vi "SentinelController v36.vi"() -> ()   [LabVIEW 2011]
uses:
  SC MT99XX tester states.ctl
  SC handler states.ctl
  Handler Types.ctl
  SC NS6040 tester states v2.ctl
  Echo tester states.ctl
  <vilib>/Instr/_visa.llb/Select Event Type.ctl
  <userlib>/configTool/configTool.llb/initConfigGlobal.vi
  <userlib>/configTool/configTool.llb/loadConfigFile.vi
  <userlib>/configTool/configTool.llb/closeConfig.vi
  <userlib>/configTool/configTool.llb/getProperty(DBL).vi
  <userlib>/configTool/configTool.llb/getProperty(U32).vi
  <userlib>/configTool/configTool.llb/getProperty(BOOL).vi
  <userlib>/configTool/configTool.llb/getProperty(I32).vi
  <userlib>/configTool/configTool.llb/getProperty(STR).vi
panel:
  out "Numeric 5":i32
  out "Numeric 4":i32
  out "Numeric 3":i32
  out "Numeric 2":i32
  out "Numeric":i32
  out "H2 wt start hidden":u32
  out "H2 wt end hidden":u32
  out "H2 it start hidden":u32
  out "H2 it end hidden":u32
  out "H2 tt start hidden":u32
  out "H2 tt end hidden":u32
  in  "Data log path and filename":path=path "configuraitons/default_configuraiton.cfg"
  in  "Panels":T1(tab)=enum."System Configuration"
  in  "Test cell ID":string="default"
  in  "Operator name":string="default"
  in  "Lot number":string="default"
  in  "Configuration file path and filename":path
  in  "POWER":bool=TRUE
  in  "Tester Handler Config":T2=enum."Seiko-Epson NS6040" caption="Handler type"
  in  "H1 handler type":T2=enum."Seiko-Epson NS6040" caption="Handler type"
  in  "H2 handler type":T2=enum."Seiko-Epson NS6040" caption="Handler type"
  in  "H2 allow lower parallelism":bool
  in  "H1 allow lower parallelism":bool
  in  "H1 low yield warning":dbl=95.0 min=0.0 max=100.0 step=1.0
  in  "Ignore alarms until AFTER this many cycles":i32=20
  in  "H1 low yield alarm":dbl=85.0 min=0.0 max=100.0 step=1.0
  in  "H1 low UPH warning (%)":dbl=95.0 min=1.0 max=48000.0 step=1.0
  in  "H1 low UPH alarm (%)":dbl=90.0 min=1.0 max=48000.0 step=1.0
  in  "Enable data logging of all events":bool=TRUE
  in  "Enable electronic notification of alarms":bool
  in  "H2 low UPH alarm (%)":dbl=90.0 min=1.0 max=48000.0 step=1.0
  in  "H2 low UPH warning (%)":dbl=95.0 min=1.0 max=48000.0 step=1.0
  in  "H2 low yield alarm":dbl=90.0 min=0.0 max=100.0 step=1.0
  in  "H2  low yield warning":dbl=95.0 min=0.0 max=100.0 step=1.0
  in  "H1 enable halt\non yield alarm":bool
  in  "H2 enable halt\non yield alarm":bool
  in  "H1 enable halt\non UPH alarm":bool
  in  "H2 enable halt\non UPH alarm":bool
  out "H2 Device Count":u32 caption="Device Count"
  out "H1 Device Count":u32 caption="Decvice Count"
  out "H1 Good Units":u32 caption="Decvice Count"
  out "H2 Good Units":u32 caption="Device Count"
  out "H1 lot yield mon":dbl format="%.1f"
  out "H2 lot yield mon":dbl format="%.1f"
  out "UPH averaging":u32=20 min=2 max=100 step=1
  out "Yield averaging":u32=20 min=2 max=100 step=1
  in  "Push to reset charts":bool
  in  "Run":bool caption="Run / Stop"
  in  "Optimize handler speed":bool
  out "H1 parallelism":u32
  out "Utilization averaging":i32=6 min=2 max=20 step=1
  out "H2 nominal 2":bool=TRUE
  out "H2 warning 2":bool
  out "H2 alarm 2":bool
  out "H1 nominal 2":bool=TRUE
  out "H1 warning 2":bool
  out "H1 alarm 2":bool
  out "H2 nominal":bool=TRUE
  out "H2 warning":bool
  out "H2 alarm":bool
  out "H1 nominal":bool=TRUE
  out "H1 warning":bool
  out "H1 alarm":bool
  out "H2 Lock":bool
  out "H1 Lock":bool
  out "H2 measured Test Time":dbl caption="Index Time" format="%.2f"
  out "H2 measured  Index Time":dbl caption="Index Time" format="%.2f"
  out "H2 Indexing":bool
  out "H2 Testing":bool
  out "H2 Waiting":bool
  out "H2 On/Off-line":bool
  out "H2 measured Wait Time":dbl caption="Index Time" format="%.2f"
  out "H1 measured Test Time":dbl caption="Index Time" format="%.2f"
  out "H1 measured Index Time":dbl caption="Index Time" format="%.2f"
  out "H1 Indexing":bool
  out "H1 Testing":bool
  out "H1 Waiting":bool
  out "H1 On/Off-line":bool
  out "H1 measured Wait Time":dbl caption="Index Time" format="%.2f"
  out "System UPH":u32(knob) caption="Sys UPH" scale=0.0..30240.0 scale format="%#.0f"
  out "H2 UPH":cluster{u32, u32}(knob) scale=0.0..14400.0 scale format="%#.0f"
  out "H1 UPH":cluster{u32, u32}(knob) scale=0.0..14400.0 scale format="%#.0f"
  out "Sys utilization":dbl(knob) caption="Yield" scale=0.0..100.0
  in  "H2 online":bool=TRUE
  in  "H1 online":bool=TRUE
  in  "Tester online":bool=TRUE
  in  "Alert volume":u32(knob)=5 max=10 step=1 scale=0.0..10.0
  in  "Audio On / Off":bool
  out "SysUtilMon":cluster{i32, i32}(graph)
  out "H2 parallelism":u32 caption="H2 Paralellism"
  out "YieldMon":cluster{i32, i32, i32, i32}(graph)
  out "Program Parallelism":u32=8 caption="Tester Parallelism" min=1 max=16 step=1
  out "H2 calc UPH":dbl format="%#.0f"
  out "H1 Index Time 2":dbl caption="H1 index time"
  out "H1 Test Time 2":dbl caption="H1 test time"
  out "H1 P in formula":u32 caption="H1 Parallelism"
  out "H2 UPH per unit area":dbl format="%.1f"
  out "H1 calc UPH":dbl format="%#.0f"
  out "H1 UPH per unit area":dbl format="%.1f"
  out "Std mo cost ($/mo)":dbl
  out "Std unit cost\n(cents/device)":dbl format="%.3g"
  out "UPH":dbl format="%#.0f"
  in  "Hours per month":i32=730
  out "Std hourly\ncost ($/hr)":dbl format="%.2f"
  in  "Std cell \nfloorspace area":i32=200 min=10 max=1000 step=10
  in  "Overhead ($/mo)":dbl=1000.0 min=0.0 max=10000.0 step=100.0
  in  "Handler cost ($/mo)":dbl=2500.0 min=0.0 max=100000.0 step=100.0
  in  "Tester cost ($/mo)":dbl=8500.0 min=0.0 max=100000.0 step=500.0
  in  "Utilization (%)":u32=80 min=10 max=100 step=10
  out "Calendar days required\nfor testing all units":dbl format="%.1f"
  in  "# of devices to test":u32=10000000 min=1000 max=100000000 step=1000
  out "$ saved":i64 format="%#.0f"
  out "H2 IT (scycle)":dbl format="%.2f"
  out "H2 TT (s/cycle)":dbl format="%.2f"
  out "H2 WT (s/cycle)":dbl format="%.2f"
  out "H1 WT (s/cycle)":dbl format="%.2f"
  out "H1 IT (s/cycle)":dbl format="%.2f"
  out "H1 TT (s/cycle)":dbl format="%.2f"
  out "H2 units/cycle":u32 caption="H1 Parallelism"
  out "H1 units/cycle":u32
  out "Calc H1 UPH":u32
  out "Calc H2 UPH":u32
  out "Std cell floorspace area":i32
  out "Tandem unit cost\n(cents/device)":dbl format="%.3f"
  out "Hours per month 2":i32 caption="Hours per month"
  out "Total Mo Costs ($/mo) 3":dbl caption="Tandem mo cost ($/mo)"
  out "Total Mo Costs ($/mo) 2":dbl caption="Std mo cost ($/mo)"
  out "Calc\nsystem UPH":u32 caption="Simulated\nSystem UPH"
  out "Tandem\nfloorspace area":i32
  out "Tandem UPH\nper unit area":dbl format="%.1f"
  in  "Second handler cost ($/mo)":dbl=2500.0 min=0.0 max=10000.0 step=100.0
  out "Tandem hourly\ncost ($/hr)":dbl format="%.2f"
  in  "Celerint licensing cost ($/mo)":dbl=1000.0 min=0.0 max=10000.0 step=100.0
  in  "Celerint hardware cost ($/mo)":dbl min=0.0 max=10000.0 step=1.0
  in  "Additional floorspace\nfor second handler":i32=50 min=0 max=1000 step=10
  out "Number of text alerts":u32 caption="Number of alerts\nsent as notifications"
  in  "Enable text notification":bool
  out "Notifications Lot Display":string="default" caption="Lot number (not editable)"
  in  "Include\ndata log as\nattachment":bool=TRUE
  out "Number of email alerts":u32 caption="Number of alerts\nsent as notifications"
  out "Email alert - attachment (not editable)":path
  in  "Email alert - message":string="An alarm event has ocurred on a semiconductor test lot that you have requested to monitor.  Please see the attached data log for event details.\n\nThis message is generated automatically by the Sentinel Controller program.\n\nTo stop these messages, please contact the test floor operator and disable automatic alert notifictions.\n\n"
  in  "Email alert - engineer":string="harry@celerint.com"
  in  "Email alert - CC":string="hjr@celerint.com"
  in  "Enable email notification":bool
  in  "Carrier":enum16{"T-Mobile", "AT&T", "Verizon", "Sprint"}(ring)=enum."AT&T"
  in  "Phone number":string="5128263411"
  in  "Subject":string="From: Sentinel Controller"
  in  "Body":string="An alarm event has ocurred"
  in  "GPIB wait time (ms)":u32=1000
  in  "Slow for  Diagnostics":bool=TRUE
  out "GPIB bus 0 read error":bool
  out "GPIB Bus 0 traffic":string
  out "GPIB bus 1 traffic":string
  out "GPIB bus 2 traffic":string
  out "GPIB bus 0 write error":bool
  out "GPIB bus 1 read error":bool
  out "GPIB bus 1 write error":bool
  out "GPIB bus 2 write error":bool
  out "GPIB bus 2 read error":bool
  out "VISA bus 1 open error":bool
  out "VISA bus 2 open error":bool
  out "VISA bus 0 open error":bool
  out "VISA bus 0 close error":bool
  out "VISA bus 1 close error":bool
  out "VISA bus 2 close error":bool
  out "Decrease Handler Velocity":string
  out "Increase Handler Velocity":string
  out "Get Handler Velocity":string
  in  "SentCtrl listens to tester at":refnum<visa-resource-name>="GPIB0::INTFC"
  out "H2 Address":string
  out "H1 Address":string
  out "Tester address":string
  in  "SentCtrl talks to tester at":refnum<visa-resource-name>="GPIB0::0::INSTR"
  in  "SentCtrl listens to handler 1 at":refnum<visa-resource-name>="GPIB1::INTFC"
  in  "SentCtrl talks to handler 1 at":refnum<visa-resource-name>="GPIB1::1::INSTR"
  in  "SentCtrl listens to handler 2 at":refnum<visa-resource-name>="GPIB2::INTFC"
  in  "SentCtrl talks to handler 2 at":refnum<visa-resource-name>="GPIB2::1::INSTR"
  in  "Ni Logo":bool
  in  "Ni Logo 2":bool
  out "H2 Ready with sites hid":bool
  in  "Echo state of tester hid":T3
  in  "SRQ MASK from tester hid":string
  in  "H1 binning string hid":string
  in  "H2 binning string hid":string
  in  "H1 FULLSITES? response hid":string
  in  "H2 FULLSITES? response hid":string
  in  "H1 FULLSITES? binary hid":string
  in  "H2 FULLSITES? binary hid":string
  in  "H1 response to SPOLL hid":string
  in  "H2 response to SPOLL hid":string
  in  "H1 response to FR? hid":string
  in  "H2 response to FR? hid":string
  in  "NS6040 tester states H1 hid":T4
  in  "NS6040 tester states H2 hid":T4
  in  "MT99XX tester states H2 hid":T5
  in  "MT99XX tester states H1 hid":T5
  in  "GPIB parsed msg from tester hid":string
  in  "Message from H2 hid":string
  in  "Message from H1 hid":string
  in  "Message from tester hid":string
  in  "H1 response to *IDN? hid":string
  in  "H2 response to *IDN? hid":string
  in  "GPIB wait timeout hid":u32
  out "Number of data log entries hid":u32
  in  "Last locked handler hid":enum16{"H1", "H2"}(ring)
  out "SC measured wait time hid":dbl
  out "Exit SC tester H2 StMach hid":bool
  out "Exit SC tester H1 StMach hid":bool
  out "Exit SC handler StMach hid":bool
  out "H2 response to *HAND? hid":string
  out "H1 response to *HAND? hid":string
  in  "Tester loop counter hid":u32
  in  "H2 loop counter hid":u32
  in  "H1 loop counter hid":u32
  in  "Test Cycle State hid":T6(ring)
  in  "Test time expected hid":dbl
  out "H1 it end hidden":u32
  out "H1 wt start hidden":u32
  out "H1 tt start hidden":u32
  out "H1 wt end hidden":u32
  out "H1 tt end hidden":u32
  out "H1 it start hidden":u32
  in  "H1 SITES? response hid":string
  out "VISA bus 1 resource name out hid":refnum<visa-resource-name>
  out "VISA bus 1 error out hid":errorcluster
  out "VISA bus 2 error out hid":errorcluster
  out "VISA bus 2 resource name out hid":refnum<visa-resource-name>
  out "VISA bus 0 error out hid":errorcluster
  out "tester wt start hid":u32
  out "tester wt end hid":u32
  out "tester tt start hid":u32
  out "tester tt end hid":u32
  out "SC measured test time hid":dbl
  in  "Binning string from tester hid":string
  out "VISA bus 0 resource name out hid":refnum<visa-resource-name>
  in  "SC handler states hid":T7
  out "H1 Single Handler UPH hid":dbl
  out "H1 UPH warning limit hid":dbl
  out "H1 UPH alarm limit hid":dbl
  out "H2 Single Handler UPH hid":dbl
  out "H2 UPH warning limit hid":dbl
  out "H2 UPH alarm limit hid":dbl
  in  "Min Test Time hid":dbl=0.499 caption="Min Test Time" min=0.1 max=1.0 step=0.1 format="%#.1g"
  in  "H2 index time expected hid":dbl
  in  "H1 index time expected hid":dbl
  in  "system states hid":T8(ring)
  in  "system statuts hid":T9(ring)
  out "H1 cycle yield hid":dbl format="%.1f"
  out "H2 cycle yield hid":dbl format="%.1f"
  in  "H2 SITES? response hid":string
  out "H1 Ready with sites hid":bool
  # "Sentinel Controller\nfor\nTandlem Handler\nTest Cells \nwww.celerint.com"
  # "Turning off POWER will stop execution the Sentinel Controller Program"
  # "INPUT FILE"
  # "LOT INFORMATION"
  # "Celerint Sentinel Controller"
  # "SYSTEM SETTINGS"
  # "Tester Handler Config"
  # "Handler  1"
  # "Handler 2"
  # "Set UPH thresholds as % of max UPH"
  # "Set UPH thresholds as % of max UPH"
  # "test cycles (insertions)"
  # "Celerint Sentinel Controller"
  # "Handler 2"
  # "Handler 1"
  # "Yield"
  # "UPH"
  # "Yield"
  # "UPH"
  # "parallelism"
  # "lot yield (%)"
  # "good devices"
  # "devices tested"
  # "Data"
  # "Avg"
  # "wait time"
  # "index time"
  # "test time"
  # "waiting"
  # "H1"
  # "H2"
  # "testing"
  # "indexing"
  # "on/off-line"
  # "STANDARD SETUP"
  # "H2 calculated\nsimilarly"
  # "3600"
  # "Celerint Sentinel\nController Simulator"
  # "TANDEM HANDLER SETUP"
  # "SAVINGS"
  # "3600 (s/hr)"
  # "3600 (s/hr)"
  # "Celerint Sentinel Controller"
  # "Lot number will be appended automatically:"
  # "This data is read from the INI file (.cfg)\nat program start and is used to configure\nthe various GPIB interfaces on the Sentinel\nController."
  # "These setting are created based on the addresses read from the INI file."
  # "Laptop Tester Sim\nGPIB0,SC\naddress 0\nlisten at: GPIB0::INTFC\ntalk to: GPIB0::1::INSTR"
  # "*SITES?"
  # "binning"
  # "Bus 0"
  # "1011"
  # "SC\nGPIB0,Non-SC\naddress 1\nlisten at: GPIB0::INTFC\ntalk to: GPIB0::0::INSTR"
  # "SC\nGPIB1,SC\naddress 0\nlisten at: GPIB1::INTFC\ntalk to: GPIB1::0::INSTR"
  # "SC\nGPIB2,SC\naddress 0\nlisten at: GPIB2::INTFC\ntalk to: GPIB2::0::INSTR"
  # "NI PXI-1031"
  # "*SITES?"
  # "binning"
  # "*SITES?"
  # "binning"
  # "Bus 1"
  # "Bus 2"
  # "1011"
  # "1011"
  # "Laptop H1 Sim\nGPIB1,Non-SC\naddress 1\nlisten at: GPIB1::INTFC\ntalk to: GPIB1::0::INSTR"
  # "Laptop H2 Sim\nGPIB2,Non-SC\naddress 1\nlisten at: GPIB2::INTFC\ntalk to: GPIB2::0::INSTR"
  # "Note:\nUsually, there are default GPIB addresses used for the tester and handler.\nThese addresses are read in from the INI file (.cfrg extension) when this\nprogram initializes.  For the purposes of this map, we are using  these defaults:\n          - Semiconductor tester default GPIB address: 6\n          - Semiconductor handler default GPIB address: 14\nFor the purposes of this illustration, these addresses are purely arbitrary."
  # "Tester\nGPIB0,SC\naddress 6\nlisten at: GPIB0::INTFC\ntalk to: GPIB0:14::INSTR"
  # "*SITES?"
  # "binning"
  # "Bus 0"
  # "1011"
  # "SC\nGPIB0,Non-SC\naddress 14\nlisten at: GPIB1::INTFC\ntalk to: GPIB1:6::INSTR"
  # "SC\nGPIB1,SC\naddress 6\nlisten at: GPIB1::INTFC\ntalk to: GPIB1:14::INSTR"
  # "SC\nGPIB2,SC\naddress 6\nlisten at: GPIB2::INTFC\ntalk to: GPIB2:14::INSTR"
  # "NI PXI-1031"
  # "*SITES?"
  # "binning"
  # "*SITES?"
  # "binning"
  # "Bus 1"
  # "Bus 2"
  # "1011"
  # "1011"
  # "Handler 1\nGPIB0,Non-SC\naddress 14\nlisten at: GPIB0::INTFC\ntalk to: GPIB0:6::INSTR"
  # "Handler 2\nGPIB0,Non-SC\naddress 14\nlisten at: GPIB0::INTFC\ntalk to: GPIB0:6::INSTR"
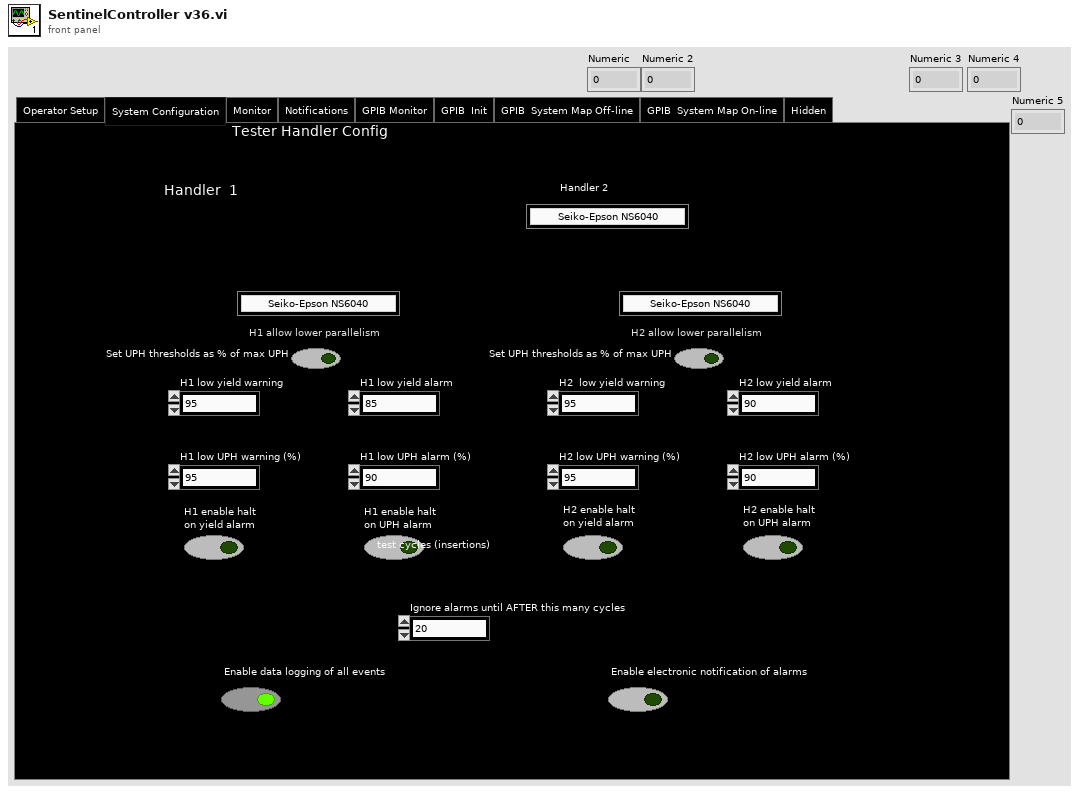
[diagram p1: front panel]
types:
  T1 = enum32{"Operator Setup", "System Configuration", "Monitor", "Benefit Analysis", "Notifications", "GPIB Monitor", "GPIB  Init", "GPIB  System Map Off-line", "GPIB  System Map On-line", "Hidden"}
  T2 = typedef "Handler Types.ctl" = enum16{"Multitest", "Seiko-Epson NS6040"}
  T3 = typedef "Echo tester states.ctl" = enum16{"ECHONG", "ECHOOK", "NO ECHO"}
  T4 = typedef "SC NS6040 tester states v2.ctl" = enum16{"initializing bus", "sending *IDN?", "serial polling handler", "sending Fullsites?", "testing", "binning", "closing bus"}
  T5 = typedef "SC MT99XX tester states.ctl" = enum16{"initializing bus", "polling *SITES?", "sending *IDN?", "testing", "binning", "closing bus"}
  T6 = enum16{"idled", "SOT received", "SOT sent", "binning sent", "binning received", "sites ready received", "sites ready sent"}
  T7 = typedef "SC handler states.ctl" = enum16{"initializing bus", "waiting on event", "waiting on serial poll", "reading", "responding to *IDN?", "responding to Fullsites?", "responding to SITES?", "responding to HIDN?", "respond to HAND?", "testing", "responding to BINON", "responding to A BIN", "ECHONG", "ECHOOK", "responding to unknown command", "closing bus"}
  T8 = enum16{"H1 Ready", "H2 Ready", "No Handler Ready"}
  T9 = enum16{"H1NH2N", "H1NH2W", "H1NH2A", "H1WH2N", "H1WH2W", "H1WH2A", "H1AH2N", "H1AH2W", "H1AH2A"}
  T10 = enum16{"open", "replace", "create", "open or create", "replace or create", "replace or create with confirmation"}
  T11 = typedef "configRef.ctl" = refnum<vi>
  T12 = cluster{i32, "rolling avg out":dbl, "H1 low yield alarm":dbl, "H2 low yield alarm":dbl}
  T13 = cluster{"rolling avg out":dbl, i32, "H1 low yield alarm":dbl, "H2 low yield alarm":dbl}
  T14 = typedef "Select Event Type.ctl" = u32
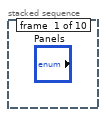
[diagram p2: hidden frame]
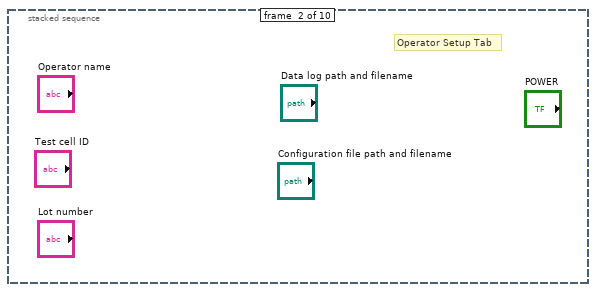
[diagram p3: hidden frame]
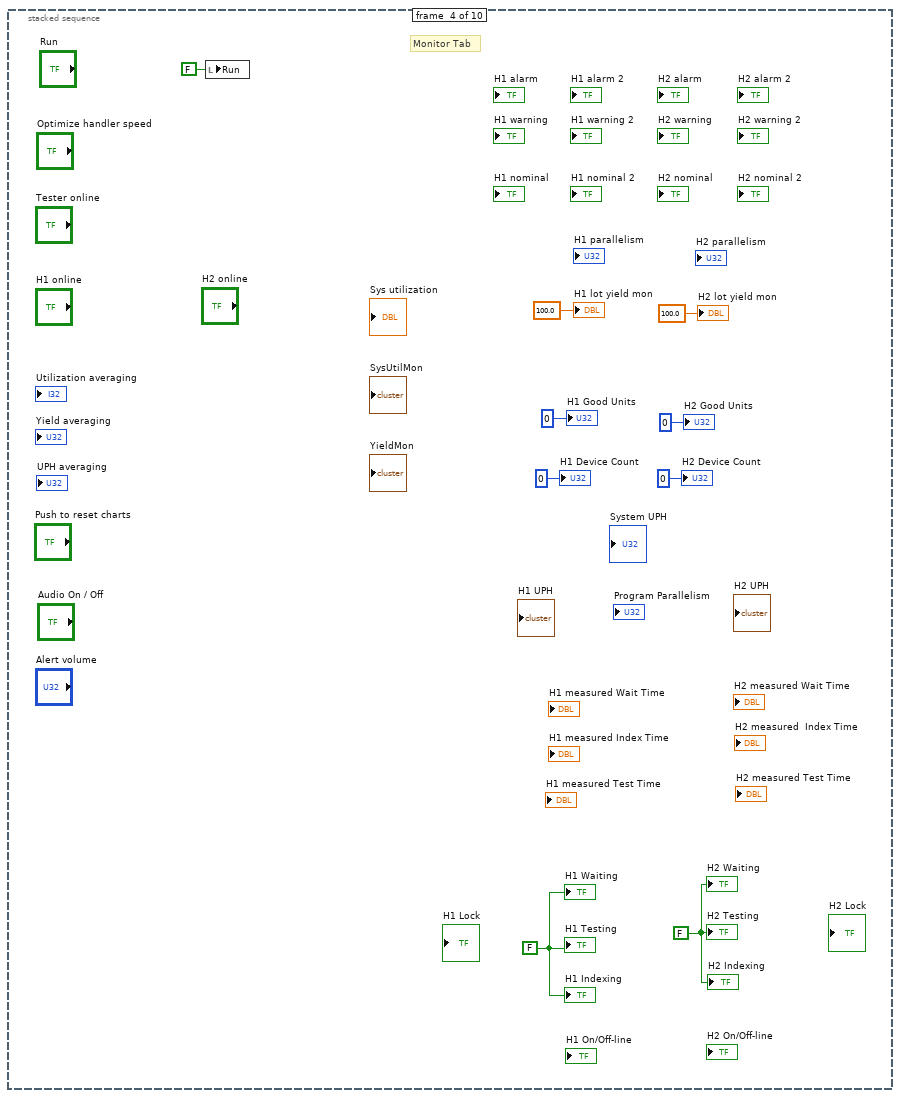
[diagram p4: hidden frame]
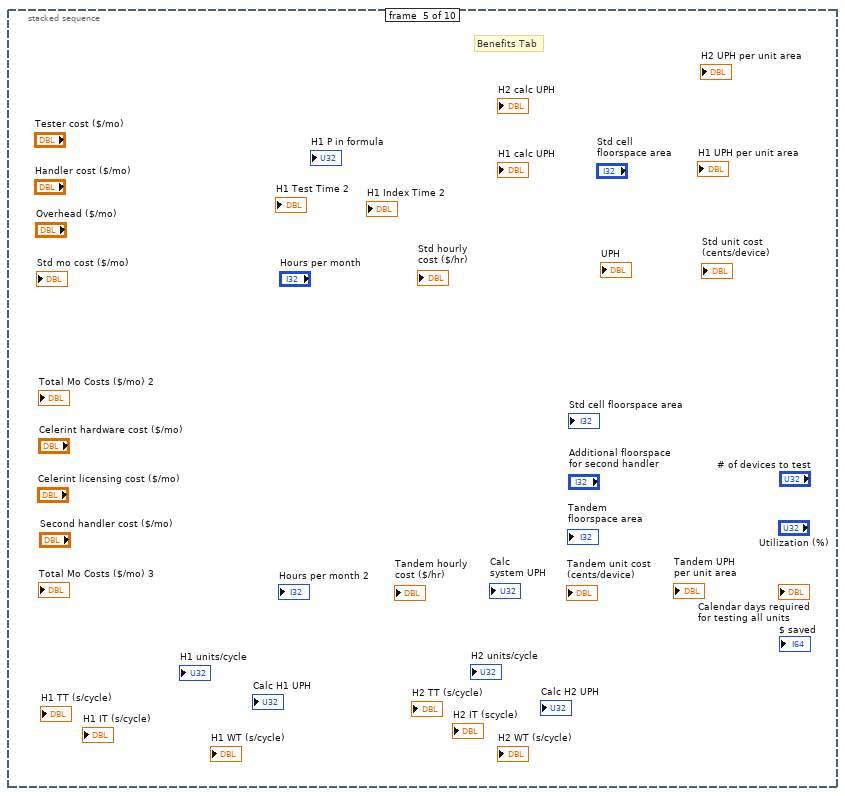
[diagram p5: hidden frame]
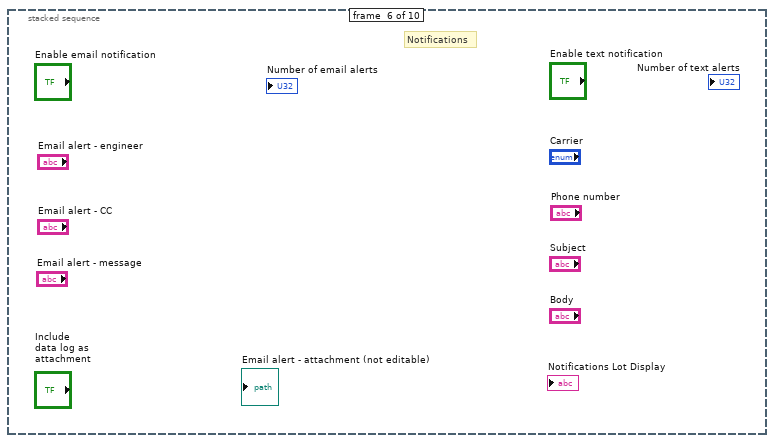
[diagram p6: hidden frame]
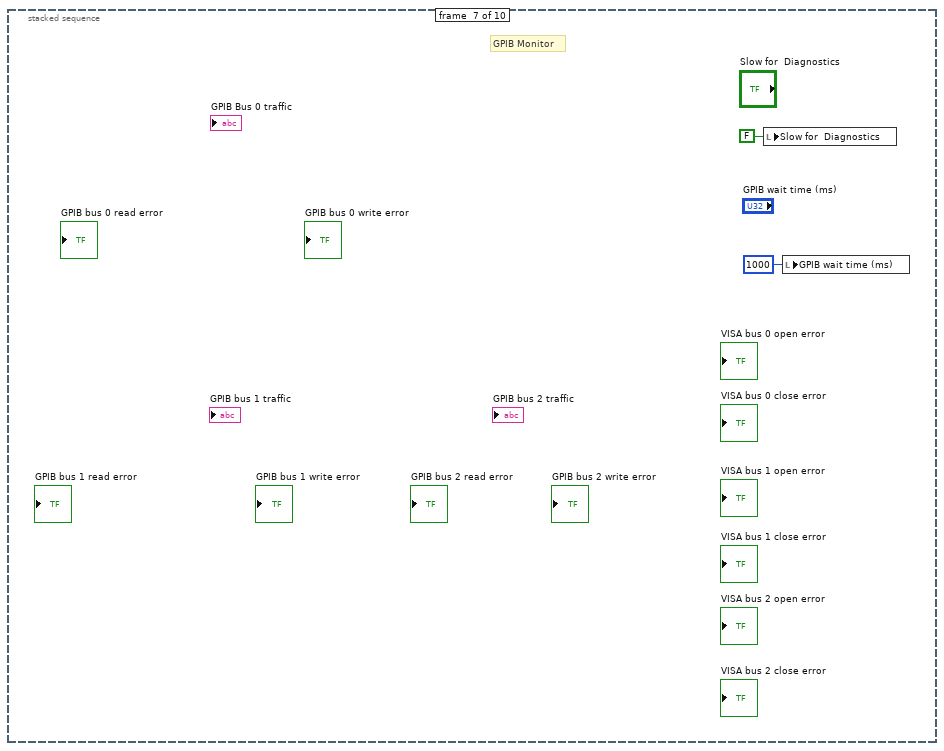
[diagram p7: hidden frame]
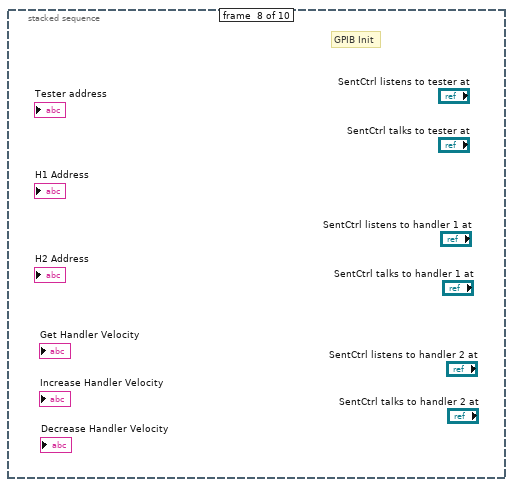
[diagram p8: hidden frame]
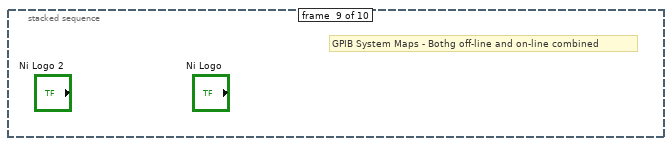
[diagram p9: hidden frame]
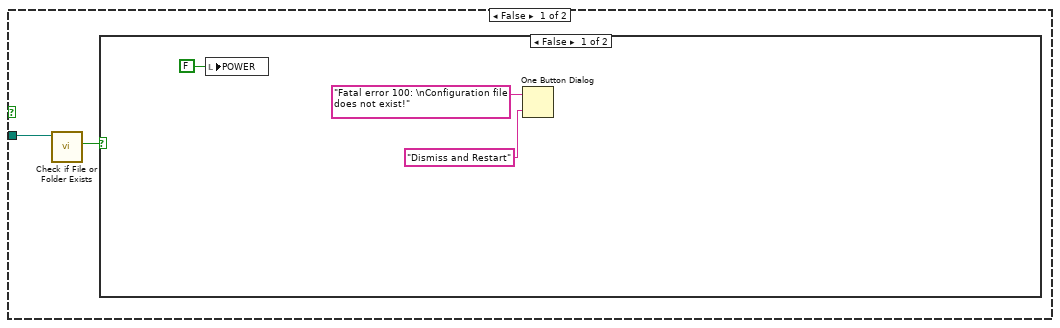
[diagram p11: hidden frame]
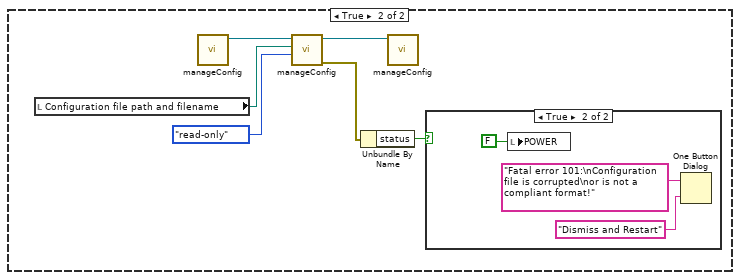
[diagram p12: hidden frame]
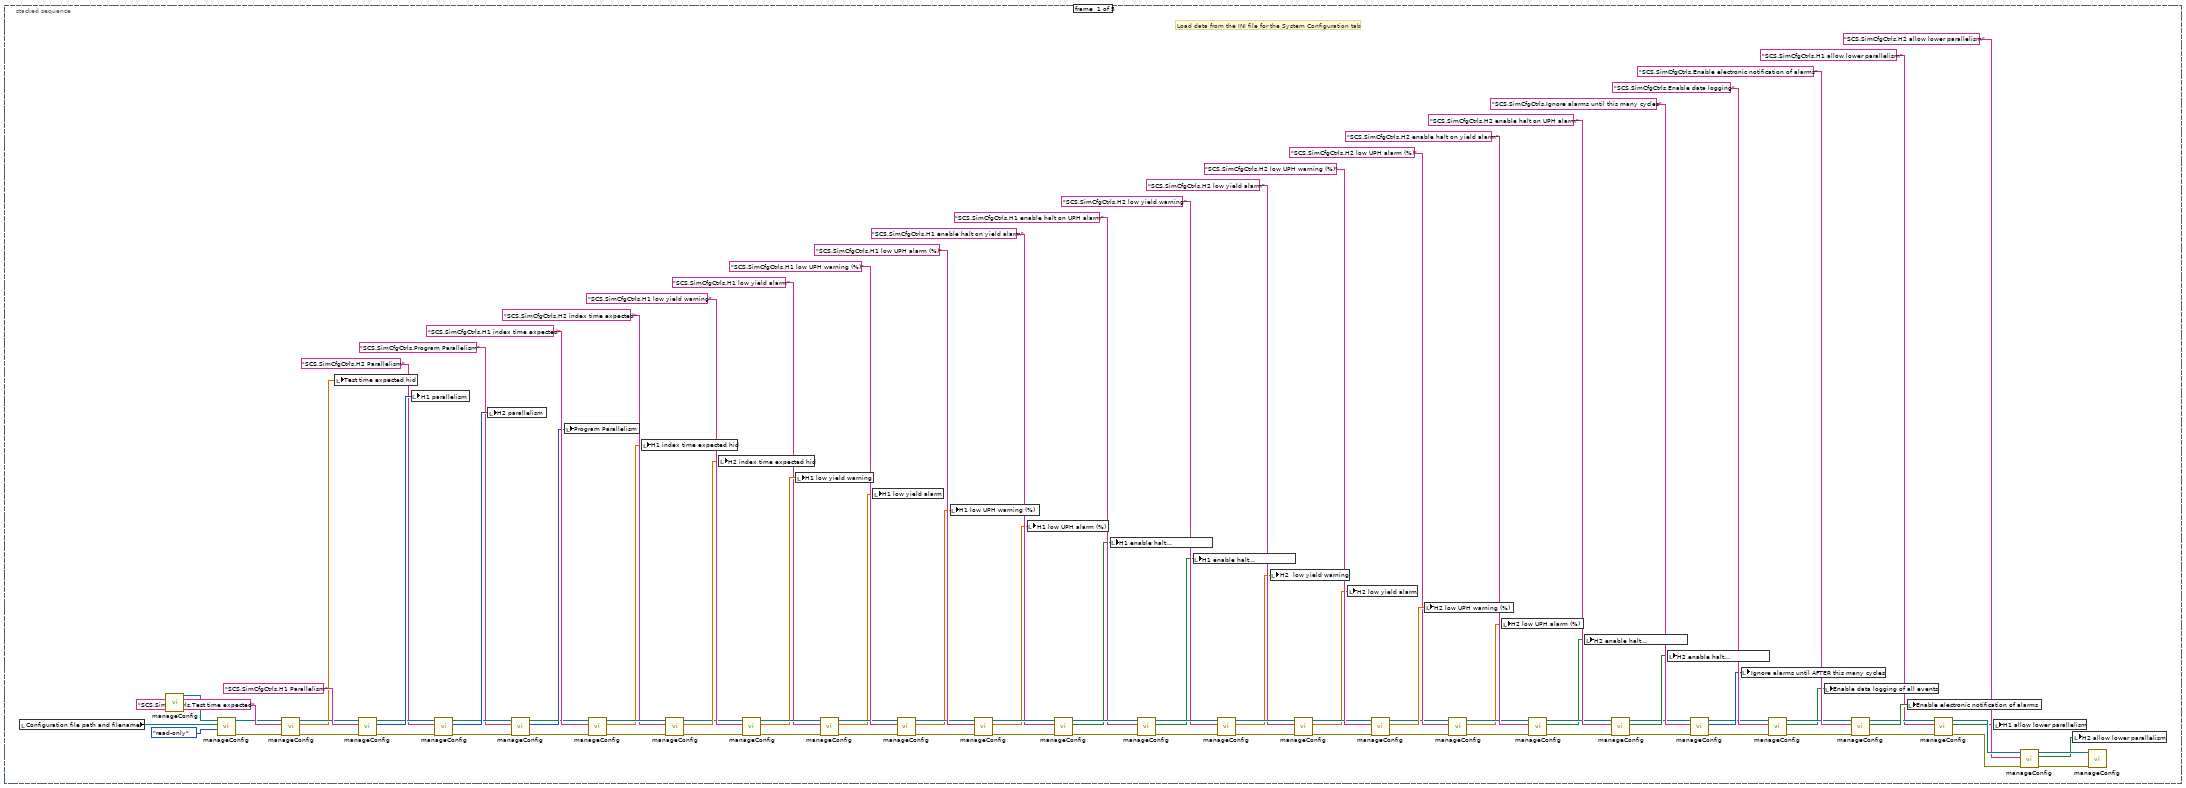
[diagram p15: hidden frame]
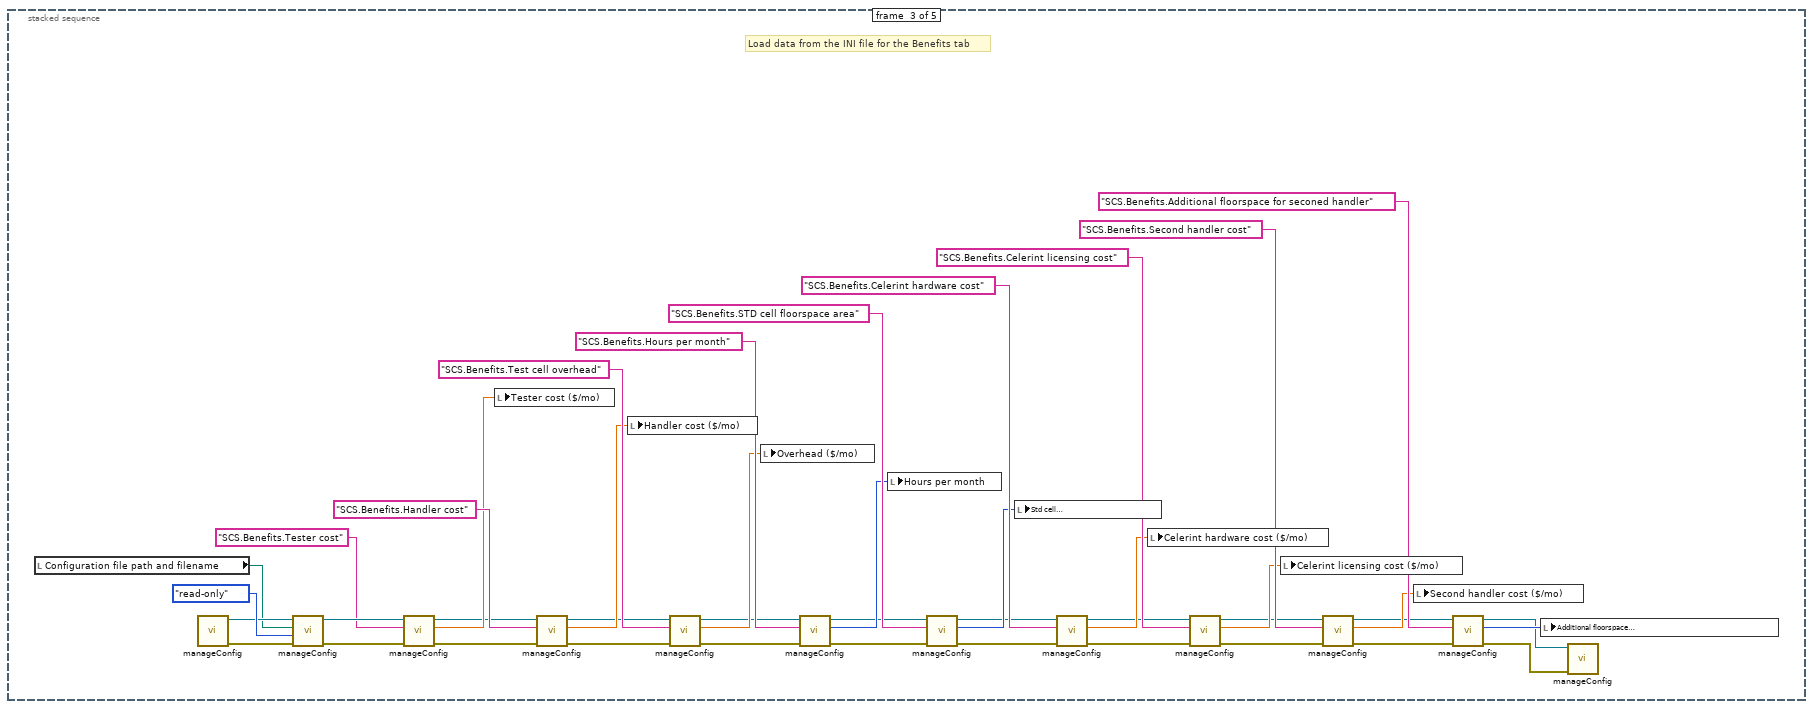
[diagram p16: hidden frame]
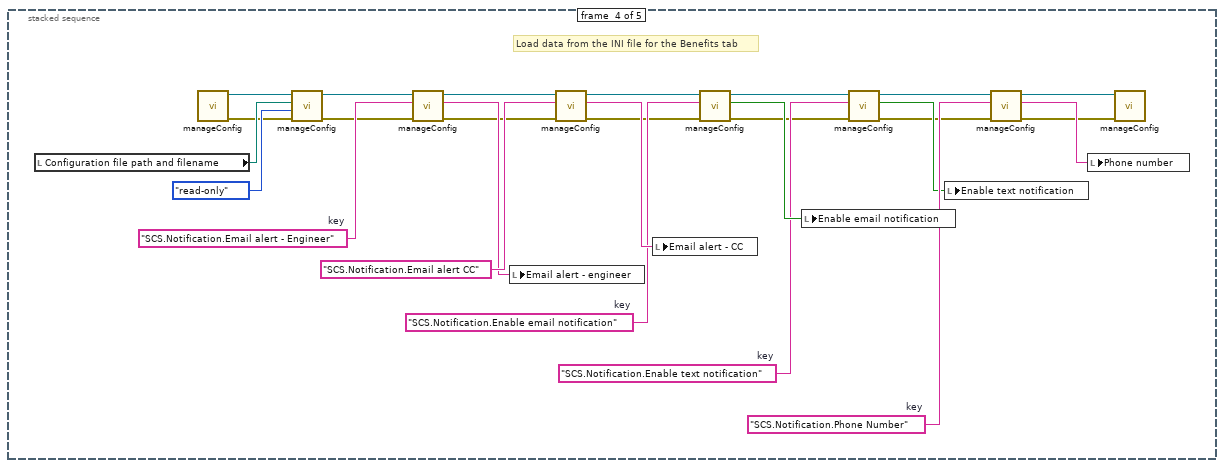
[diagram p17: hidden frame]
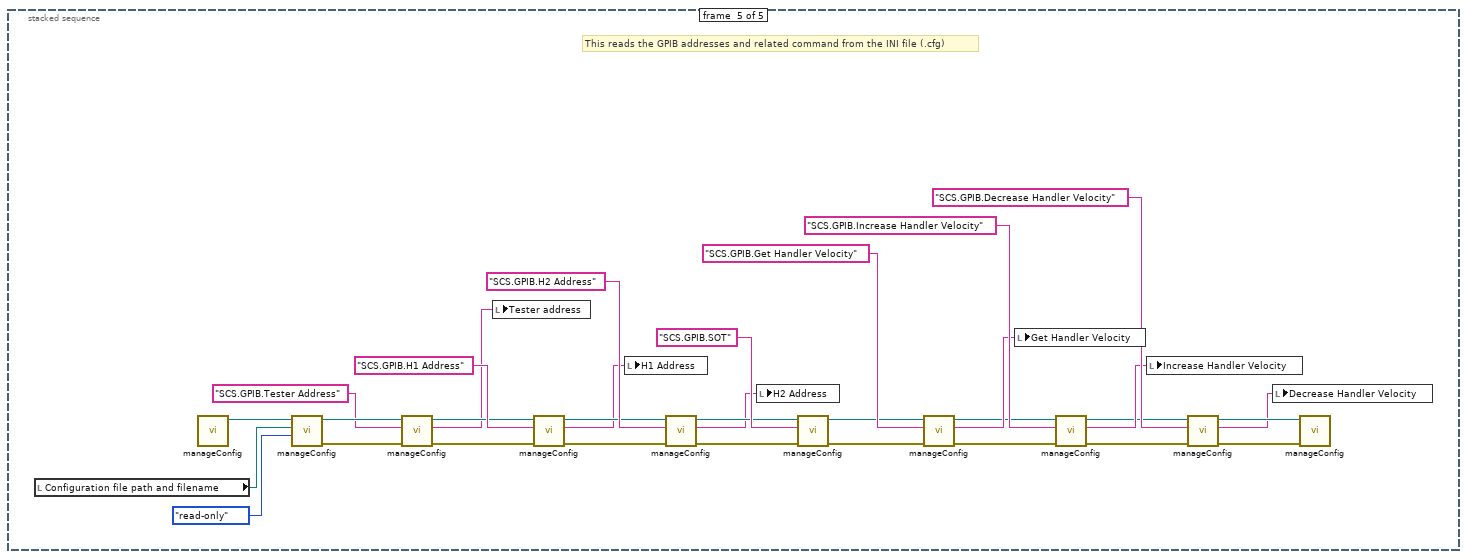
[diagram p18: hidden frame]
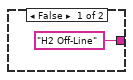
[diagram p20: hidden frame]
diagram:
  n1 = flat-sequence {
    frame #0 {
      # "This frame contains ALL declarations for control and indicators.\nAll hidden objects are on frame #9.  On the front panel, these hidden\nobjects are located on a tab that is hidden."
      n2 = stacked-sequence {
        frame #0 {
        }
        frame #1 {
          # "Operator Setup Tab"
        }
        frame #2 {
          # "System Config Tab"
        }
        frame #3 {
          w2 = FALSE ("H2 Testing")
          w1 = FALSE ("H1 Testing")
          # "Monitor Tab"
          n3 = local write "Run"(FALSE ("Run")) -> ()
          "H1 Testing" <- w1
          "H1 Waiting" <- w1
          "H1 Indexing" <- w1
          "H2 Testing" <- w2
          "H2 Waiting" <- w2
          "H2 Indexing" <- w2
          "H2 Good Units" <- 0
          "H2 Device Count" <- 0
          "H2 lot yield mon" <- 100.0 ("H2 Yield  Mon")
          "H1 lot yield mon" <- 100.0 ("H1 Yield Mon")
          "H1 Good Units" <- u32 0
          "H1 Device Count" <- u32 0
        }
        frame #4 {
          # "Benefits Tab"
        }
        frame #5 {
          # "Notifications"
        }
        frame #6 {
          # "GPIB Monitor"
          n4 = local write "Slow for  Diagnostics"(FALSE ("Slow for  Diagnostics")) -> ()
          n5 = local write "GPIB wait time (ms)"(u32 1000 ("GPIB wait time (ms)")) -> ()
        }
        frame #7 {
          # "GPIB Init"
        }
        frame #8 {
          # "GPIB System Maps - Bothg off-line and on-line combined"
        }
        frame #9 {
          (unwired) 0.031 ("tester measured wait time")
          # "Hidden controls and indicators"
          n6 = local write "Last locked handler hid"(enum16{"H1", "H2"}."H1" ("Last locked handler")) -> ()
          "SC measured test time hid" <- 1.0 ("tester measured test time")
          "H1 response to *HAND? hid" <- "" ("H1 response to *HAND? hidden")
          "H2 response to *HAND? hid" <- "" ("H2 response to *HAND? hidden")
          "Exit SC handler StMach hid" <- FALSE ("Exit tester state machine")
          "Exit SC tester H1 StMach hid" <- FALSE ("Exit H1 state machine")
          "Exit SC tester H2 StMach hid" <- FALSE ("Exit H2 state machine")
          "SC measured wait time hid" <- 1.0 ("tester measured wait time hid")
          "H2 cycle yield hid" <- 100.0 ("H2 Yield  Mon")
          "H1 cycle yield hid" <- 100.0 ("H1 Yield Mon")
        }
      }
    }
    frame #1 {
      n7 = local write "POWER"(TRUE ("POWER")) -> ()
    }
    frame #2 {
      # "This frame handles verifying that the configuration file exists and is valaid.\nIt also creates the data log."
      n8 = local read "Configuration file path and filename"() -> (w25:path)
      n9 = call <vilib>:"Application Directory.vi"() -> ("Application Directory"=w27:path)
      n10 = Equal?(x=w25, y=path "") -> (x = y?=w24:bool)
      n11 = Get Date/Time String(want seconds? (F)=TRUE) -> (date string=w40:string, time string=w32:string)  [unwired: 2 in]
      n12 = Build Path(base path=w27, name or relative path="datalogs") -> (appended path=w45:path)
      n13 = Path To String(path=w45) -> (string=w36:string)
      n14 = Search and Replace String(replace all?=TRUE ("replace all? (F)"), input string=w40, search string="/", replace string="-" ("replace string (\"\")")) -> (result string=w30:string)  [unwired: 4 in, 3 out]
      n15 = Search and Replace String(replace all?=TRUE ("replace all? (F)"), input string=w32, search string=":", replace string="." ("replace string (\"\")")) -> (result string=w31:string)  [unwired: 4 in, 3 out]
      n16 = case shown="True" w24 {
        tunnel: w25 -> [w47 _]
        frame False {
          n17 = call <vilib>:"Check if File or Folder Exists.vi"("path"=w47) -> ("file or folder exists?"=w46:bool)  [unwired: 8 in, 2 out]
          n18 = case shown="False" w46 {
            frame False {
              n19 = local write "POWER"(FALSE ("POWER")) -> ()
              n20 = One Button Dialog(message="Fatal error 100: \nConfiguration file does not exist!", button name ("OK")="Dismiss and Restart") -> ()  [unwired: 1 out]
            }
            frame True {
              n21 = local read "Configuration file path and filename"() -> (w54:path)
              n22 = call-poly <userlib>:"manageConfig.vi"() -> ("config ref out"=w55:T11)  [unwired: 10 in, 1 out]
              n23 = call-poly <userlib>:"manageConfig.vi"("access (0:read/write)"=enum16{"read/write", "read-only", "write-only"}."read-only", "config file path"=w54, "config ref"=w55) -> ("error out"=w53:errorcluster, "config ref out"=w51:T11)  [unwired: 6 in, 1 out]
              n24 = Unbundle By Name(w53) -> ("status"=w52:bool)
              n25 = call-poly <userlib>:"manageConfig.vi"("config ref"=w51) -> ()  [unwired: 10 in, 1 out]
              n26 = case shown="True" w52 {
                frame False {
                }
                frame True {
                  n27 = local write "POWER"(FALSE ("POWER")) -> ()
                  n28 = One Button Dialog(message="Fatal error 101:\nConfiguration file is corrupted\nor is not a compliant format!", button name ("OK")="Dismiss and Restart") -> ()  [unwired: 1 out]
                }
              }
            }
          }
        }
        frame True {
          n29 = call <vilib>:"Application Directory.vi"() -> ("Application Directory"=w63:path)
          n30 = Build Path(base path=w63, name or relative path="configurations") -> (appended path=w60:path)
          n31 = Path To String(path=w60) -> (string=w65:string)
          n32 = Concatenate Strings(w65, "\\" ("string"), "default_configuration.cfg" ("string")) -> (w66:string)
          n33 = String To Path(string=w66) -> (path=w67:path)
          n34 = local write "Configuration file path and filename"(w67) -> ()
        }
      }
      n35 = Concatenate Strings(w36, "\\" ("string"), w30, " " ("string"), w31, ".txt" ("string")) -> (w42:string)
      n36 = String To Path(string=w42) -> (path=w44:path)
      n37 = local write "Data log path and filename"(w44) -> ()
    }
    frame #3 {
      # "This frame reads the INI file and initializes all data that is under engineering control."
      n38 = local read "POWER"() -> (w68:bool)
      n39 = case shown="True" w68 {
        frame False {
        }
        frame True {
          n40 = stacked-sequence {
            frame #0 {
              # "Load data from the INI file for the System Configuration tab"
              n41 = local read "Configuration file path and filename"() -> (w162:path)
              n42 = call-poly <userlib>:"manageConfig.vi"() -> ("config ref out"=w163:T11)  [unwired: 10 in, 1 out]
              n43 = call-poly <userlib>:"manageConfig.vi"("access (0:read/write)"=enum16{"read/write", "read-only", "write-only"}."read-only", "config file path"=w162, "config ref"=w163) -> ("error out"=w101:errorcluster, "config ref out"=w100:T11)  [unwired: 6 in, 1 out]
              n44 = call-poly <userlib>:"manageConfig.vi"("error in"=w101, "property path"="SCS.SimCfgCtrls.Test time expected" ("key"), "config ref"=w100) -> ("error out"=w97:errorcluster, "data"=w103:dbl, "config ref out"=w104:T11)  [unwired: 5 in, 1 out]
              n45 = local write "Test time expected hid"(w103) -> ()
              n46 = call-poly <userlib>:"manageConfig.vi"("error in"=w97, "property path"="SCS.SimCfgCtrls.H1 Parallelism", "config ref"=w104) -> ("error out"=w96:errorcluster, "value"=w116:u32, "config ref out"=w110:T11)  [unwired: 5 in, 1 out]
              n47 = local write "H1 parallelism"(w116) -> ()
              n48 = call-poly <userlib>:"manageConfig.vi"("error in"=w96, "property path"="SCS.SimCfgCtrls.H2 Parallelism", "config ref"=w110) -> ("error out"=w95:errorcluster, "value"=w112:u32, "config ref out"=w109:T11)  [unwired: 5 in, 1 out]
              n49 = local write "H2 parallelism"(w112) -> ()
              n50 = call-poly <userlib>:"manageConfig.vi"("error in"=w95, "property path"="SCS.SimCfgCtrls.Program Parallelism", "config ref"=w109) -> ("error out"=w94:errorcluster, "value"=w111:u32, "config ref out"=w102:T11)  [unwired: 5 in, 1 out]
              n51 = local write "Program Parallelism"(w111) -> ()
              n52 = call-poly <userlib>:"manageConfig.vi"("error in"=w94, "property path"="SCS.SimCfgCtrls.H1 index time expected", "config ref"=w102) -> ("error out"=w93:errorcluster, "data"=w106:dbl, "config ref out"=w115:T11)  [unwired: 5 in, 1 out]
              n53 = local write "H1 index time expected hid"(w106) -> ()
              n54 = call-poly <userlib>:"manageConfig.vi"("error in"=w93, "property path"="SCS.SimCfgCtrls.H2 index time expected", "config ref"=w115) -> ("error out"=w99:errorcluster, "data"=w105:dbl, "config ref out"=w98:T11)  [unwired: 5 in, 1 out]
              n55 = local write "H2 index time expected hid"(w105) -> ()
              n56 = call-poly <userlib>:"manageConfig.vi"("error in"=w99, "property path"="SCS.SimCfgCtrls.H1 low yield warning" ("key"), "config ref"=w98) -> ("error out"=w92:errorcluster, "data"=w139:dbl, "config ref out"=w149:T11)  [unwired: 5 in, 1 out]
              n57 = local write "H1 low yield warning"(w139) -> ()
              n58 = call-poly <userlib>:"manageConfig.vi"("error in"=w92, "property path"="SCS.SimCfgCtrls.H1 low yield alarm", "config ref"=w149) -> ("error out"=w91:errorcluster, "data"=w138:dbl, "config ref out"=w148:T11)  [unwired: 5 in, 1 out]
              n59 = local write "H1 low yield alarm"(w138) -> ()
              n60 = call-poly <userlib>:"manageConfig.vi"("error in"=w91, "property path"="SCS.SimCfgCtrls.H1 low UPH warning (%)", "config ref"=w148) -> ("error out"=w90:errorcluster, "data"=w137:dbl, "config ref out"=w150:T11)  [unwired: 5 in, 1 out]
              n61 = local write "H1 low UPH warning (%)"(w137) -> ()
              n62 = call-poly <userlib>:"manageConfig.vi"("error in"=w90, "property path"="SCS.SimCfgCtrls.H1 low UPH alarm (%)", "config ref"=w150) -> ("error out"=w89:errorcluster, "data"=w136:dbl, "config ref out"=w151:T11)  [unwired: 5 in, 1 out]
              n63 = local write "H1 low UPH alarm (%)"(w136) -> ()
              n64 = call-poly <userlib>:"manageConfig.vi"("error in"=w89, "property path"="SCS.SimCfgCtrls.H1 enable halt on yield alarm", "config ref"=w151) -> ("error out"=w88:errorcluster, "value"=w135:bool, "config ref out"=w152:T11)  [unwired: 5 in, 1 out]
              n65 = local write "H1 enable halt\non yield alarm"(w135) -> ()
              n66 = call-poly <userlib>:"manageConfig.vi"("error in"=w88, "property path"="SCS.SimCfgCtrls.H1 enable halt on UPH alarm", "config ref"=w152) -> ("error out"=w87:errorcluster, "value"=w134:bool, "config ref out"=w153:T11)  [unwired: 5 in, 1 out]
              n67 = local write "H1 enable halt\non UPH alarm"(w134) -> ()
              n68 = call-poly <userlib>:"manageConfig.vi"("error in"=w87, "property path"="SCS.SimCfgCtrls.H2 low yield warning", "config ref"=w153) -> ("error out"=w86:errorcluster, "data"=w133:dbl, "config ref out"=w154:T11)  [unwired: 5 in, 1 out]
              n69 = local write "H2  low yield warning"(w133) -> ()
              n70 = call-poly <userlib>:"manageConfig.vi"("error in"=w86, "property path"="SCS.SimCfgCtrls.H2 low yield alarm", "config ref"=w154) -> ("error out"=w85:errorcluster, "data"=w132:dbl, "config ref out"=w155:T11)  [unwired: 5 in, 1 out]
              n71 = local write "H2 low yield alarm"(w132) -> ()
              n72 = call-poly <userlib>:"manageConfig.vi"("error in"=w85, "property path"="SCS.SimCfgCtrls.H2 low UPH warning (%)", "config ref"=w155) -> ("error out"=w84:errorcluster, "data"=w131:dbl, "config ref out"=w123:T11)  [unwired: 5 in, 1 out]
              n73 = local write "H2 low UPH warning (%)"(w131) -> ()
              n74 = call-poly <userlib>:"manageConfig.vi"("error in"=w84, "property path"="SCS.SimCfgCtrls.H2 low UPH alarm (%)", "config ref"=w123) -> ("error out"=w83:errorcluster, "data"=w121:dbl, "config ref out"=w122:T11)  [unwired: 5 in, 1 out]
              n75 = local write "H2 low UPH alarm (%)"(w121) -> ()
              n76 = call-poly <userlib>:"manageConfig.vi"("error in"=w83, "property path"="SCS.SimCfgCtrls.H2 enable halt on yield alarm", "config ref"=w122) -> ("error out"=w82:errorcluster, "value"=w130:bool, "config ref out"=w156:T11)  [unwired: 5 in, 1 out]
              n77 = local write "H2 enable halt\non yield alarm"(w130) -> ()
              n78 = call-poly <userlib>:"manageConfig.vi"("error in"=w82, "property path"="SCS.SimCfgCtrls.H2 enable halt on UPH alarm", "config ref"=w156) -> ("error out"=w81:errorcluster, "value"=w129:bool, "config ref out"=w120:T11)  [unwired: 5 in, 1 out]
              n79 = local write "H2 enable halt\non UPH alarm"(w129) -> ()
              n80 = call-poly <userlib>:"manageConfig.vi"("error in"=w81, "property path"="SCS.SimCfgCtrls.Ignore alarms until this many cycles", "config ref"=w120) -> ("error out"=w80:errorcluster, "value"=w128:i32, "config ref out"=w119:T11)  [unwired: 5 in, 1 out]
              n81 = local write "Ignore alarms until AFTER this many cycles"(w128) -> ()
              n82 = call-poly <userlib>:"manageConfig.vi"("error in"=w80, "property path"="SCS.SimCfgCtrls.Enable data logging", "config ref"=w119) -> ("error out"=w79:errorcluster, "value"=w127:bool, "config ref out"=w140:T11)  [unwired: 5 in, 1 out]
              n83 = local write "Enable data logging of all events"(w127) -> ()
              n84 = call-poly <userlib>:"manageConfig.vi"("error in"=w79, "property path"="SCS.SimCfgCtrls.Enable electronic notification of alarms", "config ref"=w140) -> ("error out"=w78:errorcluster, "value"=w126:bool, "config ref out"=w76:T11)  [unwired: 5 in, 1 out]
              n85 = local write "Enable electronic notification of alarms"(w126) -> ()
              n86 = call-poly <userlib>:"manageConfig.vi"("error in"=w78, "property path"="SCS.SimCfgCtrls.H1 allow lower parallelism", "config ref"=w76) -> ("error out"=w77:errorcluster, "value"=w70:bool, "config ref out"=w75:T11)  [unwired: 5 in, 1 out]
              n87 = local write "H1 allow lower parallelism"(w70) -> ()
              n88 = call-poly <userlib>:"manageConfig.vi"("error in"=w77, "property path"="SCS.SimCfgCtrls.H2 allow lower parallelism", "config ref"=w75) -> ("error out"=w73:errorcluster, "value"=w69:bool, "config ref out"=w74:T11)  [unwired: 5 in, 1 out]
              n89 = local write "H2 allow lower parallelism"(w69) -> ()
              n90 = call-poly <userlib>:"manageConfig.vi"("error in (no error)"=w73, "config ref"=w74) -> ()  [unwired: 9 in, 1 out]
            }
            frame #1 {
              # "Load data from the INI file for the Monitor tab"
              n91 = local read "Configuration file path and filename"() -> (w201:path)
              n92 = call-poly <userlib>:"manageConfig.vi"() -> ("error out"=w175:errorcluster, "config ref out"=w202:T11)  [unwired: 10 in]
              n93 = call-poly <userlib>:"manageConfig.vi"("error in (no error)"=w175, "access (0:read/write)"=enum16{"read/write", "read-only", "write-only"}."read-only", "config file path"=w201, "config ref"=w202) -> ("error out"=w204:errorcluster, "config ref out"=w206:T11)  [unwired: 5 in, 1 out]
              n94 = call-poly <userlib>:"manageConfig.vi"("error in"=w204, "property path"="SCS.Monitor.Optimize handler speed" ("key"), "config ref"=w206) -> ("error out"=w174:errorcluster, "value"=w184:bool, "config ref out"=w176:T11)  [unwired: 5 in, 1 out]
              n95 = local write "Optimize handler speed"(w184) -> ()
              n96 = call-poly <userlib>:"manageConfig.vi"("error in"=w174, "property path"="SCS.Monitor.Tester on-line" ("key"), "config ref"=w176) -> ("error out"=w173:errorcluster, "value"=w183:bool, "config ref out"=w197:T11)  [unwired: 5 in, 1 out]
              n97 = local write "Tester online"(w183) -> ()
              n98 = call-poly <userlib>:"manageConfig.vi"("error in"=w173, "property path"="SCS.Monitor.H1 on-line" ("key"), "config ref"=w197) -> ("error out"=w172:errorcluster, "value"=w182:bool, "config ref out"=w196:T11)  [unwired: 5 in, 1 out]
              n99 = local write "H1 online"(w182) -> ()
              n100 = call-poly <userlib>:"manageConfig.vi"("error in"=w172, "property path"="SCS.Monitor.H2 on-line" ("key"), "config ref"=w196) -> ("error out"=w171:errorcluster, "value"=w181:bool, "config ref out"=w195:T11)  [unwired: 5 in, 1 out]
              n101 = local write "H2 online"(w181) -> ()
              n102 = call-poly <userlib>:"manageConfig.vi"("error in"=w171, "property path"="SCS.Monitor.Utilization averaging", "config ref"=w195) -> ("error out"=w170:errorcluster, "value"=w177:i32, "config ref out"=w194:T11)  [unwired: 5 in, 1 out]
              n103 = local write "Utilization averaging"(w177) -> ()
              n104 = call-poly <userlib>:"manageConfig.vi"("error in"=w170, "property path"="SCS.Monitor.Audio On/Off", "config ref"=w194) -> ("error out"=w169:errorcluster, "config ref out"=w193:T11)  [unwired: 5 in, 2 out]
              n105 = call-poly <userlib>:"manageConfig.vi"("error in"=w169, "property path"="SCS.Monitor.Alert volume", "config ref"=w193) -> ("error out"=w168:errorcluster, "value"=w180:u32, "config ref out"=w192:T11)  [unwired: 5 in, 1 out]
              n106 = local write "Alert volume"(w180) -> ()
              n107 = call-poly <userlib>:"manageConfig.vi"("error in"=w168, "property path"="SCS.Monitor.UPH averaging", "config ref"=w192) -> ("error out"=w167:errorcluster, "value"=w179:u32, "config ref out"=w191:T11)  [unwired: 5 in, 1 out]
              n108 = local write "UPH averaging"(w179) -> ()
              n109 = call-poly <userlib>:"manageConfig.vi"("error in"=w167, "property path"="SCS.Monitor.Yield averaging", "config ref"=w191) -> ("error out"=w166:errorcluster, "value"=w178:u32, "config ref out"=w190:T11)  [unwired: 5 in, 1 out]
              n110 = local write "Yield averaging"(w178) -> ()
              n111 = call-poly <userlib>:"manageConfig.vi"("error in (no error)"=w166, "config ref"=w190) -> ()  [unwired: 9 in, 1 out]
            }
            frame #2 {
              # "Load data from the INI file for the Benefits tab"
              n112 = local read "Configuration file path and filename"() -> (w243:path)
              n113 = call-poly <userlib>:"manageConfig.vi"() -> ("error out"=w216:errorcluster, "config ref out"=w244:T11)  [unwired: 10 in]
              n114 = call-poly <userlib>:"manageConfig.vi"("error in (no error)"=w216, "access (0:read/write)"=enum16{"read/write", "read-only", "write-only"}."read-only", "config file path"=w243, "config ref"=w244) -> ("error out"=w246:errorcluster, "config ref out"=w248:T11)  [unwired: 5 in, 1 out]
              n115 = call-poly <userlib>:"manageConfig.vi"("error in"=w246, "property path"="SCS.Benefits.Tester cost" ("key"), "config ref"=w248) -> ("error out"=w215:errorcluster, "data"=w234:dbl, "config ref out"=w225:T11)  [unwired: 5 in, 1 out]
              n116 = local write "Tester cost ($/mo)"(w234) -> ()
              n117 = call-poly <userlib>:"manageConfig.vi"("error in"=w215, "property path"="SCS.Benefits.Handler cost" ("key"), "config ref"=w225) -> ("error out"=w214:errorcluster, "data"=w233:dbl, "config ref out"=w224:T11)  [unwired: 5 in, 1 out]
              n118 = local write "Handler cost ($/mo)"(w233) -> ()
              n119 = call-poly <userlib>:"manageConfig.vi"("error in"=w214, "property path"="SCS.Benefits.Test cell overhead" ("key"), "config ref"=w224) -> ("error out"=w213:errorcluster, "data"=w232:dbl, "config ref out"=w223:T11)  [unwired: 5 in, 1 out]
              n120 = local write "Overhead ($/mo)"(w232) -> ()
              n121 = call-poly <userlib>:"manageConfig.vi"("error in"=w213, "property path"="SCS.Benefits.Hours per month" ("key"), "config ref"=w223) -> ("error out"=w212:errorcluster, "value"=w231:i32, "config ref out"=w222:T11)  [unwired: 5 in, 1 out]
              n122 = local write "Hours per month"(w231) -> ()
              n123 = call-poly <userlib>:"manageConfig.vi"("error in"=w212, "property path"="SCS.Benefits.STD cell floorspace area" ("key"), "config ref"=w222) -> ("error out"=w211:errorcluster, "value"=w230:i32, "config ref out"=w221:T11)  [unwired: 5 in, 1 out]
              n124 = local write "Std cell \nfloorspace area"(w230) -> ()
              n125 = call-poly <userlib>:"manageConfig.vi"("error in"=w211, "property path"="SCS.Benefits.Celerint hardware cost" ("key"), "config ref"=w221) -> ("error out"=w210:errorcluster, "data"=w229:dbl, "config ref out"=w220:T11)  [unwired: 5 in, 1 out]
              n126 = local write "Celerint hardware cost ($/mo)"(w229) -> ()
              n127 = call-poly <userlib>:"manageConfig.vi"("error in"=w210, "property path"="SCS.Benefits.Celerint licensing cost" ("key"), "config ref"=w220) -> ("error out"=w209:errorcluster, "data"=w228:dbl, "config ref out"=w219:T11)  [unwired: 5 in, 1 out]
              n128 = local write "Celerint licensing cost ($/mo)"(w228) -> ()
              n129 = call-poly <userlib>:"manageConfig.vi"("error in"=w209, "property path"="SCS.Benefits.Second handler cost" ("key"), "config ref"=w219) -> ("error out"=w208:errorcluster, "data"=w227:dbl, "config ref out"=w218:T11)  [unwired: 5 in, 1 out]
              n130 = local write "Second handler cost ($/mo)"(w227) -> ()
              n131 = call-poly <userlib>:"manageConfig.vi"("error in"=w208, "property path"="SCS.Benefits.Additional floorspace for seconed handler" ("key"), "config ref"=w218) -> ("error out"=w207:errorcluster, "value"=w226:i32, "config ref out"=w217:T11)  [unwired: 5 in, 1 out]
              n132 = local write "Additional floorspace\nfor second handler"(w226) -> ()
              n133 = call-poly <userlib>:"manageConfig.vi"("error in (no error)"=w207, "config ref"=w217) -> ()  [unwired: 9 in, 1 out]
            }
            frame #3 {
              w259 = "SCS.Notification.Enable text notification"  # key
              w265 = "SCS.Notification.Phone Number"  # key
              w266 = "SCS.Notification.Enable email notification"  # key
              w273 = "SCS.Notification.Email alert - Engineer"  # key
              # "Load data from the INI file for the Benefits tab"
              n134 = local read "Configuration file path and filename"() -> (w270:path)
              n135 = call-poly <userlib>:"manageConfig.vi"() -> ("error out"=w255:errorcluster, "config ref out"=w271:T11)  [unwired: 10 in]
              n136 = call-poly <userlib>:"manageConfig.vi"("error in (no error)"=w255, "access (0:read/write)"=enum16{"read/write", "read-only", "write-only"}."read-only", "config file path"=w270, "config ref"=w271) -> ("error out"=w254:errorcluster, "config ref out"=w274:T11)  [unwired: 5 in, 1 out]
              n137 = call-poly <userlib>:"manageConfig.vi"("error in"=w254, "property path"=w273, "config ref"=w274) -> ("error out"=w253:errorcluster, "value"=w268:string, "config ref out"=w264:T11)  [unwired: 5 in, 1 out]
              n138 = local write "Email alert - engineer"(w268) -> ()
              n139 = call-poly <userlib>:"manageConfig.vi"("error in"=w253, "property path"="SCS.Notification.Email alert CC", "config ref"=w264) -> ("error out"=w252:errorcluster, "value"=w267:string, "config ref out"=w263:T11)  [unwired: 5 in, 1 out]
              n140 = local write "Email alert - CC"(w267) -> ()
              n141 = call-poly <userlib>:"manageConfig.vi"("error in"=w252, "property path"=w266, "config ref"=w263) -> ("error out"=w251:errorcluster, "value"=w261:bool, "config ref out"=w258:T11)  [unwired: 5 in, 1 out]
              n142 = local write "Enable email notification"(w261) -> ()
              n143 = call-poly <userlib>:"manageConfig.vi"("error in"=w251, "property path"=w259, "config ref"=w258) -> ("error out"=w250:errorcluster, "value"=w256:bool, "config ref out"=w257:T11)  [unwired: 5 in, 1 out]
              n144 = local write "Enable text notification"(w256) -> ()
              n145 = call-poly <userlib>:"manageConfig.vi"("error in"=w250, "property path"=w265, "config ref"=w257) -> ("error out"=w249:errorcluster, "value"=w260:string, "config ref out"=w262:T11)  [unwired: 5 in, 1 out]
              n146 = local write "Phone number"(w260) -> ()
              n147 = call-poly <userlib>:"manageConfig.vi"("error in (no error)"=w249, "config ref"=w262) -> ()  [unwired: 9 in, 1 out]
            }
            frame #4 {
              # "This reads the GPIB addresses and related command from the INI file (.cfg)"
              n148 = local read "Configuration file path and filename"() -> (w301:path)
              n149 = call-poly <userlib>:"manageConfig.vi"() -> ("config ref out"=w302:T11)  [unwired: 10 in, 1 out]
              n150 = call-poly <userlib>:"manageConfig.vi"("access (0:read/write)"=enum16{"read/write", "read-only", "write-only"}."read-only", "config file path"=w301, "config ref"=w302) -> ("error out"=w304:errorcluster, "config ref out"=w306:T11)  [unwired: 6 in, 1 out]
              n151 = call-poly <userlib>:"manageConfig.vi"("error in"=w304, "property path"="SCS.GPIB.Tester Address" ("key"), "config ref"=w306) -> ("error out"=w291:errorcluster, "value"=w283:string, "config ref out"=w297:T11)  [unwired: 5 in, 1 out]
              n152 = local write "Tester address"(w283) -> ()
              n153 = call-poly <userlib>:"manageConfig.vi"("error in"=w291, "property path"="SCS.GPIB.H1 Address" ("key"), "config ref"=w297) -> ("error out"=w290:errorcluster, "value"=w282:string, "config ref out"=w296:T11)  [unwired: 5 in, 1 out]
              n154 = local write "H1 Address"(w282) -> ()
              n155 = call-poly <userlib>:"manageConfig.vi"("error in"=w290, "property path"="SCS.GPIB.H2 Address" ("key"), "config ref"=w296) -> ("error out"=w289:errorcluster, "value"=w281:string, "config ref out"=w295:T11)  [unwired: 5 in, 1 out]
              n156 = local write "H2 Address"(w281) -> ()
              n157 = call-poly <userlib>:"manageConfig.vi"("error in"=w289, "property path"="SCS.GPIB.SOT" ("key"), "config ref"=w295) -> ("error out"=w288:errorcluster, "config ref out"=w277:T11)  [unwired: 5 in, 2 out]
              n158 = call-poly <userlib>:"manageConfig.vi"("error in"=w288, "property path"="SCS.GPIB.Get Handler Velocity" ("key"), "config ref"=w277) -> ("error out"=w287:errorcluster, "value"=w280:string, "config ref out"=w276:T11)  [unwired: 5 in, 1 out]
              n159 = local write "Get Handler Velocity"(w280) -> ()
              n160 = call-poly <userlib>:"manageConfig.vi"("error in"=w287, "property path"="SCS.GPIB.Increase Handler Velocity" ("key"), "config ref"=w276) -> ("error out"=w286:errorcluster, "value"=w279:string, "config ref out"=w275:T11)  [unwired: 5 in, 1 out]
              n161 = local write "Increase Handler Velocity"(w279) -> ()
              n162 = call-poly <userlib>:"manageConfig.vi"("error in"=w286, "property path"="SCS.GPIB.Decrease Handler Velocity" ("key"), "config ref"=w275) -> ("error out"=w285:errorcluster, "value"=w278:string, "config ref out"=w284:T11)  [unwired: 5 in, 1 out]
              n163 = local write "Decrease Handler Velocity"(w278) -> ()
              n164 = call-poly <userlib>:"manageConfig.vi"("error in (no error)"=w285, "config ref"=w284) -> ()  [unwired: 9 in, 1 out]
            }
          }
        }
      }
    }
    frame #4 {
      # "This frame writes the headewr to the data log.\nIt includes setup and configuration information for the lot."
      n165 = local read "POWER"() -> (w307:bool)
      n166 = case shown="True" w307 {
        frame False {
        }
        frame True {
          w313 = "\r\n"
          n167 = local read "Lot number"() -> (w317:string)
          n168 = local read "Test cell ID"() -> (w315:string)
          n169 = local read "H1 online"() -> (w325:bool)
          n170 = local read "H2 online"() -> (w326:bool)
          n171 = local read "Data log path and filename"() -> (w308:path)
          n172 = local read "Operator name"() -> (w319:string)
          n173 = local read "H1 UPH warning limit hid"() -> (w321:dbl)
          n174 = local read "H2 UPH warning limit hid"() -> (w323:dbl)
          n175 = local read "H2  low yield warning"() -> (w322:dbl)
          n176 = local read "H1 low yield warning"() -> (w320:dbl)
          n177 = case shown="True" w325 {
            tunnel: ["H1 Off-Line" "H1 On-Line"] -> w327
            frame False {
            }
            frame True {
            }
          }
          n178 = case shown="True" w326 {
            tunnel: ["H2 Off-Line" "H2 On-Line"] -> w332
            frame False {
            }
            frame True {
            }
          }
          n179 = local write "Email alert - attachment (not editable)"(w308) -> ()
          n180 = Number To Decimal String(number=w320) -> (decimal integer string=w329:string)  [unwired: 1 in]
          n181 = Number To Decimal String(number=w321) -> (decimal integer string=w331:string)  [unwired: 1 in]
          n182 = Number To Decimal String(number=w322) -> (decimal integer string=w334:string)  [unwired: 1 in]
          n183 = Number To Decimal String(number=w323) -> (decimal integer string=w336:string)  [unwired: 1 in]
          n184 = Get Date/Time String() -> (date string=w310:string, time string=w312:string)  [unwired: 3 in]
          n185 = Concatenate Strings(w310, "   " ("string"), w312, w313, "Test Cell ID: ", w315, w313, "Lot Number: ", w317, w313, "Operator Name:  ", w319, w313, "System Started", w313, w327, w313, "H1 Low Yield Warning Limit: ", w329, w313, "H1 Low UPH Warning Limit: ", w331, w313, w332, w313, "H2 Low Yield Warning Limit: ", w334, w313, "H2 Low UPH Warning Limit: ", w336, w313, w313) -> (w337:string)
          n186 = call "SentinelDatalog.vi"("operation (0:open)"=T10."open or create", "String"=w337, "data log path"=w308) -> ()  [unwired: 8 in, 1 out]
        }
      }
    }
    frame #5 {
      # "This frame implements the main Sentinel Controller loop.\nAll loops within this frame execute as parallel processes."
      n187 = local read "POWER"() -> (w342:bool)
      n188 = case shown="True" w342 {
        frame False {
        }
        frame True {
          n189 = while {
            stop <- w357 stop-if-true
            w347 = 0
            w346 = 0.0
            w354 = 0
            w355 = 0.0
            # "Sentinel operating loop\n- tester loop\n- H1 loop\n- H2 loop\n- controls loop\n- alarm state machine loop\nExit with Power off"
            n190 = local read "POWER"() -> (w358:bool)
            n191 = Wait (ms)(milliseconds to wait=u32 100) -> ()  [unwired: 1 out]
            n192 = Not(x=w358) -> (.not. x?=w357:bool)
            n193 = while {
              i -> [w3014]
              stop <- w3030 stop-if-true
              n194 = local read "Run"() -> (w3006:bool)
              n195 = First Call?() -> (First Call?: T/F=w3007:bool)
              n196 = case shown="True" w3006 {
                frame False {
                  n197 = local write "Tester online"(FALSE ("Tester online")) -> ()
                  n198 = local write "H2 online"(FALSE ("H2 online")) -> ()
                  n199 = local write "H1 online"(FALSE ("H1 online")) -> ()
                }
                frame True {
                }
              }
              n200 = local read "Additional floorspace\nfor second handler"() -> (w3015:i32)
              n201 = Wait (ms)(milliseconds to wait=u32 50) -> ()  [unwired: 1 out]
              n202 = local read "Optimize handler speed"() -> (w3023:bool)
              n203 = local read "Std cell \nfloorspace area"() -> (w3028:i32)
              n204 = local read "Std cell \nfloorspace area"() -> (w3000:i32)
              n205 = local read "Celerint hardware cost ($/mo)"() -> (w3018:dbl)
              n206 = local read "Celerint licensing cost ($/mo)"() -> (w3017:dbl)
              n207 = local read "Second handler cost ($/mo)"() -> (w3016:dbl)
              n208 = case shown="True" w3007 {
                frame False {
                }
                frame True {
                  n209 = local read "H1 parallelism"() -> (w3063:u32)
                  n210 = local read "H2 parallelism"() -> (w3062:u32)
                  n211 = local read "H1 index time expected hid"() -> (w3061:dbl)
                  n212 = local read "H1 index time expected hid"() -> (w3071:dbl)
                  n213 = local read "H2 index time expected hid"() -> (w3060:dbl)
                  n214 = local read "H2 index time expected hid"() -> (w3072:dbl)
                  n215 = local read "Test time expected hid"() -> (w3069:dbl)
                  n216 = local write "H2 units/cycle"(w3062) -> ()
                  n217 = local write "H1 units/cycle"(w3063) -> ()
                  n218 = formula code="H1UPHorig=P1*3600/(T+H1ITorig);\nH2UPHorig=P2*3600/(T+H2ITorig);\nSYSH1WT=T-H1I;\nSYSH2WT=T-H2I;"("T"=w3069, "H1I"=w3061, "H2I"=w3060, "P1"=w3063, "H1ITorig"=w3071, "H2ITorig"=w3072, "P2"=w3062) -> ("H1UPHorig"=w3059:dbl, "H2UPHorig"=w3058:dbl, "SYSH1WT"=w3078:dbl, "SYSH2WT"=w3077:dbl)
                  n219 = local write "H1 Index Time 2"(w3061) -> ()
                  n220 = local write "H1 Test Time 2"(w3060) -> ()
                  n221 = local write "H1 P in formula"(w3063) -> ()
                  n222 = local write "H2 calc UPH"(w3058) -> ()
                  n223 = local read "H1 index time expected hid"() -> (w3065:dbl)
                  n224 = local read "H2 index time expected hid"() -> (w3064:dbl)
                  n225 = local read "Test time expected hid"() -> (w3066:dbl)
                  n226 = local write "H1 calc UPH"(w3059) -> ()
                  n227 = local write "UPH"(w3059) -> ()
                  n228 = local read "H2 parallelism"() -> (w3068:u32)
                  n229 = local read "H1 parallelism"() -> (w3067:u32)
                  n230 = Less Than 0?(x=w3078) -> (x < 0?=w3079:bool)
                  n231 = Less Than 0?(x=w3077) -> (x < 0?=w3080:bool)
                  n232 = Select(t=0.0, s=w3079, f=w3078) -> (s? t:f=w3074:dbl)
                  n233 = Select(t=0.0, s=w3080, f=w3077) -> (s? t:f=w3073:dbl)
                  n234 = local read "H1 index time expected hid"() -> (w3057:dbl)
                  n235 = local read "H2 index time expected hid"() -> (w3056:dbl)
                  n236 = local read "Test time expected hid"() -> (w3052:dbl)
                  n237 = formula code="ExpH1UPH=P1*3600/(T+SYSH1I+SYSH1WT);\nExpH2UPH=P2*3600/(T+SYSH2I+SYSH2WT);\nMaxUPH=Margin*(ExpH1UPH+ExpH2UPH);"("P1"=w3068, "T"=w3066, "SYSH1I"=w3065, "SYSH2I"=w3064, "Margin"=1.05 ("input variable"), "SYSH1WT"=w3074, "SYSH2WT"=w3073, "P2"=w3067) -> ("MaxUPH"=w3070:dbl, "ExpH1UPH"=w3076:dbl, "ExpH2UPH"=w3075:dbl)
                  n238 = Add(x=w3057, y=w3056) -> (x+y=w3055:dbl)
                  n239 = Divide(x=w3055, y=2.0) -> (x/y=w3053:dbl)
                  n240 = Add(x=w3052, y=w3053) -> (x+y=w3051:dbl)
                  n241 = Multiply(x=4000.0, y=w3051) -> (x*y=w3049:dbl)
                  n242 = To Unsigned Long Integer(number=w3049) -> (unsigned 32bit integer=w3048:u32)
                  n243 = local write "GPIB wait timeout hid"(w3048) -> ()
                  n244 = property on="System UPH" class="Knob (strict)"("Scale.Maximum"=w3070) -> ()  [unwired: 2 in, 2 out]
                  n245 = property on="H1 UPH" class="Knob (strict)"("Scale.Maximum"=w3076) -> ()  [unwired: 2 in, 2 out]
                  n246 = property on="H2 UPH" class="Knob (strict)"("Scale.Maximum"=w3075) -> ()  [unwired: 2 in, 2 out]
                }
              }
              n247 = local read "Handler cost ($/mo)"() -> (w3020:dbl)
              n248 = local read "Tester cost ($/mo)"() -> (w3021:dbl)
              n249 = local read "H1 online"() -> (w3010:bool)
              n250 = local read "H2 online"() -> (w3009:bool)
              n251 = local read "Overhead ($/mo)"() -> (w3019:dbl)
              n252 = local read "POWER"() -> (w3032:bool)
              n253 = Not(x=w3032) -> (.not. x?=w3031:bool)
              n254 = Not(x=w3010) -> (.not. x?=w2998:bool)
              n255 = Not(x=w3009) -> (.not. x?=w2997:bool)
              n256 = local read "Hours per month"() -> (w3002:i32)
              n257 = case shown="True" w3023 {
                frame False {
                }
                frame True {
                  # "place code here to optimize handler index times"
                }
              }
              n258 = local write "Std cell floorspace area"(w3000) -> ()
              n259 = Compound Arithmetic op=OR(w3031) -> (w3030:bool)
              n260 = And(x=w2998, y=w2997) -> (x .and. y?=w3008:bool)
              n261 = case shown="True" w2998 {
                frame False {
                }
                frame True {
                  n262 = local write "H1 nominal 2"(TRUE) -> ()
                  n263 = local write "H1 nominal"(TRUE) -> ()
                  n264 = local write "H1 warning 2"(TRUE) -> ()
                  n265 = local write "H1 warning"(TRUE) -> ()
                  n266 = local write "H1 alarm 2"(TRUE) -> ()
                  n267 = local write "H1 alarm"(TRUE) -> ()
                }
              }
              n268 = local write "H1 On/Off-line"(w2998) -> ()
              n269 = case shown="True" w2997 {
                frame False {
                }
                frame True {
                  n270 = local write "H2 nominal"(TRUE) -> ()
                  n271 = local write "H2 nominal 2"(TRUE) -> ()
                  n272 = local write "H2 warning"(TRUE) -> ()
                  n273 = local write "H2 warning 2"(TRUE) -> ()
                  n274 = local write "H2 alarm"(TRUE) -> ()
                  n275 = local write "H2 alarm 2"(TRUE) -> ()
                }
              }
              n276 = local write "H2 On/Off-line"(w2997) -> ()
              n277 = Add(x=w3015, y=w3028) -> (x+y=w2999:i32)
              n278 = Compound Arithmetic op=ADD(w3021, w3020, w3019) -> (w3025:dbl)
              n279 = Compound Arithmetic op=ADD(w3018, w3017, w3016) -> (w3026:dbl)
              n280 = Compound Arithmetic op=ADD(w3021, w3019) -> (w3003:dbl)
              n281 = case shown="False" w3008 {
                frame False {
                }
                frame True {
                  n282 = local write "System UPH"(u32 0 ("System UPH")) -> ()
                  n283 = local write "Sys utilization"(0.0 ("Sys utilization")) -> ()
                }
              }
              n284 = local write "Tandem\nfloorspace area"(w2999) -> ()
              n285 = Divide(x=w3026, y=w3002) -> (x/y=w3029:dbl)
              n286 = Add(x=w3026, y=w3025) -> (x+y=w3005:dbl)
              n287 = Divide(x=w3025, y=w3002) -> (x/y=w3001:dbl)
              n288 = local write "Hours per month 2"(w3002) -> ()
              n289 = local write "Total Mo Costs ($/mo) 2"(w3003) -> ()
              n290 = local write "Total Mo Costs ($/mo) 3"(w3005) -> ()
              n291 = local write "Std mo cost ($/mo)"(w3003) -> ()
              n292 = Add(x=w3001, y=w3029) -> (x+y=w3004:dbl)
              n293 = local write "Std hourly\ncost ($/hr)"(w3001) -> ()
              n294 = local read "Push to reset charts"() -> (w3012:bool)
              n295 = local write "Tandem hourly\ncost ($/hr)"(w3004) -> ()
              n296 = local read "Optimize handler speed"() -> (w3011:bool)
              n297 = case shown="True" w3012 {
                frame False {
                }
                frame True {
                  n298 = property on="YieldMon" class="WFChart (strict)"("History Data"=cluster{dbl, dbl, dbl, dbl}[] [{100.0, 100.0, 0.0, 0.0}]) -> ()  [unwired: 2 in, 2 out]
                  n299 = property on="SysUtilMon" class="WFChart (strict)"("History Data"=cluster{dbl, dbl}[] []) -> ()  [unwired: 2 in, 2 out]
                }
              }
              n300 = Equal To 0?(x=w3014) -> (x = 0?=w3013:bool)
              n301 = case shown="True" w3013 {
                frame False {
                }
                frame True {
                  w3107 = "" ("Message from tester")
                  w3110 = 0
                  w3113 = 0
                  w3126 = 100
                  w3127 = 0
                  w3128 = FALSE ("H1 alarm")
                  # "graphs and charts - declared here, displayed elsewhere"
                  n302 = Bundle(w3126, w3126, w3126, w3126) -> (w3105:cluster{i32, i32, i32, i32})  [unwired: 1 in]
                  n303 = Bundle(w3127, w3127) -> (w3104:cluster{i32, i32})  [unwired: 1 in]
                  n304 = local write "H2 Lock"(FALSE ("H2 Lock")) -> ()
                  n305 = local write "H1 alarm"(FALSE ("H1 warning")) -> ()
                  n306 = local write "H1 Lock"(FALSE ("H1 Lock")) -> ()
                  n307 = local write "H2 warning 2"(FALSE ("H1 warning")) -> ()
                  n308 = local write "H2 warning"(FALSE ("H1 warning")) -> ()
                  n309 = local write "H1 warning 2"(FALSE ("H1 warning")) -> ()
                  n310 = local write "H1 warning"(FALSE ("H1 warning")) -> ()
                  n311 = local write "H2 nominal 2"(TRUE ("H1 nominal")) -> ()
                  n312 = local write "H2 alarm 2"(FALSE ("H1 warning")) -> ()
                  n313 = local write "H2 alarm"(FALSE ("H1 warning")) -> ()
                  n314 = local write "H1 nominal 2"(TRUE ("H1 nominal")) -> ()
                  n315 = local write "H1 alarm 2"(FALSE ("H1 warning")) -> ()
                  n316 = local write "system statuts hid"(T9."H1NH2N" ("system statuts")) -> ()
                  n317 = local write "H1 Good Units"(w3113) -> ()
                  n318 = local write "H2 Device Count"(w3113) -> ()
                  n319 = local write "H2 Good Units"(w3113) -> ()
                  n320 = local write "H1 Device Count"(w3113) -> ()
                  n321 = property on="System UPH" class="Knob (strict)"("Scale.Minimum"=w3110) -> ()  [unwired: 2 in, 2 out]
                  n322 = property on="H1 UPH" class="Knob (strict)"("Scale.Minimum"=w3110) -> ()  [unwired: 2 in, 2 out]
                  n323 = property on="H2 UPH" class="Knob (strict)"("Scale.Minimum"=w3110) -> ()  [unwired: 2 in, 2 out]
                  n324 = property on="SysUtilMon" class="WFChart (strict)"("History Data"=cluster{dbl, dbl}[] []) -> ()  [unwired: 2 in, 2 out]
                  n325 = local write "H1 alarm"(w3128) -> ()
                  n326 = local write "H2 alarm"(w3128) -> ()
                  n327 = property on="YieldMon" class="WFChart (strict)"("History Data"=cluster{dbl, dbl, dbl, dbl}[] []) -> ()  [unwired: 2 in, 2 out]
                  n328 = local write "YieldMon"(w3105) -> ()
                  n329 = local write "SysUtilMon"(w3104) -> ()
                  n330 = local write "Sys utilization"(0.0) -> ()
                  n331 = local write "H2 alarm 2"(w3128) -> ()
                  n332 = local write "H1 alarm 2"(w3128) -> ()
                  n333 = local write "H2 nominal"(TRUE ("H1 nominal")) -> ()
                  n334 = local write "H1 nominal"(TRUE ("H1 nominal")) -> ()
                  n335 = local read "Lot number"() -> (w3102:string)
                  n336 = local write "Number of text alerts"(0.0 ("Number of Emails Alerts Sent")) -> ()
                  n337 = local write "Number of email alerts"(u32 0 ("Number of Emails Alerts Sent")) -> ()
                  n338 = local write "Tester loop counter hid"(u32 0 ("Tester loop counter")) -> ()
                  n339 = local write "H1 loop counter hid"(u32 0 ("H1 loop counter hid")) -> ()
                  n340 = local write "H2 loop counter hid"(u32 0 ("H2 loop counter hid")) -> ()
                  n341 = local write "H1 Waiting"(FALSE ("H1 Ready with sites")) -> ()
                  n342 = local write "H2 Waiting"(FALSE ("H1 Ready with sites")) -> ()
                  n343 = local write "GPIB Bus 0 traffic"(w3107) -> ()
                  n344 = local write "Notifications Lot Display"(w3102) -> ()
                  n345 = local write "GPIB bus 1 traffic"(w3107) -> ()
                  n346 = local write "GPIB bus 2 traffic"(w3107) -> ()
                }
              }
              n347 = case shown="True" w3011 {
                frame False {
                }
                frame True {
                  w3087 = FALSE
                  n348 = local read "H1 online"() -> (w3089:bool)
                  n349 = local read "H2 online"() -> (w3088:bool)
                  n350 = Equal?(x=w3089, y=w3087) -> (x = y?=w3091:bool)
                  n351 = Equal?(x=w3087, y=w3088) -> (x = y?=w3090:bool)
                  n352 = Or(x=w3091, y=w3090) -> (x .or. y?=w3086:bool)
                  n353 = case shown="True" w3086 {
                    frame False {
                    }
                    frame True {
                      n354 = local write "Optimize handler speed"(FALSE ("Optimize Handler Speed")) -> ()
                    }
                  }
                }
              }
              n355 = local read "Alert volume"() -> (w3022:u32)
              n356 = Equal To 0?(x=w3022) -> (x = 0?=w3024:bool)
              n357 = case shown="True" w3024 {
                frame False {
                }
                frame True {
                  n358 = local write "Audio On / Off"(FALSE ("Audio On/Off")) -> ()
                }
              }
            }
            n359 = case shown="True" FALSE {
              frame False {
              }
              frame True {
                n360 = while {
                  i -> [w870]
                  stop <- w883 stop-if-true
                  # "Play Audio Aert Loop"
                  n361 = local read "Ignore alarms until AFTER this many cycles"() -> (w875:i32)
                  n362 = local read "H1 Device Count"() -> (w880:u32)
                  n363 = local read "H2 Device Count"() -> (w879:u32)
                  n364 = local read "Program Parallelism"() -> (w877:u32)
                  n365 = local read "Run"() -> (w872:bool)
                  n366 = local read "POWER"() -> (w873:bool)
                  n367 = Add(x=w880, y=w879) -> (x+y=w878:u32)
                  n368 = Wait (ms)(milliseconds to wait=u32 100) -> ()  [unwired: 1 out]
                  n369 = Divide(x=w878, y=w877) -> (x/y=w876:dbl)
                  n370 = Greater?(x=w870, y=50) -> (0:w868:bool)
                  n371 = Greater?(x=w876, y=w875) -> (0:w874:bool)
                  n372 = Compound Arithmetic op=AND(w874, w873, w872, w868) -> (w871:bool)
                  n373 = case shown="True" w871 {
                    frame False {
                    }
                    frame True {
                      n374 = local read "system statuts hid"() -> (w887:T9)
                      n375 = case shown="\"H1AH2A\"" w887 {
                        frame "H1NH2N", Default {
                          n376 = Wait (ms)(milliseconds to wait=u32 50) -> ()  [unwired: 1 out]
                        }
                        frame "H1NH2W" {
                          n377 = flat-sequence {
                            frame #0 {
                              n378 = local read "Audio On / Off"() -> (w890:bool)
                              n379 = local read "H2 online"() -> (w889:bool)
                              n380 = And(x=w889, y=w890) -> (x .and. y?=w891:bool)
                              n381 = case shown="True" w891 {
                                frame False {
                                }
                                frame True {
                                n382 = local read "Run"() -> (w894:bool)
                                n383 = case shown="True" w894 {
                                tunnel: [0.001 w896] -> w893
                                frame False {
                                }
                                frame True {
                                n384 = local read "Alert volume"() -> (w896:u32)
                                }
                                }
                                n385 = call "PlayAlarm.vi"("wavefilename"="audio\\4_synth_warning.wav", "alertvolume"=w893) -> ()  [unwired: 10 in]
                                }
                              }
                            }
                            frame #1 {
                              n386 = local read "Run"() -> (w897:bool)
                              n387 = case shown="True" w897 {
                                frame False {
                                }
                                frame True {
                                n388 = Wait (ms)(milliseconds to wait=u32 5000) -> ()  [unwired: 1 out]
                                }
                              }
                            }
                          }
                        }
                        frame "H1NH2A" {
                          n389 = flat-sequence {
                            frame #0 {
                              n390 = local read "Audio On / Off"() -> (w901:bool)
                              n391 = local read "H2 online"() -> (w900:bool)
                              n392 = And(x=w900, y=w901) -> (x .and. y?=w899:bool)
                              n393 = case shown="True" w899 {
                                frame False {
                                }
                                frame True {
                                n394 = local read "Run"() -> (w904:bool)
                                n395 = case shown="True" w904 {
                                tunnel: [0.001 w906] -> w903
                                frame False {
                                }
                                frame True {
                                n396 = local read "Alert volume"() -> (w906:u32)
                                }
                                }
                                n397 = call "PlayAlarm.vi"("wavefilename"="audio\\bass_synth_alarm.wav", "alertvolume"=w903) -> ()  [unwired: 10 in]
                                }
                              }
                            }
                            frame #1 {
                              n398 = local read "Run"() -> (w907:bool)
                              n399 = case shown="True" w907 {
                                frame False {
                                n400 = Wait (ms)(milliseconds to wait=u32 50) -> ()  [unwired: 1 out]
                                }
                                frame True {
                                n401 = Wait (ms)(milliseconds to wait=u32 5000) -> ()  [unwired: 1 out]
                                }
                              }
                            }
                          }
                        }
                        frame "H1WH2N" {
                          n402 = flat-sequence {
                            frame #0 {
                              n403 = local read "Audio On / Off"() -> (w912:bool)
                              n404 = local read "H1 online"() -> (w911:bool)
                              n405 = And(x=w911, y=w912) -> (x .and. y?=w910:bool)
                              n406 = case shown="True" w910 {
                                frame False {
                                }
                                frame True {
                                n407 = local read "Run"() -> (w915:bool)
                                n408 = case shown="True" w915 {
                                tunnel: [0.001 w917] -> w914
                                frame False {
                                }
                                frame True {
                                n409 = local read "Alert volume"() -> (w917:u32)
                                }
                                }
                                n410 = call "PlayAlarm.vi"("wavefilename"="audio\\4_synth_warning.wav", "alertvolume"=w914) -> ()  [unwired: 10 in]
                                }
                              }
                            }
                            frame #1 {
                              n411 = local read "Run"() -> (w918:bool)
                              n412 = case shown="True" w918 {
                                frame False {
                                n413 = Wait (ms)(milliseconds to wait=u32 50) -> ()  [unwired: 1 out]
                                }
                                frame True {
                                n414 = Wait (ms)(milliseconds to wait=u32 5000) -> ()  [unwired: 1 out]
                                }
                              }
                            }
                          }
                        }
                        frame "H1WH2W" {
                          n415 = flat-sequence {
                            frame #0 {
                              n416 = local read "Audio On / Off"() -> (w924:bool)
                              n417 = local read "H1 online"() -> (w921:bool)
                              n418 = local read "H2 online"() -> (w923:bool)
                              n419 = Compound Arithmetic op=AND(w921, w923, w924) -> (w922:bool)
                              n420 = case shown="True" w922 {
                                frame False {
                                }
                                frame True {
                                n421 = local read "Run"() -> (w927:bool)
                                n422 = case shown="True" w927 {
                                tunnel: [0.001 w929] -> w926
                                frame False {
                                }
                                frame True {
                                n423 = local read "Alert volume"() -> (w929:u32)
                                }
                                }
                                n424 = call "PlayAlarm.vi"("wavefilename"="audio\\4_synth_warning.wav", "alertvolume"=w926) -> ()  [unwired: 10 in]
                                }
                              }
                            }
                            frame #1 {
                              n425 = local read "Run"() -> (w930:bool)
                              n426 = case shown="True" w930 {
                                frame False {
                                n427 = Wait (ms)(milliseconds to wait=u32 50) -> ()  [unwired: 1 out]
                                }
                                frame True {
                                n428 = Wait (ms)(milliseconds to wait=u32 5000) -> ()  [unwired: 1 out]
                                }
                              }
                            }
                          }
                        }
                        frame "H1WH2A" {
                          n429 = flat-sequence {
                            frame #0 {
                              n430 = local read "Audio On / Off"() -> (w936:bool)
                              n431 = local read "H1 online"() -> (w934:bool)
                              n432 = local read "H2 online"() -> (w935:bool)
                              n433 = Compound Arithmetic op=AND(w934, w935, w936) -> (w933:bool)
                              n434 = case shown="True" w933 {
                                frame False {
                                }
                                frame True {
                                n435 = local read "Run"() -> (w939:bool)
                                n436 = case shown="True" w939 {
                                tunnel: [0.001 w941] -> w938
                                frame False {
                                }
                                frame True {
                                n437 = local read "Alert volume"() -> (w941:u32)
                                }
                                }
                                n438 = call "PlayAlarm.vi"("wavefilename"="audio\\bass_synth_alarm.wav", "alertvolume"=w938) -> ()  [unwired: 10 in]
                                }
                              }
                            }
                            frame #1 {
                              n439 = local read "Run"() -> (w942:bool)
                              n440 = case shown="True" w942 {
                                frame False {
                                n441 = Wait (ms)(milliseconds to wait=u32 50) -> ()  [unwired: 1 out]
                                }
                                frame True {
                                n442 = Wait (ms)(milliseconds to wait=u32 5000) -> ()  [unwired: 1 out]
                                }
                              }
                            }
                          }
                        }
                        frame "H1AH2N" {
                          n443 = flat-sequence {
                            frame #0 {
                              n444 = local read "Audio On / Off"() -> (w947:bool)
                              n445 = local read "H1 online"() -> (w945:bool)
                              n446 = And(x=w945, y=w947) -> (x .and. y?=w946:bool)
                              n447 = case shown="True" w946 {
                                frame False {
                                }
                                frame True {
                                n448 = local read "Run"() -> (w950:bool)
                                n449 = case shown="True" w950 {
                                tunnel: [0.001 w952] -> w949
                                frame False {
                                }
                                frame True {
                                n450 = local read "Alert volume"() -> (w952:u32)
                                }
                                }
                                n451 = call "PlayAlarm.vi"("wavefilename"="audio\\bass_synth_alarm.wav", "alertvolume"=w949) -> ()  [unwired: 10 in]
                                }
                              }
                            }
                            frame #1 {
                              n452 = local read "Run"() -> (w953:bool)
                              n453 = case shown="True" w953 {
                                frame False {
                                n454 = Wait (ms)(milliseconds to wait=u32 50) -> ()  [unwired: 1 out]
                                }
                                frame True {
                                n455 = Wait (ms)(milliseconds to wait=u32 5000) -> ()  [unwired: 1 out]
                                }
                              }
                            }
                          }
                        }
                        frame "H1AH2W" {
                          n456 = flat-sequence {
                            frame #0 {
                              n457 = local read "Audio On / Off"() -> (w959:bool)
                              n458 = local read "H1 online"() -> (w957:bool)
                              n459 = local read "H2 online"() -> (w958:bool)
                              n460 = Compound Arithmetic op=AND(w957, w958, w959) -> (w956:bool)
                              n461 = case shown="True" w956 {
                                frame False {
                                }
                                frame True {
                                n462 = local read "Run"() -> (w962:bool)
                                n463 = case shown="True" w962 {
                                tunnel: [0.001 w964] -> w961
                                frame False {
                                }
                                frame True {
                                n464 = local read "Alert volume"() -> (w964:u32)
                                }
                                }
                                n465 = call "PlayAlarm.vi"("wavefilename"="audio\\bass_synth_alarm.wav", "alertvolume"=w961) -> ()  [unwired: 10 in]
                                }
                              }
                            }
                            frame #1 {
                              n466 = local read "Run"() -> (w965:bool)
                              n467 = case shown="True" w965 {
                                frame False {
                                n468 = Wait (ms)(milliseconds to wait=u32 50) -> ()  [unwired: 1 out]
                                }
                                frame True {
                                n469 = Wait (ms)(milliseconds to wait=u32 5000) -> ()  [unwired: 1 out]
                                }
                              }
                            }
                          }
                        }
                        frame "H1AH2A" {
                          n470 = flat-sequence {
                            frame #0 {
                              n471 = local read "Audio On / Off"() -> (w971:bool)
                              n472 = local read "H1 online"() -> (w969:bool)
                              n473 = local read "H2 online"() -> (w970:bool)
                              n474 = Compound Arithmetic op=AND(w969, w970, w971) -> (w968:bool)
                              n475 = case shown="True" w968 {
                                frame False {
                                }
                                frame True {
                                n476 = local read "Run"() -> (w974:bool)
                                n477 = case shown="True" w974 {
                                tunnel: [0.001 w976] -> w973
                                frame False {
                                }
                                frame True {
                                n478 = local read "Alert volume"() -> (w976:u32)
                                }
                                }
                                n479 = call "PlayAlarm.vi"("wavefilename"="audio\\bass_synth_alarm.wav", "alertvolume"=w973) -> ()  [unwired: 10 in]
                                }
                              }
                            }
                            frame #1 {
                              n480 = local read "Run"() -> (w977:bool)
                              n481 = case shown="True" w977 {
                                frame False {
                                n482 = Wait (ms)(milliseconds to wait=u32 50) -> ()  [unwired: 1 out]
                                }
                                frame True {
                                n483 = Wait (ms)(milliseconds to wait=u32 5000) -> ()  [unwired: 1 out]
                                }
                              }
                            }
                          }
                        }
                      }
                    }
                  }
                  n484 = local read "Run"() -> (w881:bool)
                  n485 = local read "POWER"() -> (w884:bool)
                  n486 = Not(x=w884) -> (.not. x?=w886:bool)
                  n487 = Not(x=w881) -> (.not. x?=w885:bool)
                  n488 = Compound Arithmetic op=OR(w886, w885) -> (w883:bool)
                }
              }
            }
            n489 = while {
              shift-right: [w2417] -> _
              shift-left: T9."H1NH2N" ("system statuts") -> [w2407]
              stop <- w2406 continue-if-true
              # "system status state machine:\n- writes data log whenever there is a change (if data loggin enabled)\n- issues email and text alerts is enabled (electronic notification of alarms)"
              n490 = local read "H1 parallelism"() -> (w2413:u32)
              n491 = local read "H1 Device Count"() -> (w2414:u32)
              n492 = local read "H2 Device Count"() -> (w2412:u32)
              n493 = local read "H2 parallelism"() -> (w2411:u32)
              n494 = local read "POWER"() -> (w2406:bool)
              n495 = Divide(x=w2412, y=w2411) -> (x/y=w2408:dbl)
              n496 = Divide(x=w2414, y=w2413) -> (x/y=w2409:dbl)
              n497 = local read "Ignore alarms until AFTER this many cycles"() -> (w2416:i32)
              n498 = Add(x=w2409, y=w2408) -> (x+y=w2410:dbl)
              n499 = Greater?(x=w2410, y=w2416) -> (0:w2415:bool)
              n500 = case shown="True" w2415 {
                tunnel: [w2419 w2422] -> w2417
                tunnel: w2407 -> [w2419 w2420]
                frame False {
                }
                frame True {
                  n501 = flat-sequence {
                    tunnel: [w2423] -> w2421
                    tunnel: w2420 -> [w2423]
                    tunnel: [w2520] -> w2422
                    tunnel: w2421 -> [w2518]
                    frame #0 {
                      # "Determine current state for System Status state-machine"
                      n502 = stacked-sequence {
                        frame #0 {
                          n503 = local read "H1 nominal 2"() -> (w2427:bool)
                          n504 = local read "H2 nominal 2"() -> (w2425:bool)
                          n505 = local read "H1 nominal"() -> (w2428:bool)
                          n506 = local read "H2 nominal"() -> (w2426:bool)
                          n507 = Compound Arithmetic op=AND(w2428, w2427, w2426, w2425) -> (w2424:bool)
                          n508 = case shown="True" w2424 {
                            frame False {
                            }
                            frame True {
                              n509 = local write "system statuts hid"(T9."H1NH2N" ("system statuts")) -> ()
                            }
                          }
                        }
                        frame #1 {
                          n510 = local read "H2 warning 2"() -> (w2432:bool)
                          n511 = local read "H2 warning"() -> (w2433:bool)
                          n512 = local read "H1 nominal 2"() -> (w2434:bool)
                          n513 = local read "H1 nominal"() -> (w2435:bool)
                          n514 = Or(x=w2433, y=w2432) -> (x .or. y?=w2431:bool)
                          n515 = Compound Arithmetic op=AND(w2435, w2434, w2431) -> (w2430:bool)
                          n516 = case shown="False" w2430 {
                            frame False {
                            }
                            frame True {
                              n517 = local write "system statuts hid"(T9."H1NH2W" ("system statuts")) -> ()
                            }
                          }
                        }
                        frame #2 {
                          n518 = local read "H1 nominal 2"() -> (w2442:bool)
                          n519 = local read "H1 nominal"() -> (w2443:bool)
                          n520 = local read "H2 alarm 2"() -> (w2440:bool)
                          n521 = local read "H2 alarm"() -> (w2441:bool)
                          n522 = Or(x=w2441, y=w2440) -> (x .or. y?=w2438:bool)
                          n523 = And(x=w2443, y=w2442) -> (x .and. y?=w2439:bool)
                          n524 = And(x=w2439, y=w2438) -> (x .and. y?=w2437:bool)
                          n525 = case shown="True" w2437 {
                            frame False {
                            }
                            frame True {
                              n526 = local write "system statuts hid"(T9."H1NH2A" ("system statuts")) -> ()
                            }
                          }
                        }
                        frame #3 {
                          n527 = local read "H1 alarm 2"() -> (w2453:bool)
                          n528 = local read "H1 alarm"() -> (w2454:bool)
                          n529 = local read "H2 nominal 2"() -> (w2456:bool)
                          n530 = local read "H1 warning 2"() -> (w2449:bool)
                          n531 = local read "H1 warning"() -> (w2450:bool)
                          n532 = local read "H2 nominal"() -> (w2455:bool)
                          n533 = Not(x=w2454) -> (.not. x?=w2452:bool)
                          n534 = Not(x=w2453) -> (.not. x?=w2451:bool)
                          n535 = Or(x=w2450, y=w2449) -> (x .or. y?=w2447:bool)
                          n536 = And(x=w2452, y=w2451) -> (x .and. y?=w2446:bool)
                          n537 = And(x=w2455, y=w2456) -> (x .and. y?=w2445:bool)
                          n538 = Compound Arithmetic op=AND(w2447, w2446, w2445) -> (w2448:bool)
                          n539 = case shown="True" w2448 {
                            frame False {
                            }
                            frame True {
                              n540 = local write "system statuts hid"(T9."H1WH2N" ("system statuts")) -> ()
                            }
                          }
                        }
                        frame #4 {
                          n541 = local read "H1 alarm 2"() -> (w2468:bool)
                          n542 = local read "H2 alarm 2"() -> (w2473:bool)
                          n543 = local read "H1 alarm"() -> (w2467:bool)
                          n544 = local read "H2 alarm"() -> (w2474:bool)
                          n545 = local read "H1 warning 2"() -> (w2464:bool)
                          n546 = local read "H2 warning 2"() -> (w2465:bool)
                          n547 = local read "H1 warning"() -> (w2463:bool)
                          n548 = local read "H2 warning"() -> (w2466:bool)
                          n549 = Not(x=w2467) -> (.not. x?=w2469:bool)
                          n550 = Not(x=w2468) -> (.not. x?=w2470:bool)
                          n551 = Not(x=w2474) -> (.not. x?=w2472:bool)
                          n552 = Not(x=w2473) -> (.not. x?=w2471:bool)
                          n553 = Or(x=w2463, y=w2464) -> (x .or. y?=w2461:bool)
                          n554 = Or(x=w2466, y=w2465) -> (x .or. y?=w2459:bool)
                          n555 = And(x=w2469, y=w2470) -> (x .and. y?=w2460:bool)
                          n556 = And(x=w2472, y=w2471) -> (x .and. y?=w2458:bool)
                          n557 = Compound Arithmetic op=AND(w2461, w2460, w2459, w2458) -> (w2462:bool)
                          n558 = case shown="True" w2462 {
                            frame False {
                            }
                            frame True {
                              n559 = local write "system statuts hid"(T9."H1WH2W" ("system statuts")) -> ()
                            }
                          }
                        }
                        frame #5 {
                          n560 = local read "H1 alarm 2"() -> (w2481:bool)
                          n561 = local read "H1 alarm"() -> (w2482:bool)
                          n562 = local read "H1 warning 2"() -> (w2484:bool)
                          n563 = local read "H1 warning"() -> (w2485:bool)
                          n564 = local read "H2 alarm 2"() -> (w2486:bool)
                          n565 = local read "H2 alarm"() -> (w2487:bool)
                          n566 = Not(x=w2482) -> (.not. x?=w2480:bool)
                          n567 = Not(x=w2481) -> (.not. x?=w2479:bool)
                          n568 = Or(x=w2485, y=w2484) -> (x .or. y?=w2478:bool)
                          n569 = Or(x=w2487, y=w2486) -> (x .or. y?=w2476:bool)
                          n570 = And(x=w2480, y=w2479) -> (x .and. y?=w2477:bool)
                          n571 = Compound Arithmetic op=AND(w2478, w2477, w2476) -> (w2483:bool)
                          n572 = case shown="True" w2483 {
                            frame False {
                            }
                            frame True {
                              n573 = local write "system statuts hid"(T9."H1WH2A" ("system statuts")) -> ()
                            }
                          }
                        }
                        frame #6 {
                          n574 = local read "H2 nominal 2"() -> (w2494:bool)
                          n575 = local read "H2 nominal"() -> (w2495:bool)
                          n576 = local read "H1 alarm 2"() -> (w2492:bool)
                          n577 = local read "H1 alarm"() -> (w2493:bool)
                          n578 = Or(x=w2493, y=w2492) -> (x .or. y?=w2490:bool)
                          n579 = And(x=w2495, y=w2494) -> (x .and. y?=w2489:bool)
                          n580 = And(x=w2490, y=w2489) -> (x .and. y?=w2491:bool)
                          n581 = case shown="True" w2491 {
                            frame False {
                            }
                            frame True {
                              n582 = local write "system statuts hid"(T9."H1AH2N" ("system statuts")) -> ()
                            }
                          }
                        }
                        frame #7 {
                          n583 = local read "H2 alarm 2"() -> (w2499:bool)
                          n584 = local read "H2 alarm"() -> (w2500:bool)
                          n585 = local read "H2 warning 2"() -> (w2505:bool)
                          n586 = local read "H2 warning"() -> (w2506:bool)
                          n587 = local read "H1 alarm 2"() -> (w2507:bool)
                          n588 = local read "H1 alarm"() -> (w2508:bool)
                          n589 = Not(x=w2500) -> (.not. x?=w2498:bool)
                          n590 = Not(x=w2499) -> (.not. x?=w2497:bool)
                          n591 = Or(x=w2508, y=w2507) -> (x .or. y?=w2503:bool)
                          n592 = Or(x=w2506, y=w2505) -> (x .or. y?=w2502:bool)
                          n593 = And(x=w2498, y=w2497) -> (x .and. y?=w2501:bool)
                          n594 = Compound Arithmetic op=AND(w2503, w2502, w2501) -> (w2504:bool)
                          n595 = case shown="True" w2504 {
                            frame False {
                            }
                            frame True {
                              n596 = local write "system statuts hid"(T9."H1AH2W" ("system statuts")) -> ()
                            }
                          }
                        }
                        frame #8 {
                          n597 = local read "H1 alarm 2"() -> (w2514:bool)
                          n598 = local read "H2 alarm 2"() -> (w2513:bool)
                          n599 = local read "H1 alarm"() -> (w2515:bool)
                          n600 = local read "H2 alarm"() -> (w2512:bool)
                          n601 = Or(x=w2515, y=w2514) -> (x .or. y?=w2510:bool)
                          n602 = Or(x=w2512, y=w2513) -> (x .or. y?=w2511:bool)
                          n603 = And(x=w2510, y=w2511) -> (x .and. y?=w2516:bool)
                          n604 = case shown="True" w2516 {
                            frame False {
                            }
                            frame True {
                              n605 = local write "system statuts hid"(T9."H1AH2A" ("system statuts")) -> ()
                            }
                          }
                        }
                      }
                    }
                    frame #1 {
                      n606 = local read "system statuts hid"() -> (w2520:T9)
                      n607 = Not Equal?(x=w2520, y=w2518) -> (x != y?=w2519:bool)
                      n608 = case shown="True" w2519 {
                        tunnel: w2520 -> [_ w2522]
                        frame False {
                        }
                        frame True {
                          n609 = local read "Enable data logging of all events"() -> (w2521:bool)
                          n610 = case shown="True" w2521 {
                            tunnel: w2522 -> [_ w2523]
                            frame False {
                            }
                            frame True {
                              n611 = stacked-sequence {
                                tunnel: w2523 -> [_ w2526 _ _ _]
                                frame #0 {
                                n612 = local read "Number of data log entries hid"() -> (w2525:u32)
                                n613 = Increment(x=w2525) -> (x+1=w2524:u32)
                                n614 = local write "Number of data log entries hid"(w2524) -> ()
                                }
                                frame #1 {
                                n615 = case shown="\"H1AH2A\"" w2526 {
                                frame "H1NH2N", Default {
                                w2533 = "\r\n"
                                n616 = local read "H1 online"() -> (w2550:bool)
                                n617 = local read "H2 online"() -> (w2551:bool)
                                n618 = local read "Number of data log entries hid"() -> (w2527:u32)
                                n619 = local read "H1 UPH warning limit hid"() -> (w2546:dbl)
                                n620 = local read "H2 UPH warning limit hid"() -> (w2548:dbl)
                                n621 = local read "YieldMon"() -> (w2531:cluster{i32, i32, i32, i32})
                                n622 = local read "H2  low yield warning"() -> (w2547:dbl)
                                n623 = local read "H1 low yield warning"() -> (w2545:dbl)
                                n624 = local read "H1 UPH"() -> (w2539:cluster{u32, u32})
                                n625 = local read "H2 UPH"() -> (w2537:cluster{u32, u32})
                                n626 = local read "YieldMon"() -> (w2529:cluster{i32, i32, i32, i32})
                                n627 = case shown="True" w2550 {
                                tunnel: ["H1 Off-Line" "H1 On-Line"] -> w2552
                                frame False {
                                }
                                frame True {
                                }
                                }
                                n628 = case shown="True" w2551 {
                                tunnel: ["H2 Off-Line" "H2 On-Line"] -> w2561
                                frame False {
                                }
                                frame True {
                                }
                                }
                                n629 = Unbundle(w2531) -> (w2530:i32)  [unwired: 3 out]
                                n630 = Unbundle(w2539) -> (w2538:u32)  [unwired: 1 out]
                                n631 = Unbundle(w2529) -> (w2528:i32)  [unwired: 3 out]
                                n632 = Unbundle(w2537) -> (w2536:u32)  [unwired: 1 out]
                                n633 = local read "Data log path and filename"() -> (w2535:path)
                                n634 = Number To Decimal String(number=w2545) -> (decimal integer string=w2554:string)  [unwired: 1 in]
                                n635 = Number To Decimal String(number=w2530) -> (decimal integer string=w2556:string)  [unwired: 1 in]
                                n636 = Number To Decimal String(number=w2546) -> (decimal integer string=w2558:string)  [unwired: 1 in]
                                n637 = Number To Decimal String(number=w2538) -> (decimal integer string=w2560:string)  [unwired: 1 in]
                                n638 = Number To Decimal String(number=w2547) -> (decimal integer string=w2563:string)  [unwired: 1 in]
                                n639 = Number To Decimal String(number=w2528) -> (decimal integer string=w2565:string)  [unwired: 1 in]
                                n640 = Number To Decimal String(number=w2548) -> (decimal integer string=w2567:string)  [unwired: 1 in]
                                n641 = Number To Decimal String(number=w2536) -> (decimal integer string=w2569:string)  [unwired: 1 in]
                                n642 = Number To Decimal String(number=w2527) -> (decimal integer string=w2532:string)  [unwired: 1 in]
                                n643 = Get Date/Time String(want seconds? (F)=TRUE) -> (date string=w2543:string, time string=w2544:string)  [unwired: 2 in]
                                n644 = Concatenate Strings(w2532, w2533, w2543, "   " ("string"), w2544, w2533, "H1 Nominal, H2 Nominal", w2533, w2552, w2533, "H1 Low Yield Warning Limit: ", w2554, ", H1 yield = ", w2556, w2533, "H1 Low UPH Warning Limit: ", w2558, ", H1 UPH = ", w2560, w2533, w2561, w2533, "H2 Low Yield Warning Limit: ", w2563, ", H2 yield = ", w2565, w2533, "H2 Low UPH Warning Limit: ", w2567, ", H2 UPH = ", w2569, w2533, w2533) -> (w2541:string)
                                n645 = call "SentinelDatalog.vi"("operation (0:open)"=T10."open", "String"=w2541, "data log path"=w2535) -> ()  [unwired: 8 in, 1 out]
                                }
                                frame "H1NH2W" {
                                w2579 = "\r\n"
                                n646 = local read "H1 online"() -> (w2597:bool)
                                n647 = local read "H2 online"() -> (w2598:bool)
                                n648 = local read "H1 UPH warning limit hid"() -> (w2593:dbl)
                                n649 = local read "H2 UPH warning limit hid"() -> (w2595:dbl)
                                n650 = local read "YieldMon"() -> (w2578:cluster{i32, i32, i32, i32})
                                n651 = local read "H2  low yield warning"() -> (w2594:dbl)
                                n652 = local read "H1 low yield warning"() -> (w2592:dbl)
                                n653 = local read "H1 UPH"() -> (w2586:cluster{u32, u32})
                                n654 = local read "H2 UPH"() -> (w2584:cluster{u32, u32})
                                n655 = local read "YieldMon"() -> (w2576:cluster{i32, i32, i32, i32})
                                n656 = local read "Number of data log entries hid"() -> (w2574:u32)
                                n657 = case shown="True" w2597 {
                                tunnel: ["H1 Off-Line" "H1 On-Line"] -> w2599
                                frame False {
                                }
                                frame True {
                                }
                                }
                                n658 = case shown="True" w2598 {
                                tunnel: ["H2 Off-Line" "H2 On-Line"] -> w2608
                                frame False {
                                }
                                frame True {
                                }
                                }
                                n659 = Unbundle(w2576) -> (w2575:i32)  [unwired: 3 out]
                                n660 = Unbundle(w2586) -> (w2585:u32)  [unwired: 1 out]
                                n661 = Unbundle(w2578) -> (w2577:i32)  [unwired: 3 out]
                                n662 = Unbundle(w2584) -> (w2583:u32)  [unwired: 1 out]
                                n663 = Number To Decimal String(number=w2592) -> (decimal integer string=w2601:string)  [unwired: 1 in]
                                n664 = Number To Decimal String(number=w2575) -> (decimal integer string=w2603:string)  [unwired: 1 in]
                                n665 = Number To Decimal String(number=w2593) -> (decimal integer string=w2605:string)  [unwired: 1 in]
                                n666 = Number To Decimal String(number=w2585) -> (decimal integer string=w2607:string)  [unwired: 1 in]
                                n667 = Number To Decimal String(number=w2594) -> (decimal integer string=w2610:string)  [unwired: 1 in]
                                n668 = Number To Decimal String(number=w2577) -> (decimal integer string=w2612:string)  [unwired: 1 in]
                                n669 = Number To Decimal String(number=w2595) -> (decimal integer string=w2614:string)  [unwired: 1 in]
                                n670 = Number To Decimal String(number=w2583) -> (decimal integer string=w2616:string)  [unwired: 1 in]
                                n671 = Number To Decimal String(number=w2574) -> (decimal integer string=w2580:string)  [unwired: 1 in]
                                n672 = local read "Data log path and filename"() -> (w2582:path)
                                n673 = Get Date/Time String(want seconds? (F)=TRUE) -> (date string=w2590:string, time string=w2591:string)  [unwired: 2 in]
                                n674 = Concatenate Strings(w2580, w2579, w2590, "   " ("string"), w2591, w2579, "H1 Nominal, H2 Warning", w2579, w2599, w2579, "H1 Low Yield Warning Limit: ", w2601, ", H1 yield = ", w2603, w2579, "H1 Low UPH Warning Limit: ", w2605, ", H1 UPH = ", w2607, w2579, w2608, w2579, "H2 Low Yield Warning Limit: ", w2610, ", H2 yield = ", w2612, w2579, "H2 Low UPH Warning Limit: ", w2614, ", H2 UPH = ", w2616, w2579, w2579) -> (w2588:string)
                                n675 = call "SentinelDatalog.vi"("operation (0:open)"=T10."open", "String"=w2588, "data log path"=w2582) -> ()  [unwired: 8 in, 1 out]
                                }
                                frame "H1NH2A" {
                                w2627 = "\r\n"
                                n676 = local read "H1 online"() -> (w2644:bool)
                                n677 = local read "H2 online"() -> (w2645:bool)
                                n678 = local read "Number of data log entries hid"() -> (w2621:u32)
                                n679 = local read "H1 UPH warning limit hid"() -> (w2640:dbl)
                                n680 = local read "H1 low yield warning"() -> (w2639:dbl)
                                n681 = local read "H2 UPH alarm limit hid"() -> (w2642:dbl)
                                n682 = local read "YieldMon"() -> (w2625:cluster{i32, i32, i32, i32})
                                n683 = local read "H1 UPH"() -> (w2633:cluster{u32, u32})
                                n684 = local read "H2 low yield alarm"() -> (w2641:dbl)
                                n685 = local read "H2 UPH"() -> (w2632:cluster{u32, u32})
                                n686 = local read "YieldMon"() -> (w2623:cluster{i32, i32, i32, i32})
                                n687 = case shown="True" w2644 {
                                tunnel: ["H1 Off-Line" "H1 On-Line"] -> w2646
                                frame False {
                                }
                                frame True {
                                }
                                }
                                n688 = case shown="True" w2645 {
                                tunnel: ["H2 Off-Line" "H2 On-Line"] -> w2655
                                frame False {
                                }
                                frame True {
                                }
                                }
                                n689 = Number To Decimal String(number=w2621) -> (decimal integer string=w2626:string)  [unwired: 1 in]
                                n690 = Unbundle(w2625) -> (w2624:i32)  [unwired: 3 out]
                                n691 = Unbundle(w2633) -> (w2630:u32)  [unwired: 1 out]
                                n692 = Unbundle(w2623) -> (w2622:i32)  [unwired: 3 out]
                                n693 = Unbundle(w2632) -> (w2631:u32)  [unwired: 1 out]
                                n694 = Number To Decimal String(number=w2639) -> (decimal integer string=w2648:string)  [unwired: 1 in]
                                n695 = Number To Decimal String(number=w2624) -> (decimal integer string=w2650:string)  [unwired: 1 in]
                                n696 = Number To Decimal String(number=w2640) -> (decimal integer string=w2652:string)  [unwired: 1 in]
                                n697 = Number To Decimal String(number=w2630) -> (decimal integer string=w2654:string)  [unwired: 1 in]
                                n698 = Number To Decimal String(number=w2641) -> (decimal integer string=w2657:string)  [unwired: 1 in]
                                n699 = Number To Decimal String(number=w2622) -> (decimal integer string=w2659:string)  [unwired: 1 in]
                                n700 = Number To Decimal String(number=w2642) -> (decimal integer string=w2661:string)  [unwired: 1 in]
                                n701 = Number To Decimal String(number=w2631) -> (decimal integer string=w2663:string)  [unwired: 1 in]
                                n702 = local read "Data log path and filename"() -> (w2629:path)
                                n703 = Get Date/Time String(want seconds? (F)=TRUE) -> (date string=w2637:string, time string=w2638:string)  [unwired: 2 in]
                                n704 = Concatenate Strings(w2626, w2627, w2637, "   " ("string"), w2638, w2627, "H1 Nominal, H2 Alarming", w2627, w2646, w2627, "H1 Low Yield Warning Limit: ", w2648, ", H1 yield = ", w2650, w2627, "H1 Low UPH Warning Limit: ", w2652, ", H1 UPH = ", w2654, w2627, w2655, w2627, "H2 Low Yield Alarm Limit: ", w2657, ", H2 yield = ", w2659, w2627, "H2 Low UPH Alarm Limit: ", w2661, ", H2 UPH = ", w2663, w2627, w2627) -> (w2635:string)
                                n705 = call "SentinelDatalog.vi"("operation (0:open)"=T10."open", "String"=w2635, "data log path"=w2629) -> ()  [unwired: 8 in, 1 out]
                                }
                                frame "H1WH2N" {
                                w2674 = "\r\n"
                                n706 = local read "H1 online"() -> (w2692:bool)
                                n707 = local read "H2 online"() -> (w2693:bool)
                                n708 = local read "H1 UPH warning limit hid"() -> (w2688:dbl)
                                n709 = local read "H2 UPH warning limit hid"() -> (w2690:dbl)
                                n710 = local read "H2  low yield warning"() -> (w2689:dbl)
                                n711 = local read "H1 low yield warning"() -> (w2687:dbl)
                                n712 = local read "H1 UPH"() -> (w2680:cluster{u32, u32})
                                n713 = local read "H2 UPH"() -> (w2679:cluster{u32, u32})
                                n714 = local read "YieldMon"() -> (w2672:cluster{i32, i32, i32, i32})
                                n715 = local read "YieldMon"() -> (w2670:cluster{i32, i32, i32, i32})
                                n716 = local read "Number of data log entries hid"() -> (w2668:u32)
                                n717 = case shown="True" w2692 {
                                tunnel: ["H1 Off-Line" "H1 On-Line"] -> w2681
                                frame False {
                                }
                                frame True {
                                }
                                }
                                n718 = case shown="True" w2693 {
                                tunnel: ["H2 Off-Line" "H2 On-Line"] -> w2702
                                frame False {
                                }
                                frame True {
                                }
                                }
                                n719 = Unbundle(w2672) -> (w2671:i32)  [unwired: 3 out]
                                n720 = Unbundle(w2680) -> (w2677:u32)  [unwired: 1 out]
                                n721 = Unbundle(w2670) -> (w2669:i32)  [unwired: 3 out]
                                n722 = Unbundle(w2679) -> (w2678:u32)  [unwired: 1 out]
                                n723 = Number To Decimal String(number=w2687) -> (decimal integer string=w2695:string)  [unwired: 1 in]
                                n724 = Number To Decimal String(number=w2671) -> (decimal integer string=w2697:string)  [unwired: 1 in]
                                n725 = Number To Decimal String(number=w2688) -> (decimal integer string=w2699:string)  [unwired: 1 in]
                                n726 = Number To Decimal String(number=w2677) -> (decimal integer string=w2701:string)  [unwired: 1 in]
                                n727 = Number To Decimal String(number=w2689) -> (decimal integer string=w2704:string)  [unwired: 1 in]
                                n728 = Number To Decimal String(number=w2669) -> (decimal integer string=w2706:string)  [unwired: 1 in]
                                n729 = Number To Decimal String(number=w2690) -> (decimal integer string=w2708:string)  [unwired: 1 in]
                                n730 = Number To Decimal String(number=w2678) -> (decimal integer string=w2710:string)  [unwired: 1 in]
                                n731 = local read "Data log path and filename"() -> (w2676:path)
                                n732 = Number To Decimal String(number=w2668) -> (decimal integer string=w2673:string)  [unwired: 1 in]
                                n733 = Get Date/Time String(want seconds? (F)=TRUE) -> (date string=w2685:string, time string=w2686:string)  [unwired: 2 in]
                                n734 = Concatenate Strings(w2673, w2674, w2685, "   " ("string"), w2686, w2674, "H1 Warning, H2 Nominal", w2674, w2681, w2674, "H1 Low Yield Warning Limit: ", w2695, ", H1 yield = ", w2697, w2674, "H1 Low UPH Warning Limit: ", w2699, ", H1 UPH = ", w2701, w2674, w2702, w2674, "H2 Low Yield Warning Limit: ", w2704, ", H2 yield = ", w2706, w2674, "H2 Low UPH Warning Limit: ", w2708, ", H2 UPH = ", w2710, w2674, w2674) -> (w2683:string)
                                n735 = call "SentinelDatalog.vi"("operation (0:open)"=T10."open", "String"=w2683, "data log path"=w2676) -> ()  [unwired: 8 in, 1 out]
                                }
                                frame "H1WH2W" {
                                w2720 = "\r\n"
                                w2728 = "\r\n"
                                n736 = local read "H1 online"() -> (w2739:bool)
                                n737 = local read "H2 online"() -> (w2740:bool)
                                n738 = local read "H1 UPH warning limit hid"() -> (w2735:dbl)
                                n739 = local read "H2 UPH warning limit hid"() -> (w2737:dbl)
                                n740 = local read "H2  low yield warning"() -> (w2736:dbl)
                                n741 = local read "H1 low yield warning"() -> (w2734:dbl)
                                n742 = local read "H1 UPH"() -> (w2727:cluster{u32, u32})
                                n743 = local read "H2 UPH"() -> (w2726:cluster{u32, u32})
                                n744 = local read "YieldMon"() -> (w2719:cluster{i32, i32, i32, i32})
                                n745 = local read "YieldMon"() -> (w2717:cluster{i32, i32, i32, i32})
                                n746 = case shown="True" w2739 {
                                tunnel: ["H1 Off-Line" "H1 On-Line"] -> w2741
                                frame False {
                                }
                                frame True {
                                }
                                }
                                n747 = case shown="True" w2740 {
                                tunnel: ["H2 Off-Line" "H2 On-Line"] -> w2750
                                frame False {
                                }
                                frame True {
                                }
                                }
                                n748 = local read "Number of data log entries hid"() -> (w2715:u32)
                                n749 = Unbundle(w2719) -> (w2718:i32)  [unwired: 3 out]
                                n750 = Unbundle(w2727) -> (w2725:u32)  [unwired: 1 out]
                                n751 = Unbundle(w2717) -> (w2716:i32)  [unwired: 3 out]
                                n752 = Unbundle(w2726) -> (w2724:u32)  [unwired: 1 out]
                                n753 = Number To Decimal String(number=w2734) -> (decimal integer string=w2743:string)  [unwired: 1 in]
                                n754 = Number To Decimal String(number=w2718) -> (decimal integer string=w2745:string)  [unwired: 1 in]
                                n755 = Number To Decimal String(number=w2735) -> (decimal integer string=w2747:string)  [unwired: 1 in]
                                n756 = Number To Decimal String(number=w2725) -> (decimal integer string=w2749:string)  [unwired: 1 in]
                                n757 = Number To Decimal String(number=w2736) -> (decimal integer string=w2752:string)  [unwired: 1 in]
                                n758 = Number To Decimal String(number=w2716) -> (decimal integer string=w2754:string)  [unwired: 1 in]
                                n759 = Number To Decimal String(number=w2737) -> (decimal integer string=w2756:string)  [unwired: 1 in]
                                n760 = Number To Decimal String(number=w2724) -> (decimal integer string=w2758:string)  [unwired: 1 in]
                                n761 = local read "Data log path and filename"() -> (w2723:path)
                                n762 = Get Date/Time String(want seconds? (F)=TRUE) -> (date string=w2732:string, time string=w2733:string)  [unwired: 2 in]
                                n763 = Number To Decimal String(number=w2715) -> (decimal integer string=w2721:string)  [unwired: 1 in]
                                n764 = Concatenate Strings(w2721, w2720, w2732, "   " ("string"), w2733, w2720, "H1 Warning, H2 Warning", w2720, w2741, w2720, "H1 Low Yield Warning Limit: ", w2743, ", H1 yield = ", w2745, w2728, "H1 Low UPH Warning Limit: ", w2747, ", H1 UPH = ", w2749, w2728, w2750, w2728, "H2 Low Yield Warning Limit: ", w2752, ", H2 yield = ", w2754, w2728, "H2 Low UPH Warning Limit: ", w2756, ", H2 UPH = ", w2758, w2728, w2728) -> (w2730:string)
                                n765 = call "SentinelDatalog.vi"("operation (0:open)"=T10."open", "String"=w2730, "data log path"=w2723) -> ()  [unwired: 8 in, 1 out]
                                }
                                frame "H1WH2A" {
                                w2769 = "\r\n"
                                n766 = local read "H1 online"() -> (w2786:bool)
                                n767 = local read "H2 online"() -> (w2787:bool)
                                n768 = local read "H1 UPH warning limit hid"() -> (w2782:dbl)
                                n769 = local read "H1 low yield warning"() -> (w2781:dbl)
                                n770 = local read "H2 UPH alarm limit hid"() -> (w2784:dbl)
                                n771 = local read "H1 UPH"() -> (w2775:cluster{u32, u32})
                                n772 = local read "H2 low yield alarm"() -> (w2783:dbl)
                                n773 = local read "H2 UPH"() -> (w2774:cluster{u32, u32})
                                n774 = local read "YieldMon"() -> (w2765:cluster{i32, i32, i32, i32})
                                n775 = local read "YieldMon"() -> (w2767:cluster{i32, i32, i32, i32})
                                n776 = local read "Number of data log entries hid"() -> (w2763:u32)
                                n777 = case shown="True" w2786 {
                                tunnel: ["H1 Off-Line" "H1 On-Line"] -> w2788
                                frame False {
                                }
                                frame True {
                                }
                                }
                                n778 = case shown="True" w2787 {
                                tunnel: ["H2 Off-Line" "H2 On-Line"] -> w2797
                                frame False {
                                }
                                frame True {
                                }
                                }
                                n779 = Unbundle(w2765) -> (w2764:i32)  [unwired: 3 out]
                                n780 = Unbundle(w2775) -> (w2773:u32)  [unwired: 1 out]
                                n781 = Unbundle(w2767) -> (w2766:i32)  [unwired: 3 out]
                                n782 = Unbundle(w2774) -> (w2772:u32)  [unwired: 1 out]
                                n783 = Number To Decimal String(number=w2781) -> (decimal integer string=w2790:string)  [unwired: 1 in]
                                n784 = Number To Decimal String(number=w2764) -> (decimal integer string=w2792:string)  [unwired: 1 in]
                                n785 = Number To Decimal String(number=w2782) -> (decimal integer string=w2794:string)  [unwired: 1 in]
                                n786 = Number To Decimal String(number=w2773) -> (decimal integer string=w2796:string)  [unwired: 1 in]
                                n787 = Number To Decimal String(number=w2783) -> (decimal integer string=w2799:string)  [unwired: 1 in]
                                n788 = Number To Decimal String(number=w2766) -> (decimal integer string=w2801:string)  [unwired: 1 in]
                                n789 = Number To Decimal String(number=w2784) -> (decimal integer string=w2803:string)  [unwired: 1 in]
                                n790 = Number To Decimal String(number=w2772) -> (decimal integer string=w2805:string)  [unwired: 1 in]
                                n791 = local read "Data log path and filename"() -> (w2771:path)
                                n792 = Get Date/Time String(want seconds? (F)=TRUE) -> (date string=w2779:string, time string=w2780:string)  [unwired: 2 in]
                                n793 = Number To Decimal String(number=w2763) -> (decimal integer string=w2768:string)  [unwired: 1 in]
                                n794 = Concatenate Strings(w2768, w2769, w2779, "   " ("string"), w2780, w2769, "H1 Warning, H2 Alarming", w2769, w2788, w2769, "H1 Low Yield Warning Limit: ", w2790, ", H1 yield = ", w2792, w2769, "H1 Low UPH Warning Limit: ", w2794, ", H1 UPH = ", w2796, w2769, w2797, w2769, "H2 Low Yield Alarm Limit: ", w2799, ", H2 yield = ", w2801, w2769, "H2 Low UPH Alarm Limit: ", w2803, ", H2 UPH = ", w2805, w2769, w2769) -> (w2777:string)
                                n795 = call "SentinelDatalog.vi"("operation (0:open)"=T10."open", "String"=w2777, "data log path"=w2771) -> ()  [unwired: 8 in, 1 out]
                                }
                                frame "H1AH2N" {
                                w2816 = "\r\n"
                                n796 = local read "H1 online"() -> (w2833:bool)
                                n797 = local read "H2 online"() -> (w2834:bool)
                                n798 = local read "H2 UPH warning limit hid"() -> (w2831:dbl)
                                n799 = local read "H2  low yield warning"() -> (w2830:dbl)
                                n800 = local read "H1 UPH alarm limit hid"() -> (w2829:dbl)
                                n801 = local read "H1 low yield alarm"() -> (w2828:dbl)
                                n802 = local read "H1 UPH"() -> (w2822:cluster{u32, u32})
                                n803 = local read "H2 UPH"() -> (w2821:cluster{u32, u32})
                                n804 = local read "YieldMon"() -> (w2814:cluster{i32, i32, i32, i32})
                                n805 = local read "YieldMon"() -> (w2812:cluster{i32, i32, i32, i32})
                                n806 = case shown="True" w2833 {
                                tunnel: ["H1 Off-Line" "H1 On-Line"] -> w2835
                                frame False {
                                }
                                frame True {
                                }
                                }
                                n807 = case shown="False" w2834 {
                                tunnel: ["H2 Off-Line" "H2 On-Line"] -> w2844
                                frame False {
                                }
                                frame True {
                                }
                                }
                                n808 = local read "Number of data log entries hid"() -> (w2810:u32)
                                n809 = Unbundle(w2814) -> (w2813:i32)  [unwired: 3 out]
                                n810 = Unbundle(w2822) -> (w2820:u32)  [unwired: 1 out]
                                n811 = Unbundle(w2812) -> (w2811:i32)  [unwired: 3 out]
                                n812 = Unbundle(w2821) -> (w2819:u32)  [unwired: 1 out]
                                n813 = Number To Decimal String(number=w2828) -> (decimal integer string=w2837:string)  [unwired: 1 in]
                                n814 = Number To Decimal String(number=w2813) -> (decimal integer string=w2839:string)  [unwired: 1 in]
                                n815 = Number To Decimal String(number=w2829) -> (decimal integer string=w2841:string)  [unwired: 1 in]
                                n816 = Number To Decimal String(number=w2820) -> (decimal integer string=w2843:string)  [unwired: 1 in]
                                n817 = Number To Decimal String(number=w2830) -> (decimal integer string=w2846:string)  [unwired: 1 in]
                                n818 = Number To Decimal String(number=w2811) -> (decimal integer string=w2848:string)  [unwired: 1 in]
                                n819 = Number To Decimal String(number=w2831) -> (decimal integer string=w2850:string)  [unwired: 1 in]
                                n820 = Number To Decimal String(number=w2819) -> (decimal integer string=w2852:string)  [unwired: 1 in]
                                n821 = local read "Data log path and filename"() -> (w2818:path)
                                n822 = Get Date/Time String(want seconds? (F)=TRUE) -> (date string=w2826:string, time string=w2827:string)  [unwired: 2 in]
                                n823 = Number To Decimal String(number=w2810) -> (decimal integer string=w2815:string)  [unwired: 1 in]
                                n824 = Concatenate Strings(w2815, w2816, w2826, "   " ("string"), w2827, w2816, "H1 Alarming, H2 Nominal", w2816, w2835, w2816, "H1 Low Yield Alarm Limit: ", w2837, ", H1 yield = ", w2839, w2816, "H1 Low UPH Alarm Limit: ", w2841, ", H1 UPH = ", w2843, w2816, w2844, w2816, "H2 Low Yield Warning Limit: ", w2846, ", H2 yield = ", w2848, w2816, "H2 Low UPH Warning Limit: ", w2850, ", H2 UPH = ", w2852, w2816, w2816) -> (w2824:string)
                                n825 = call "SentinelDatalog.vi"("operation (0:open)"=T10."open", "String"=w2824, "data log path"=w2818) -> ()  [unwired: 8 in, 1 out]
                                }
                                frame "H1AH2W" {
                                w2863 = "\r\n"
                                n826 = local read "H1 online"() -> (w2880:bool)
                                n827 = local read "H2 online"() -> (w2881:bool)
                                n828 = local read "H2 UPH warning limit hid"() -> (w2878:dbl)
                                n829 = local read "H2  low yield warning"() -> (w2877:dbl)
                                n830 = local read "H1 UPH alarm limit hid"() -> (w2876:dbl)
                                n831 = local read "H1 low yield alarm"() -> (w2875:dbl)
                                n832 = local read "H1 UPH"() -> (w2869:cluster{u32, u32})
                                n833 = local read "H2 UPH"() -> (w2868:cluster{u32, u32})
                                n834 = local read "YieldMon"() -> (w2861:cluster{i32, i32, i32, i32})
                                n835 = local read "YieldMon"() -> (w2859:cluster{i32, i32, i32, i32})
                                n836 = case shown="True" w2880 {
                                tunnel: ["H1 Off-Line" "H1 On-Line"] -> w2882
                                frame False {
                                }
                                frame True {
                                }
                                }
                                n837 = case shown="True" w2881 {
                                tunnel: ["H2 Off-Line" "H2 On-Line"] -> w2891
                                frame False {
                                }
                                frame True {
                                }
                                }
                                n838 = local read "Number of data log entries hid"() -> (w2857:u32)
                                n839 = Unbundle(w2861) -> (w2860:i32)  [unwired: 3 out]
                                n840 = Unbundle(w2869) -> (w2867:u32)  [unwired: 1 out]
                                n841 = Unbundle(w2859) -> (w2858:i32)  [unwired: 3 out]
                                n842 = Unbundle(w2868) -> (w2866:u32)  [unwired: 1 out]
                                n843 = Number To Decimal String(number=w2875) -> (decimal integer string=w2884:string)  [unwired: 1 in]
                                n844 = Number To Decimal String(number=w2860) -> (decimal integer string=w2886:string)  [unwired: 1 in]
                                n845 = Number To Decimal String(number=w2876) -> (decimal integer string=w2888:string)  [unwired: 1 in]
                                n846 = Number To Decimal String(number=w2867) -> (decimal integer string=w2890:string)  [unwired: 1 in]
                                n847 = Number To Decimal String(number=w2877) -> (decimal integer string=w2893:string)  [unwired: 1 in]
                                n848 = Number To Decimal String(number=w2858) -> (decimal integer string=w2895:string)  [unwired: 1 in]
                                n849 = Number To Decimal String(number=w2878) -> (decimal integer string=w2897:string)  [unwired: 1 in]
                                n850 = Number To Decimal String(number=w2866) -> (decimal integer string=w2899:string)  [unwired: 1 in]
                                n851 = local read "Data log path and filename"() -> (w2865:path)
                                n852 = Get Date/Time String(want seconds? (F)=TRUE) -> (date string=w2873:string, time string=w2874:string)  [unwired: 2 in]
                                n853 = Number To Decimal String(number=w2857) -> (decimal integer string=w2862:string)  [unwired: 1 in]
                                n854 = Concatenate Strings(w2862, w2863, w2873, "   " ("string"), w2874, w2863, "H1 Alarming, H2 Warning", w2863, w2882, w2863, "H1 Low Yield Alarm Limit: ", w2884, ", H1 yield = ", w2886, w2863, "H1 Low UPH Alarm Limit: ", w2888, ", H1 UPH = ", w2890, w2863, w2891, w2863, "H2 Low Yield Warning Limit: ", w2893, ", H2 yield = ", w2895, w2863, "H2 Low UPH Warning Limit: ", w2897, ", H2 UPH = ", w2899, w2863) -> (w2871:string)
                                n855 = call "SentinelDatalog.vi"("operation (0:open)"=T10."open", "String"=w2871, "data log path"=w2865) -> ()  [unwired: 8 in, 1 out]
                                }
                                frame "H1AH2A" {
                                w2910 = "\r\n"
                                n856 = local read "H1 online"() -> (w2927:bool)
                                n857 = local read "H2 online"() -> (w2928:bool)
                                n858 = local read "H1 UPH alarm limit hid"() -> (w2923:dbl)
                                n859 = local read "H2 UPH alarm limit hid"() -> (w2925:dbl)
                                n860 = local read "H1 low yield alarm"() -> (w2922:dbl)
                                n861 = local read "H1 UPH"() -> (w2916:cluster{u32, u32})
                                n862 = local read "H2 low yield alarm"() -> (w2924:dbl)
                                n863 = local read "H2 UPH"() -> (w2915:cluster{u32, u32})
                                n864 = local read "YieldMon"() -> (w2908:cluster{i32, i32, i32, i32})
                                n865 = local read "YieldMon"() -> (w2907:cluster{i32, i32, i32, i32})
                                n866 = case shown="True" w2927 {
                                tunnel: ["H1 Off-Line" "H1 On-Line"] -> w2929
                                frame False {
                                }
                                frame True {
                                }
                                }
                                n867 = case shown="True" w2928 {
                                tunnel: ["H2 Off-Line" "H2 On-Line"] -> w2938
                                frame False {
                                }
                                frame True {
                                }
                                }
                                n868 = local read "Number of data log entries hid"() -> (w2904:u32)
                                n869 = Unbundle(w2908) -> (w2905:i32)  [unwired: 3 out]
                                n870 = Unbundle(w2916) -> (w2914:u32)  [unwired: 1 out]
                                n871 = Unbundle(w2907) -> (w2906:i32)  [unwired: 3 out]
                                n872 = Unbundle(w2915) -> (w2913:u32)  [unwired: 1 out]
                                n873 = Number To Decimal String(number=w2922) -> (decimal integer string=w2931:string)  [unwired: 1 in]
                                n874 = Number To Decimal String(number=w2905) -> (decimal integer string=w2933:string)  [unwired: 1 in]
                                n875 = Number To Decimal String(number=w2923) -> (decimal integer string=w2935:string)  [unwired: 1 in]
                                n876 = Number To Decimal String(number=w2914) -> (decimal integer string=w2937:string)  [unwired: 1 in]
                                n877 = Number To Decimal String(number=w2924) -> (decimal integer string=w2940:string)  [unwired: 1 in]
                                n878 = Number To Decimal String(number=w2906) -> (decimal integer string=w2942:string)  [unwired: 1 in]
                                n879 = Number To Decimal String(number=w2925) -> (decimal integer string=w2944:string)  [unwired: 1 in]
                                n880 = Number To Decimal String(number=w2913) -> (decimal integer string=w2946:string)  [unwired: 1 in]
                                n881 = local read "Data log path and filename"() -> (w2912:path)
                                n882 = Get Date/Time String(want seconds? (F)=TRUE) -> (date string=w2920:string, time string=w2921:string)  [unwired: 2 in]
                                n883 = Number To Decimal String(number=w2904) -> (decimal integer string=w2909:string)  [unwired: 1 in]
                                n884 = Concatenate Strings(w2909, w2910, w2920, "   " ("string"), w2921, w2910, "H1 Alarming, H2 Alarming", w2910, w2929, w2910, "H1 Low Yield Alarm Limit: ", w2931, ", H1 yield = ", w2933, w2910, "H1 Low UPH Alarm Limit: ", w2935, ", H1 UPH = ", w2937, w2910, w2938, w2910, "H2 Low Yield Alarm Limit: ", w2940, ", H2 yield = ", w2942, w2910, "H2 Low UPH Alarm Limit: ", w2944, ", H2 UPH = ", w2946, w2910, w2910) -> (w2918:string)
                                n885 = call "SentinelDatalog.vi"("operation (0:open)"=T10."open", "String"=w2918, "data log path"=w2912) -> ()  [unwired: 8 in, 1 out]
                                }
                                }
                                }
                                frame #2 {
                                n886 = Wait (ms)(milliseconds to wait=u32 100) -> ()  [unwired: 1 out]
                                }
                                frame #3 {
                                n887 = local read "Enable electronic notification of alarms"() -> (w2952:bool)
                                n888 = case shown="True" w2952 {
                                frame False {
                                }
                                frame True {
                                n889 = stacked-sequence {
                                frame #0 {
                                # "Email"
                                n890 = local read "Enable email notification"() -> (w2955:bool)
                                n891 = local read "Number of email alerts"() -> (w2954:u32)
                                n892 = Increment(x=w2954) -> (x+1=w2953:u32)
                                n893 = local write "Number of email alerts"(w2953) -> ()
                                n894 = case shown="True" w2955 {
                                frame False {
                                }
                                frame True {
                                n895 = flat-sequence {
                                tunnel: [w2962] -> w2957
                                tunnel: [w2970] -> w2956
                                tunnel: w2957 -> [w2970]
                                tunnel: w2956 -> [w2971]
                                frame #0 {
                                n896 = local read "Data log path and filename"() -> (w2967:path)
                                n897 = local read "Number of email alerts"() -> (w2961:u32)
                                n898 = Number To Decimal String(number=w2961) -> (decimal integer string=w2960:string)  [unwired: 1 in]
                                n899 = Strip Path(path=w2967) -> (stripped path=w2965:path, name=w2959:string)
                                n900 = Path To String(path=w2965) -> (string=w2964:string)
                                n901 = Concatenate Strings(w2964, "\\sent_#" ("string"), w2960, "_" ("string"), w2959) -> (w2968:string)
                                n902 = String To Path(string=w2968) -> (path=w2963:path)
                                n903 = Copy(10:w2963, 11:w2967) -> (3:w2962:path)  [unwired: 3 in, 2 out]
                                }
                                frame #1 {
                                n904 = Wait (ms)(milliseconds to wait=u32 1000) -> ()  [unwired: 1 out]
                                }
                                frame #2 {
                                n905 = local read "Email alert - engineer"() -> (w2973:string)
                                n906 = local read "Email alert - CC"() -> (w2972:string)
                                n907 = local read "Email alert - message"() -> (w2974:string)
                                n908 = call "email_alert.vi"("Email Alert - Message"=w2974, "Email Alert - Engineer"=w2973, "Email Alert - CC"=w2972, "Email ALert - Attachment"=w2971) -> ()  [unwired: 8 in]
                                }
                                }
                                }
                                }
                                }
                                frame #1 {
                                n909 = Wait (ms)(milliseconds to wait=u32 200) -> ()  [unwired: 1 out]
                                }
                                frame #2 {
                                # "text"
                                n910 = local read "Enable text notification"() -> (w2976:bool)
                                n911 = case shown="True" w2976 {
                                frame False {
                                }
                                frame True {
                                n912 = local read "Number of text alerts"() -> (w2980:u32)
                                n913 = Increment(x=w2980) -> (x+1=w2979:u32)
                                n914 = local write "Number of text alerts"(w2979) -> ()
                                n915 = local read "Number of email alerts"() -> (w2989:u32)
                                n916 = local read "Carrier"() -> (w2982:enum16{"T-Mobile", "AT&T", "Verizon", "Sprint"})
                                n917 = local read "Phone number"() -> (w2981:string)
                                n918 = local read "Body"() -> (w2978:string)
                                n919 = local read "Lot number"() -> (w2983:string)
                                n920 = local read "Subject"() -> (w2977:string)
                                n921 = Number To Decimal String(number=w2989) -> (decimal integer string=w2985:string)  [unwired: 1 in]
                                n922 = Concatenate Strings(w2978, ", # " ("string"), w2985, ", Lot Number: " ("string"), w2983) -> (w2990:string)
                                n923 = local write "Notifications Lot Display"(w2983) -> ()
                                n924 = call <userlib>:"Send SMS 2009.vi"("Body"=w2990, "Carrier"=w2982, "Subject"=w2977, "phone number"=w2981, "smtp server"="smtp.gmail.com", "password"="sentinelcontroller", "email username"="sentinelcontroller@gmail.com") -> ("Error Out"=w2988:errorcluster)  [unwired: 4 in]
                                n925 = Unbundle By Name(w2988) -> ("status"=w2987:bool)
                                n926 = case shown="True" w2987 {
                                frame False {
                                }
                                frame True {
                                n927 = One Button Dialog(message="Warning:\nError sending text message!\nTry changing the settings or\nswitch to email method", button name ("OK")="Dismiss") -> ()  [unwired: 1 out]
                                }
                                }
                                }
                                }
                                }
                                }
                                }
                                }
                                }
                                frame #4 {
                                n928 = Wait (ms)(milliseconds to wait=u32 100) -> ()  [unwired: 1 out]
                                }
                              }
                            }
                          }
                        }
                      }
                    }
                  }
                }
              }
              n929 = Wait (ms)(milliseconds to wait=u32 100) -> ()  [unwired: 1 out]
            }
            n930 = local read "Yield averaging"() -> (w350:u32)
            n931 = local read "UPH averaging"() -> (w349:u32)
            n932 = local read "Yield averaging"() -> (w351:u32)
            n933 = local read "UPH averaging"() -> (w352:u32)
            n934 = Initialize Array(w347, w350) -> (w348:i32[])
            n935 = Initialize Array(w346, w349) -> (w345:dbl[])
            n936 = Initialize Array(w354, w351) -> (w353:i32[])
            n937 = Initialize Array(w355, w352) -> (w356:dbl[])
            n938 = while {
              shift-right: [w2259] -> _
              shift-left: w346 -> [w2265]
              shift-right: [w2260] -> _
              shift-left: w345 -> [w2264]
              shift-right: [w2261] -> _
              shift-left: w347 -> [w2258]
              shift-right: [w2262] -> _
              shift-left: w348 -> [w2263]
              stop <- w2256 stop-if-true
              # "if there is now a lock, it is unlikely that the test time is going to be less than 100ms,\nso this is a relatively slow loop"
              n939 = local read "H2 Lock"() -> (w2255:bool)
              n940 = Wait (ms)(milliseconds to wait=u32 50) -> ()  [unwired: 1 out]
              n941 = case shown="True" w2255 {
                tunnel: w2265 -> [w2270 w2295]
                tunnel: w2264 -> [w2269 w2290]
                tunnel: w2263 -> [w2267 w2287]
                tunnel: [w2267 w2281] -> w2262
                tunnel: [w2268 w2279] -> w2261
                tunnel: [w2269 w2278] -> w2260
                tunnel: [w2270 w2277] -> w2259
                tunnel: w2258 -> [w2268 w2276]
                frame False {
                  n942 = local write "Calc H1 UPH"(u32 0 ("Sim H1 UPH")) -> ()
                }
                frame True {
                  n943 = flat-sequence {
                    tunnel: w2287 -> [w2298]
                    tunnel: w2276 -> [w2299]
                    tunnel: w2290 -> [w2300]
                    tunnel: w2295 -> [w2301]
                    tunnel: [w2301] -> w2286
                    tunnel: [w2300] -> w2285
                    tunnel: [w2299] -> w2284
                    tunnel: [w2298] -> w2283
                    tunnel: [w2314] -> w2294
                    tunnel: [w2313] -> w2291
                    tunnel: [w2312] -> w2289
                    tunnel: [w2311] -> w2288
                    tunnel: w2286 -> [w2314]
                    tunnel: w2285 -> [w2313]
                    tunnel: w2284 -> [w2312]
                    tunnel: w2283 -> [w2311]
                    tunnel: w2294 -> [w2340]
                    tunnel: [w2340] -> w2293
                    tunnel: [w2339] -> w2292
                    tunnel: w2291 -> [w2339]
                    tunnel: w2289 -> [w2329]
                    tunnel: w2288 -> [w2328]
                    tunnel: [w2327] -> w2282
                    tunnel: [w2326] -> w2280
                    tunnel: w2293 -> [w2366]
                    tunnel: w2292 -> [w2367]
                    tunnel: w2282 -> [w2385]
                    tunnel: w2280 -> [w2384]
                    tunnel: [w2385] -> w2275
                    tunnel: [w2384] -> w2274
                    tunnel: [w2363] -> w2273
                    tunnel: [w2362] -> w2272
                    tunnel: [w2400] -> w2277
                    tunnel: [w2401] -> w2278
                    tunnel: [w2402] -> w2279
                    tunnel: [w2403] -> w2281
                    tunnel: w2275 -> [w2403]
                    tunnel: w2274 -> [w2402]
                    tunnel: w2273 -> [w2401]
                    tunnel: w2272 -> [w2400]
                    frame #0 {
                      n944 = local read "H2 loop counter hid"() -> (w2296:u32)
                      n945 = Equal To 0?(x=w2296) -> (x = 0?=w2297:bool)
                      n946 = case shown="True" w2297 {
                        frame False {
                        }
                        frame True {
                          # "H2 first pass init"
                          n947 = local write "H2 Device Count"(0.0 ("H2 Device Count")) -> ()
                          n948 = local write "H2 measured  Index Time"(0.0 ("H2 Index Time")) -> ()
                          n949 = local write "H2 measured Test Time"(0.0 ("H2 Test Time")) -> ()
                          n950 = local write "H2 measured Wait Time"(0.0 ("H2 Wait Time")) -> ()
                          n951 = local read "H2 low UPH alarm (%)"() -> (w2305:dbl)
                          n952 = Divide(x=w2305, y=100.0) -> (x/y=w2304:dbl)
                          n953 = Bundle(0.0, w2304) -> (w2302:cluster{dbl, dbl})  [unwired: 1 in]
                          n954 = local write "H2 UPH"(w2302) -> ()
                        }
                      }
                    }
                    frame #1 {
                      # "H2 testing"
                      n955 = while {
                        stop <- w2318 stop-if-true
                        n956 = local read "H2 Lock"() -> (w2322:bool)
                        n957 = local read "POWER"() -> (w2317:bool)
                        n958 = local read "Run"() -> (w2315:bool)
                        n959 = Not(x=w2322) -> (.not. x?=w2316:bool)
                        n960 = Not(x=w2317) -> (.not. x?=w2320:bool)
                        n961 = Not(x=w2315) -> (.not. x?=w2319:bool)
                        n962 = Compound Arithmetic op=OR(w2316, w2320, w2319) -> (w2318:bool)
                        n963 = Wait (ms)(milliseconds to wait=u32 1) -> ()  [unwired: 1 out]
                      }
                    }
                    frame #2 {
                      n964 = local read "H2 cycle yield hid"() -> (w2323:dbl)
                      n965 = local read "H2 loop counter hid"() -> (w2324:u32)
                      n966 = local read "Yield averaging"() -> (w2325:u32)
                      n967 = local read "H2 low yield alarm"() -> (w2338:dbl)
                      n968 = local read "YieldMon"() -> (w2331:cluster{i32, i32, i32, i32})
                      n969 = local read "H2  low yield warning"() -> (w2337:dbl)
                      n970 = call "moving_avg_core.vi"("Array in"=w2328, "avg"=w2325, "accumulator in"=w2329, "i"=w2324, "data in"=w2323) -> ("Array out"=w2327:dbl[], "accumulator out"=w2326:dbl, "rolling avg out"=w2332:dbl)  [unwired: 4 in]
                      n971 = Unbundle(w2331) -> (w2330:i32)  [unwired: 3 out]
                      n972 = Less?(x=w2332, y=w2337) -> (x < y?=w2336:bool)
                      n973 = case shown="True" w2336 {
                        tunnel: w2332 -> [_ w2345]
                        tunnel: w2338 -> [_ w2344]
                        frame False {
                          n974 = local write "H2 nominal"(TRUE ("H1 nominal")) -> ()
                          n975 = local write "H2 warning"(FALSE ("H1 warning")) -> ()
                          n976 = local write "H2 alarm"(FALSE ("H1 warning")) -> ()
                        }
                        frame True {
                          n977 = Less?(x=w2345, y=w2344) -> (x < y?=w2346:bool)
                          n978 = case shown="True" w2346 {
                            frame False {
                              n979 = local write "H2 nominal"(FALSE ("H1 nominal")) -> ()
                              n980 = local write "H2 warning"(TRUE ("H1 warning")) -> ()
                              n981 = local write "H2 alarm"(FALSE ("H1 warning")) -> ()
                            }
                            frame True {
                              n982 = local read "H2 enable halt\non yield alarm"() -> (w2350:bool)
                              n983 = local write "H2 nominal"(FALSE ("H1 nominal")) -> ()
                              n984 = local write "H2 alarm"(TRUE ("H1 warning")) -> ()
                              n985 = local write "H2 warning"(FALSE ("H1 warning")) -> ()
                              n986 = case shown="True" w2350 {
                                frame False {
                                }
                                frame True {
                                n987 = local write "H2 online"(FALSE ("H1 Online")) -> ()
                                }
                              }
                            }
                          }
                        }
                      }
                      n988 = local read "H1 low yield alarm"() -> (w2335:dbl)
                      n989 = local read "H2 low yield alarm"() -> (w2334:dbl)
                      n990 = Bundle(w2330, "rolling avg out"=w2332, "H1 low yield alarm"=w2335, "H2 low yield alarm"=w2334) -> (w2333:T12)  [unwired: 1 in]
                      n991 = local write "YieldMon"(w2333) -> ()
                    }
                    frame #3 {
                      n992 = local read "H2 measured  Index Time"() -> (w2356:dbl)
                      n993 = local read "H2 measured Wait Time"() -> (w2355:dbl)
                      n994 = local read "H2 measured Test Time"() -> (w2357:dbl)
                      n995 = local read "H2 parallelism"() -> (w2369:u32)
                      n996 = local read "H2 lot yield mon"() -> (w2383:dbl)
                      n997 = local write "H2 IT (scycle)"(w2356) -> ()
                      n998 = local write "H2 TT (s/cycle)"(w2357) -> ()
                      n999 = local write "H2 WT (s/cycle)"(w2355) -> ()
                      n1000 = Compound Arithmetic op=ADD(w2356, w2357, w2355) -> (w2372:dbl)
                      n1001 = Compound Arithmetic op=ADD(w2356, w2357) -> (w2368:dbl)
                      n1002 = Multiply(x=w2369, y=3600.0 ("x")) -> (x*y=w2371:dbl)
                      n1003 = Divide(x=w2371, y=w2372) -> (x/y=w2382:dbl)
                      n1004 = Divide(x=w2383, y=w2368) -> (x/y=w2361:dbl)
                      n1005 = local write "H2 Single Handler UPH hid"(w2361) -> ()
                      n1006 = local read "H2 low UPH warning (%)"() -> (w2379:dbl)
                      n1007 = local read "H2 loop counter hid"() -> (w2365:u32)
                      n1008 = local read "Yield averaging"() -> (w2364:u32)
                      n1009 = local read "H2 low UPH alarm (%)"() -> (w2374:dbl)
                      n1010 = property on="H2 UPH" class="Knob (strict)"() -> ("Scale.Maximum"=w2380:dbl)  [unwired: 2 in, 2 out]
                      n1011 = Divide(x=w2379, y=100.0) -> (x/y=w2378:dbl)
                      n1012 = call "moving_avg_core.vi"("Array in"=w2367, "avg"=w2364, "accumulator in"=w2366, "i"=w2365, "data in"=w2382) -> ("Array out"=w2363:dbl[], "accumulator out"=w2362:dbl, "rolling avg out"=w2381:dbl)  [unwired: 4 in]
                      n1013 = Multiply(x=w2380, y=w2378) -> (x*y=w2360:dbl)
                      n1014 = Divide(x=w2374, y=100.0) -> (x/y=w2376:dbl)
                      n1015 = local write "H2 UPH warning limit hid"(w2360) -> ()
                      n1016 = Less?(x=w2381, y=w2360) -> (x < y?=w2373:bool)
                      n1017 = Multiply(x=w2380, y=w2376) -> (x*y=w2359:dbl)
                      n1018 = case shown="True" w2373 {
                        tunnel: w2381 -> [_ w2390]
                        tunnel: w2359 -> [_ w2389]
                        frame False {
                          n1019 = local write "H2 nominal 2"(TRUE ("H1 nominal")) -> ()
                          n1020 = local write "H2 warning 2"(FALSE ("H1 warning")) -> ()
                          n1021 = local write "H2 alarm 2"(FALSE ("H1 warning")) -> ()
                        }
                        frame True {
                          n1022 = Less?(x=w2390, y=w2389) -> (x < y?=w2391:bool)
                          n1023 = case shown="True" w2391 {
                            frame False {
                              n1024 = local write "H2 nominal 2"(FALSE ("H1 nominal")) -> ()
                              n1025 = local write "H2 warning 2"(TRUE ("H1 warning")) -> ()
                              n1026 = local write "H2 alarm 2"(FALSE ("H1 warning")) -> ()
                            }
                            frame True {
                              n1027 = local read "H2 enable halt\non UPH alarm"() -> (w2395:bool)
                              n1028 = local write "H2 alarm 2"(TRUE ("H1 warning")) -> ()
                              n1029 = local write "H2 warning 2"(FALSE ("H1 warning")) -> ()
                              n1030 = local write "H2 nominal 2"(FALSE ("H1 nominal")) -> ()
                              n1031 = case shown="True" w2395 {
                                frame False {
                                }
                                frame True {
                                n1032 = local write "H2 online"(FALSE ("H1 Online")) -> ()
                                }
                              }
                            }
                          }
                        }
                      }
                      n1033 = local write "H2 UPH alarm limit hid"(w2359) -> ()
                      n1034 = Bundle("rolling avg out"=w2381, w2359) -> (w2358:cluster{"rolling avg out":dbl, dbl})  [unwired: 1 in]
                      n1035 = local write "H2 UPH"(w2358) -> ()
                    }
                    frame #4 {
                      n1036 = while {
                        stop <- w2405 continue-if-true
                        n1037 = local read "H2 Lock"() -> (w2405:bool)
                        n1038 = Wait (ms)(milliseconds to wait=u32 10) -> ()  [unwired: 1 out]
                      }
                    }
                  }
                }
              }
              n1039 = local read "POWER"() -> (w2257:bool)
              n1040 = Not(x=w2257) -> (.not. x?=w2256:bool)
            }
            n1041 = while {
              shift-right: [w3136] -> _
              shift-left: w355 -> [w3139]
              shift-right: [w3137] -> _
              shift-left: w356 -> [w3138]
              shift-right: [w3132] -> _
              shift-left: w354 -> [w3135]
              shift-right: [w3133] -> _
              shift-left: w353 -> [w3134]
              stop <- w3131 stop-if-true
              # "if there is now a lock, it is unlikely that the test time is going to be less than 100ms,\nso this is a relatively slow loop"
              n1042 = local read "H1 Lock"() -> (w3130:bool)
              n1043 = case shown="True" w3130 {
                tunnel: w3139 -> [w3145 w3170]
                tunnel: w3138 -> [w3144 w3165]
                tunnel: [w3144 w3164] -> w3137
                tunnel: [w3145 w3163] -> w3136
                tunnel: w3135 -> [w3143 w3161]
                tunnel: w3134 -> [w3142 w3159]
                tunnel: [w3142 w3157] -> w3133
                tunnel: [w3143 w3155] -> w3132
                frame False {
                  n1044 = local write "Calc H1 UPH"(u32 0 ("Sim H1 UPH")) -> ()
                }
                frame True {
                  n1045 = flat-sequence {
                    tunnel: w3159 -> [w3173]
                    tunnel: w3161 -> [w3174]
                    tunnel: w3165 -> [w3175]
                    tunnel: w3170 -> [w3176]
                    tunnel: [w3176] -> w3154
                    tunnel: [w3175] -> w3153
                    tunnel: [w3174] -> w3152
                    tunnel: [w3173] -> w3151
                    tunnel: [w3189] -> w3169
                    tunnel: [w3188] -> w3166
                    tunnel: [w3187] -> w3162
                    tunnel: [w3186] -> w3160
                    tunnel: w3154 -> [w3189]
                    tunnel: w3153 -> [w3188]
                    tunnel: w3152 -> [w3187]
                    tunnel: w3151 -> [w3186]
                    tunnel: w3169 -> [w3204]
                    tunnel: [w3204] -> w3168
                    tunnel: [w3203] -> w3167
                    tunnel: w3166 -> [w3203]
                    tunnel: w3162 -> [w3202]
                    tunnel: w3160 -> [w3201]
                    tunnel: [w3200] -> w3158
                    tunnel: [w3199] -> w3156
                    tunnel: w3168 -> [w3242]
                    tunnel: w3167 -> [w3241]
                    tunnel: w3158 -> [w3238]
                    tunnel: w3156 -> [w3237]
                    tunnel: [w3240] -> w3150
                    tunnel: [w3239] -> w3149
                    tunnel: [w3238] -> w3148
                    tunnel: [w3237] -> w3147
                    tunnel: [w3277] -> w3155
                    tunnel: [w3278] -> w3157
                    tunnel: [w3279] -> w3163
                    tunnel: [w3280] -> w3164
                    tunnel: w3150 -> [w3280]
                    tunnel: w3149 -> [w3279]
                    tunnel: w3148 -> [w3278]
                    tunnel: w3147 -> [w3277]
                    frame #0 {
                      n1046 = local read "H1 loop counter hid"() -> (w3172:u32)
                      n1047 = Equal To 0?(x=w3172) -> (x = 0?=w3171:bool)
                      n1048 = case shown="True" w3171 {
                        frame False {
                        }
                        frame True {
                          n1049 = local read "H1 low UPH alarm (%)"() -> (w3181:dbl)
                          n1050 = local write "H1 measured Index Time"(0.0 ("H1 Index Time")) -> ()
                          n1051 = local write "H1 measured Wait Time"(0.0 ("H1 Wait Time")) -> ()
                          n1052 = local write "H1 Device Count"(0.0 ("H1 Device Count")) -> ()
                          n1053 = local write "H1 measured Test Time"(0.0 ("H1 Test Time")) -> ()
                          n1054 = Divide(x=w3181, y=100.0) -> (x/y=w3179:dbl)
                          n1055 = Bundle("y"=0.0, w3179) -> (w3177:cluster{"y":dbl, dbl})  [unwired: 1 in]
                          n1056 = local write "H1 UPH"(w3177) -> ()
                        }
                      }
                    }
                    frame #1 {
                      # "H1 testing"
                      n1057 = while {
                        stop <- w3193 stop-if-true
                        n1058 = local read "H1 Lock"() -> (w3197:bool)
                        n1059 = local read "POWER"() -> (w3191:bool)
                        n1060 = local read "Run"() -> (w3190:bool)
                        n1061 = Wait (ms)(milliseconds to wait=u32 1) -> ()  [unwired: 1 out]
                        n1062 = Not(x=w3197) -> (.not. x?=w3192:bool)
                        n1063 = Not(x=w3191) -> (.not. x?=w3195:bool)
                        n1064 = Not(x=w3190) -> (.not. x?=w3194:bool)
                        n1065 = Compound Arithmetic op=OR(w3192, w3195, w3194) -> (w3193:bool)
                      }
                    }
                    frame #2 {
                      n1066 = local read "H1 cycle yield hid"() -> (w3207:dbl)
                      n1067 = local read "H1 loop counter hid"() -> (w3206:u32)
                      n1068 = local read "Yield averaging"() -> (w3205:u32)
                      n1069 = local read "H1 low yield warning"() -> (w3215:dbl)
                      n1070 = local read "H1 low yield alarm"() -> (w3213:dbl)
                      n1071 = call "moving_avg_core.vi"("Array in"=w3201, "avg"=w3205, "accumulator in"=w3202, "i"=w3206, "data in"=w3207) -> ("Array out"=w3200:dbl[], "accumulator out"=w3199:dbl, "rolling avg out"=w3210:dbl)  [unwired: 4 in]
                      n1072 = Less?(x=w3210, y=w3215) -> (x < y?=w3214:bool)
                      n1073 = case shown="True" w3214 {
                        tunnel: w3210 -> [_ w3221]
                        tunnel: w3213 -> [_ w3220]
                        frame False {
                          n1074 = local write "H1 alarm"(FALSE ("H1 warning")) -> ()
                          n1075 = local write "H1 warning"(FALSE ("H1 warning")) -> ()
                          n1076 = local write "H1 nominal"(TRUE ("H1 nominal")) -> ()
                        }
                        frame True {
                          n1077 = Less?(x=w3221, y=w3220) -> (x < y?=w3219:bool)
                          n1078 = case shown="True" w3219 {
                            frame False {
                              n1079 = local write "H1 alarm"(FALSE ("H1 warning")) -> ()
                              n1080 = local write "H1 warning"(TRUE ("H1 warning")) -> ()
                              n1081 = local write "H1 nominal"(FALSE ("H1 nominal")) -> ()
                            }
                            frame True {
                              n1082 = local read "H1 enable halt\non yield alarm"() -> (w3225:bool)
                              n1083 = local write "H1 nominal"(FALSE ("H1 nominal")) -> ()
                              n1084 = local write "H1 warning"(FALSE ("H1 warning")) -> ()
                              n1085 = local write "H1 alarm"(TRUE ("H1 warning")) -> ()
                              n1086 = case shown="True" w3225 {
                                frame False {
                                }
                                frame True {
                                n1087 = local write "H1 online"(FALSE ("H1 Online")) -> ()
                                }
                              }
                            }
                          }
                        }
                      }
                      n1088 = local read "YieldMon"() -> (w3209:cluster{i32, i32, i32, i32})
                      n1089 = local read "H1 low yield alarm"() -> (w3212:dbl)
                      n1090 = local read "H2 low yield alarm"() -> (w3211:dbl)
                      n1091 = Unbundle(w3209) -> (w3198:i32)  [unwired: 3 out]
                      n1092 = Bundle("rolling avg out"=w3210, w3198, "H1 low yield alarm"=w3212, "H2 low yield alarm"=w3211) -> (w3208:T13)  [unwired: 1 in]
                      n1093 = local write "YieldMon"(w3208) -> ()
                    }
                    frame #3 {
                      n1094 = local read "H1 measured Index Time"() -> (w3232:dbl)
                      n1095 = local read "H1 measured Wait Time"() -> (w3230:dbl)
                      n1096 = local read "H1 measured Test Time"() -> (w3231:dbl)
                      n1097 = local read "H1 parallelism"() -> (w3249:u32)
                      n1098 = local read "H1 loop counter hid"() -> (w3244:u32)
                      n1099 = local read "UPH averaging"() -> (w3243:u32)
                      n1100 = local read "H1 low UPH warning (%)"() -> (w3253:dbl)
                      n1101 = local write "H1 IT (s/cycle)"(w3232) -> ()
                      n1102 = local write "H1 TT (s/cycle)"(w3231) -> ()
                      n1103 = local write "H1 WT (s/cycle)"(w3230) -> ()
                      n1104 = Compound Arithmetic op=ADD(w3232, w3231, w3230) -> (w3245:dbl)
                      n1105 = Compound Arithmetic op=ADD(w3232, w3231) -> (w3252:dbl)
                      n1106 = Multiply(x=w3249, y=u32 3600 ("x")) -> (x*y=w3251:u32)
                      n1107 = Divide(x=w3251, y=w3252) -> (x/y=w3235:dbl)
                      n1108 = local read "H1 low UPH alarm (%)"() -> (w3258:dbl)
                      n1109 = local write "H1 Single Handler UPH hid"(w3235) -> ()
                      n1110 = property on="H1 UPH" class="Knob (strict)"() -> ("Scale.Maximum"=w3260:dbl)  [unwired: 2 in, 2 out]
                      n1111 = Divide(x=w3253, y=100.0) -> (x/y=w3254:dbl)
                      n1112 = Multiply(x=w3260, y=w3254) -> (x*y=w3233:dbl)
                      n1113 = Divide(x=w3258, y=100.0) -> (x/y=w3256:dbl)
                      n1114 = local write "H1 UPH warning limit hid"(w3233) -> ()
                      n1115 = Multiply(x=w3260, y=w3256) -> (x*y=w3234:dbl)
                      n1116 = local write "H1 UPH alarm limit hid"(w3234) -> ()
                      n1117 = local read "H1 parallelism"() -> (w3248:u32)
                      n1118 = Multiply(x=w3248, y=u32 3600 ("x")) -> (x*y=w3246:u32)
                      n1119 = Divide(x=w3246, y=w3245) -> (x/y=w3262:dbl)
                      n1120 = call "moving_avg_core.vi"("Array in"=w3241, "avg"=w3243, "accumulator in"=w3242, "i"=w3244, "data in"=w3262) -> ("Array out"=w3240:dbl[], "accumulator out"=w3239:dbl, "rolling avg out"=w3261:dbl)  [unwired: 4 in]
                      n1121 = Less?(x=w3261, y=w3233) -> (x < y?=w3259:bool)
                      n1122 = case shown="True" w3259 {
                        tunnel: w3261 -> [_ w3267]
                        tunnel: w3234 -> [_ w3266]
                        frame False {
                          n1123 = local write "H1 alarm 2"(FALSE ("H1 warning")) -> ()
                          n1124 = local write "H1 nominal 2"(TRUE ("H1 nominal")) -> ()
                          n1125 = local write "H1 warning 2"(FALSE ("H1 warning")) -> ()
                        }
                        frame True {
                          n1126 = Less?(x=w3267, y=w3266) -> (x < y?=w3268:bool)
                          n1127 = case shown="True" w3268 {
                            frame False {
                              n1128 = local write "H1 nominal 2"(FALSE ("H1 nominal")) -> ()
                              n1129 = local write "H1 warning 2"(TRUE ("H1 warning")) -> ()
                              n1130 = local write "H1 alarm 2"(FALSE ("H1 warning")) -> ()
                            }
                            frame True {
                              n1131 = local read "H1 enable halt\non UPH alarm"() -> (w3272:bool)
                              n1132 = local write "H1 warning 2"(FALSE ("H1 warning")) -> ()
                              n1133 = local write "H1 alarm 2"(TRUE ("H1 warning")) -> ()
                              n1134 = local write "H1 nominal 2"(FALSE ("H1 nominal")) -> ()
                              n1135 = case shown="True" w3272 {
                                frame False {
                                }
                                frame True {
                                n1136 = local write "H1 online"(FALSE ("H1 Online")) -> ()
                                }
                              }
                            }
                          }
                        }
                      }
                      n1137 = Bundle("rolling avg out"=w3261, w3234) -> (w3236:cluster{"rolling avg out":dbl, dbl})  [unwired: 1 in]
                      n1138 = local write "H1 UPH"(w3236) -> ()
                    }
                    frame #4 {
                      n1139 = while {
                        stop <- w3282 continue-if-true
                        n1140 = local read "H1 Lock"() -> (w3282:bool)
                        n1141 = Wait (ms)(milliseconds to wait=u32 10) -> ()  [unwired: 1 out]
                      }
                    }
                  }
                }
              }
              n1142 = Wait (ms)(milliseconds to wait=u32 50) -> ()  [unwired: 1 out]
              n1143 = local read "POWER"() -> (w3141:bool)
              n1144 = Not(x=w3141) -> (.not. x?=w3131:bool)
            }
            n1145 = while {
              stop <- w850 continue-if-true
              n1146 = while {
                stop <- w852 stop-if-true
                n1147 = event shown="[1] \"H1 online\": Value Change" {
                  selector: _ -> [_ _]
                  dyn-events: _ -> [_ _]
                  timeout: -1 -> [_ _]
                  tunnel: [_ TRUE] -> w852
                  event Timeout {
                    n1148 = event-data() -> ()  [unwired: 1 in, 2 out]
                  }
                  event "H1 online": Value Change {
                    n1149 = event-data() -> ()  [unwired: 1 in, 5 out]
                    n1150 = local read "Enable data logging of all events"() -> (w853:bool)
                    n1151 = case shown="True" w853 {
                      frame False {
                      }
                      frame True {
                        w857 = "\r\n"
                        n1152 = Get Date/Time String(want seconds? (F)=TRUE) -> (date string=w862:string, time string=w861:string)  [unwired: 2 in]
                        n1153 = local read "H1 online"() -> (w859:bool)
                        n1154 = case shown="False" w859 {
                          tunnel: ["H1 Off-Line" "H1 On-Line"] -> w858
                          frame False {
                          }
                          frame True {
                          }
                        }
                        n1155 = local read "Data log path and filename"() -> (w856:path)
                        n1156 = Concatenate Strings(w862, "   " ("string"), w861, w857, "Change in H1 Status: ", w858, w857, w857) -> (w864:string)
                        n1157 = call "SentinelDatalog.vi"("operation (0:open)"=T10."open", "String"=w864, "data log path"=w856) -> ()  [unwired: 8 in, 1 out]
                      }
                    }
                  }
                }
              }
              n1158 = local read "POWER"() -> (w850:bool)
            }
            n1159 = while {
              stop <- w832 continue-if-true
              n1160 = while {
                stop <- w834 stop-if-true
                n1161 = event shown="[1] \"H2 online\": Value Change" {
                  selector: _ -> [_ _]
                  dyn-events: _ -> [_ _]
                  timeout: -1 -> [_ _]
                  tunnel: [_ TRUE] -> w834
                  event Timeout {
                    n1162 = event-data() -> ()  [unwired: 1 in, 2 out]
                  }
                  event "H2 online": Value Change {
                    n1163 = event-data() -> ()  [unwired: 1 in, 5 out]
                    n1164 = local read "Enable data logging of all events"() -> (w835:bool)
                    n1165 = case shown="True" w835 {
                      frame False {
                      }
                      frame True {
                        w839 = "\r\n"
                        n1166 = local read "H2 online"() -> (w841:bool)
                        n1167 = case shown="False" w841 {
                          tunnel: ["H2 Off-Line" "H2 On-Line"] -> w840
                          frame False {
                          }
                          frame True {
                          }
                        }
                        n1168 = local read "Data log path and filename"() -> (w838:path)
                        n1169 = Get Date/Time String(want seconds? (F)=TRUE) -> (date string=w844:string, time string=w843:string)  [unwired: 2 in]
                        n1170 = Concatenate Strings(w844, "   " ("string"), w843, w839, "Change in H2 Status: ", w840, w839, w839) -> (w846:string)
                        n1171 = call "SentinelDatalog.vi"("operation (0:open)"=T10."open", "String"=w846, "data log path"=w838) -> ()  [unwired: 8 in, 1 out]
                      }
                    }
                  }
                }
              }
              n1172 = local read "POWER"() -> (w832:bool)
            }
            n1173 = while {
              stop <- w980 continue-if-true
              n1174 = local read "Tester online"() -> (w981:bool)
              n1175 = case shown="True" w981 {
                frame False {
                }
                frame True {
                  n1176 = flat-sequence {
                    frame #0 {
                      n1177 = local write "Exit SC handler StMach hid"(FALSE ("Exit tester state machine hid")) -> ()
                      n1178 = local write "SC handler states hid"(SC_handler_states."initializing bus" ("SC virtual handler states")) -> ()
                    }
                    frame #1 {
                      n1179 = flat-sequence {
                        tunnel: [w988] -> w985
                        tunnel: [w987] -> w986
                        frame #0 {
                          w987 = 0.0
                          # "These are consumed in the \"responding to sites\"\nstate when at least one handler has sites ready.  \nIt is executed only after one cycle. At that point,\nthere is at least one test period and one wait period\nto make a utilization calculation."
                          n1180 = local read "Utilization averaging"() -> (w989:i32)
                          n1181 = Initialize Array(w987, w989) -> (w988:dbl[])
                        }
                      }
                      n1182 = while {
                        shift-right: [w996] -> _
                        shift-left: w986 -> [w991]
                        shift-right: [w992] -> _
                        shift-left: w985 -> [w990]
                        stop <- w993 stop-if-true
                        n1183 = flat-sequence {
                          tunnel: [w1002] -> w995
                          tunnel: [w1001] -> w994
                          tunnel: w991 -> [w1000]
                          tunnel: w990 -> [w999]
                          tunnel: [w1781] -> w992
                          tunnel: [w1782] -> w996
                          tunnel: w995 -> [w1782]
                          tunnel: w994 -> [w1781]
                          frame #0 {
                            n1184 = local read "SC handler states hid"() -> (w998:T7)
                            n1185 = case shown="\"responding to BINON\"" w998 {
                              tunnel: w1000 -> [w1003 w1028 w1079 w1108 w1187 w1203 w1238 w1273 w1312 w1348 w1424 w1526 w1628 w1656 w1762 w1773]
                              tunnel: [w1004 w1029 w1080 w1109 w1188 w1204 w1237 w1272 w1309 w1347 w1423 w1525 w1627 w1655 w1761 w1772] -> w1001
                              tunnel: w999 -> [w1004 w1029 w1080 w1109 w1188 w1204 w1237 w1272 w1311 w1347 w1423 w1525 w1627 w1655 w1761 w1772]
                              tunnel: [w1003 w1028 w1079 w1108 w1187 w1203 w1238 w1273 w1310 w1348 w1424 w1526 w1628 w1656 w1762 w1773] -> w1002
                              frame "initializing bus", Default {
                                n1186 = flat-sequence {
                                frame #0 {
                                n1187 = local write "VISA bus 0 close error"(FALSE ("VISA bus 0 close error")) -> ()
                                }
                                frame #1 {
                                w1013 = T14 1073684500 items=["Service Request"=1073684491, "Trigger"=3221168138, "Clear"=1073684493, "VXI Signal"=1073684512, "VXI/VME Interrupt"=3221168161, "VXI/VME Sysfail"=1073684509, "VXI/VME Sysreset"=1073684510, "GPIB CIC"=1073684498, "GPIB Talk"=1073684499, "GPIB Listen"=1073684500, "PXI Interrupt"=1073684514, "Serial Break"=1073684515, "Serial TermChar"=1073684516, "Serial CTS"=1073684521, "Serial DSR"=1073684522, "Serial DCD"=1073684524, "Serial RI"=1073684526, "Serial Character"=1073684533, "USB Interrupt"=1073684535, "All Enabled"=1073709055] ("Event Type")
                                n1188 = local read "SentCtrl listens to tester at"() -> (w1010:refnum<visa-resource-name>)
                                n1189 = local read "GPIB wait timeout hid"() -> (w1008:u32)
                                n1190 = VISA Open(VISA resource name=w1010) -> (VISA resource name=w1015:refnum<visa-resource-name>, error out=w1014:errorcluster)  [unwired: 1 in, 3 out]
                                n1191 = Unbundle By Name(w1014) -> ()  [unwired: 1 out]
                                n1192 = property class="GPIB BoardInterface"(reference=w1015, error in=w1014, "General Settings:Timeout Value"=w1008) -> (reference out=w1012:refnum<visa-resource-name>, error out=w1011:errorcluster)
                                n1193 = VISA Enable Event(8:w1011, 10:w1013, 11:w1012) -> (0:w1007:errorcluster, 3:→"VISA bus 0 resource name out hid":refnum<visa-resource-name>)  [unwired: 1 out]
                                "VISA bus 0 error out hid" <- w1007
                                n1194 = Unbundle By Name(w1007) -> ("status"=w1006:bool)
                                n1195 = local write "VISA bus 0 open error"(w1006) -> ()
                                }
                                frame #2 {
                                n1196 = Concatenate Strings("Bus 0 initializing " ("string"), "\r\n") -> (w1017:string)
                                n1197 = local write "GPIB Bus 0 traffic"(w1017) -> ()
                                }
                                frame #3 {
                                n1198 = local write "Exit SC handler StMach hid"(FALSE ("Exit tester state machine hid")) -> ()
                                n1199 = local write "H1 Ready with sites hid"(FALSE ("H1 Ready with sites hid")) -> ()
                                n1200 = local write "H2 Ready with sites hid"(FALSE ("H2 Ready with sites hid")) -> ()
                                n1201 = local write "Last locked handler hid"(enum16{"H1", "H2"}."H1" ("Last locked handler hid")) -> ()
                                n1202 = local write "H1 Lock"(FALSE ("H1 Lock")) -> ()
                                n1203 = local write "H2 Lock"(FALSE ("H1 Lock")) -> ()
                                }
                                frame #4 {
                                n1204 = local read "Tester Handler Config"() -> (w1025:T2)
                                n1205 = case shown="\"Seiko-Epson NS6040\"" w1025 {
                                frame "Multitest", Default {
                                n1206 = local write "SC handler states hid"(SC_handler_states."waiting on event" ("SC Test Interface States")) -> ()
                                }
                                frame "Seiko-Epson NS6040" {
                                n1207 = local write "SC handler states hid"(SC_handler_states."waiting on serial poll" ("SC Test Interface States")) -> ()
                                }
                                }
                                }
                                }
                              }
                              frame "waiting on serial poll" {
                                n1208 = flat-sequence {
                                frame #0 {
                                n1209 = local write "GPIB Bus 0 traffic"("Bus 0 waiting on SPOLL" ("string")) -> ()
                                }
                                frame #1 {
                                n1210 = while {
                                i -> [w1031]
                                stop <- w1033 stop-if-true
                                n1211 = local read "H1 Ready with sites hid"() -> (w1034:bool)
                                n1212 = local read "H2 Ready with sites hid"() -> (w1035:bool)
                                n1213 = Or(x=w1034, y=w1035) -> (x .or. y?=w1033:bool)
                                n1214 = Wait (ms)(milliseconds to wait=u32 5) -> ()  [unwired: 1 out]
                                "Numeric" <- w1031
                                }
                                }
                                frame #2 {
                                n1215 = property class="GPIB BoardInterface"(reference=refnum<visa-resource-name> "GPIB0::INTFC", "Device STB"=u8 65 ("Message Based Settings:Device Status Byte")) -> ()  [unwired: 1 in, 2 out]
                                }
                                frame #3 {
                                n1216 = local read "VISA bus 0 resource name out hid"() -> (w1039:refnum<visa-resource-name>)
                                n1217 = local read "VISA bus 0 error out hid"() -> (w1038:errorcluster)
                                n1218 = local read "GPIB wait timeout hid"() -> (w1047:u32)
                                n1219 = VISA Wait on Event(7:w1047, 8:w1038, 11:w1039) -> (0:w1042:errorcluster, 3:w1041:refnum<visa-resource-name>)  [unwired: 2 in, 2 out]
                                n1220 = local write "VISA bus 0 resource name out hid"(w1041) -> ()
                                n1221 = local write "VISA bus 0 error out hid"(w1042) -> ()
                                n1222 = Unbundle By Name(w1042) -> ("status"=w1044:bool)
                                n1223 = Unbundle By Name(w1042) -> ("code"=w1046:i32)
                                n1224 = Equal?(x=w1046, y=-1073807339) -> (x = y?=w1043:bool)
                                n1225 = Or(x=w1044, y=w1043) -> (x .or. y?=w1040:bool)
                                n1226 = case shown="False" w1040 {
                                frame False {
                                n1227 = flat-sequence {
                                frame #0 {
                                n1228 = property class="GPIB BoardInterface"(reference=refnum<visa-resource-name> "GPIB0::INTFC") -> ("ATN State"=w1048:i16)  [unwired: 1 in, 2 out]
                                n1229 = case shown="0" w1048 {
                                frame 0 {
                                n1230 = flat-sequence {
                                frame #0 {
                                n1231 = local read "Last locked handler hid"() -> (w1050:enum16{"H1", "H2"})
                                n1232 = case shown="\"H1\", Default" w1050 {
                                frame "H1", Default {
                                n1233 = local read "H2 Ready with sites hid"() -> (w1051:bool)
                                n1234 = case shown="False" w1051 {
                                frame False {
                                n1235 = local read "H1 Ready with sites hid"() -> (w1052:bool)
                                n1236 = case shown="True" w1052 {
                                frame False {
                                }
                                frame True {
                                n1237 = local read "H1 loop counter hid"() -> (w1056:u32)
                                n1238 = local write "H1 Lock"(TRUE ("H1 Lock")) -> ()
                                n1239 = local write "Last locked handler hid"(enum16{"H1", "H2"}."H1" ("Last locked handler hid")) -> ()
                                n1240 = Increment(x=w1056) -> (x+1=w1055:u32)
                                n1241 = local write "H1 loop counter hid"(w1055) -> ()
                                }
                                }
                                }
                                frame True {
                                n1242 = local read "H2 loop counter hid"() -> (w1059:u32)
                                n1243 = local write "H2 Lock"(TRUE ("H2 Lock")) -> ()
                                n1244 = local write "Last locked handler hid"(enum16{"H1", "H2"}."H2" ("Last locked handler hid")) -> ()
                                n1245 = Increment(x=w1059) -> (x+1=w1060:u32)
                                n1246 = local write "H2 loop counter hid"(w1060) -> ()
                                }
                                }
                                }
                                frame "H2" {
                                n1247 = local read "H1 Ready with sites hid"() -> (w1061:bool)
                                n1248 = case shown="True" w1061 {
                                frame False {
                                n1249 = local read "H2 Ready with sites hid"() -> (w1062:bool)
                                n1250 = case shown="True" w1062 {
                                frame False {
                                }
                                frame True {
                                n1251 = local read "H2 loop counter hid"() -> (w1065:u32)
                                n1252 = local write "H2 Lock"(TRUE ("H2 Lock")) -> ()
                                n1253 = local write "Last locked handler hid"(enum16{"H1", "H2"}."H2" ("Last locked handler hid")) -> ()
                                n1254 = Increment(x=w1065) -> (x+1=w1066:u32)
                                n1255 = local write "H2 loop counter hid"(w1066) -> ()
                                }
                                }
                                }
                                frame True {
                                n1256 = local read "H1 loop counter hid"() -> (w1070:u32)
                                n1257 = local write "H1 Lock"(TRUE ("H1 Lock")) -> ()
                                n1258 = local write "Last locked handler hid"(enum16{"H1", "H2"}."H1" ("Last locked handler hid")) -> ()
                                n1259 = Increment(x=w1070) -> (x+1=w1069:u32)
                                n1260 = local write "H1 loop counter hid"(w1069) -> ()
                                }
                                }
                                }
                                }
                                }
                                frame #1 {
                                n1261 = local write "SC handler states hid"(SC_handler_states."waiting on event" ("SC Test Interface States")) -> ()
                                }
                                }
                                }
                                frame 1, Default {
                                n1262 = flat-sequence {
                                frame #0 {
                                n1263 = Wait (ms)(milliseconds to wait=u32 5) -> ()  [unwired: 1 out]
                                }
                                frame #1 {
                                n1264 = local write "SC handler states hid"(SC_handler_states."waiting on serial poll" ("SC Test Interface States")) -> ()
                                }
                                }
                                }
                                }
                                }
                                }
                                }
                                frame True {
                                n1265 = flat-sequence {
                                frame #0 {
                                n1266 = local read "VISA bus 0 resource name out hid"() -> (w1074:refnum<visa-resource-name>)
                                n1267 = local read "VISA bus 0 error out hid"() -> (w1075:errorcluster)
                                n1268 = VISA Close(VISA resource name=w1074, error in (no error)=w1075) -> (error out=w1077:errorcluster)
                                n1269 = Unbundle By Name(w1077) -> ("status"=w1076:bool)
                                n1270 = local write "VISA bus 0 close error"(w1076) -> ()
                                }
                                frame #1 {
                                n1271 = local write "SC handler states hid"(SC_handler_states."closing bus" ("SC Test Interface States")) -> ()
                                }
                                }
                                }
                                }
                                }
                                }
                              }
                              frame "waiting on event" {
                                n1272 = flat-sequence {
                                frame #0 {
                                n1273 = local read "GPIB Bus 0 traffic"() -> (w1081:string)
                                n1274 = Concatenate Strings(w1081, "\r\n", "Bus 0 waiting on event" ("string")) -> (w1084:string)
                                n1275 = local write "GPIB Bus 0 traffic"(w1084) -> ()
                                }
                                frame #1 {
                                n1276 = local read "VISA bus 0 resource name out hid"() -> (w1094:refnum<visa-resource-name>)
                                n1277 = local read "VISA bus 0 error out hid"() -> (w1093:errorcluster)
                                n1278 = local read "GPIB wait timeout hid"() -> (w1092:u32)
                                n1279 = VISA Wait on Event(7:w1092, 8:w1093, 11:w1094) -> (0:w1085:errorcluster, 3:w1086:refnum<visa-resource-name>)  [unwired: 2 in, 2 out]
                                n1280 = local write "VISA bus 0 resource name out hid"(w1086) -> ()
                                n1281 = local write "VISA bus 0 error out hid"(w1085) -> ()
                                n1282 = Unbundle By Name(w1085) -> ("status"=w1089:bool)
                                n1283 = Unbundle By Name(w1085) -> ("code"=w1091:i32)
                                n1284 = Equal?(x=w1091, y=-1073807339) -> (x = y?=w1088:bool)
                                n1285 = Or(x=w1089, y=w1088) -> (x .or. y?=w1087:bool)
                                n1286 = case shown="False" w1087 {
                                tunnel: w1086 -> [_ w1097]
                                tunnel: w1085 -> [_ w1096]
                                frame False {
                                n1287 = local write "SC handler states hid"(SC_handler_states."reading" ("SC Test Interface States")) -> ()
                                }
                                frame True {
                                n1288 = flat-sequence {
                                tunnel: w1097 -> [w1101]
                                tunnel: w1096 -> [w1100]
                                frame #0 {
                                n1289 = VISA Close(VISA resource name=w1101, error in (no error)=w1100) -> (error out=w1099:errorcluster)
                                n1290 = Unbundle By Name(w1099) -> ("status"=w1098:bool)
                                n1291 = local write "VISA bus 0 close error"(w1098) -> ()
                                }
                                frame #1 {
                                n1292 = Concatenate Strings("GPIB bus 0 error or time out waiting on event,\nclosing Bus 0 and re-initializing." ("string"), "\r\n") -> (w1104:string)
                                n1293 = local write "GPIB Bus 0 traffic"(w1104) -> ()
                                }
                                frame #2 {
                                n1294 = local write "SC handler states hid"(SC_handler_states."initializing bus" ("SC Test Interface States")) -> ()
                                }
                                }
                                }
                                }
                                }
                                }
                              }
                              frame "reading" {
                                n1295 = flat-sequence {
                                tunnel: [w1110] -> w1107
                                tunnel: [w1113] -> w1106
                                tunnel: w1107 -> [w1125]
                                tunnel: w1106 -> [w1124]
                                frame #0 {
                                n1296 = local read "VISA bus 0 resource name out hid"() -> (w1120:refnum<visa-resource-name>)
                                n1297 = local read "VISA bus 0 error out hid"() -> (w1121:errorcluster)
                                n1298 = VISA Read(VISA resource name=w1120, byte count=128, error in (no error)=w1121) -> (VISA resource name out=w1119:refnum<visa-resource-name>, read buffer=w1115:string, return count=w1114:u32, error out=w1111:errorcluster)
                                n1299 = local write "VISA bus 0 resource name out hid"(w1119) -> ()
                                n1300 = local write "Message from tester hid"(w1115) -> ()
                                n1301 = Unbundle By Name(w1111) -> ("status"=w1112:bool)
                                n1302 = call <vilib>:"Trim Whitespace.vi"("string"=w1115) -> ("trimmed string"=w1110:string)  [unwired: 1 in]
                                n1303 = Greater Than 0?(x=w1114) -> (x > 0?=w1113:bool)
                                n1304 = local write "GPIB bus 0 read error"(w1112) -> ()
                                n1305 = local read "GPIB Bus 0 traffic"() -> (w1118:string)
                                n1306 = Concatenate Strings(w1118, "\r\n", "Bus 0 read: " ("string"), w1110) -> (w1116:string)
                                n1307 = local write "GPIB Bus 0 traffic"(w1116) -> ()
                                }
                                frame #1 {
                                n1308 = case shown="True" w1124 {
                                tunnel: w1125 -> [_ w1128]
                                frame False {
                                n1309 = local write "SC handler states hid"(SC_handler_states."waiting on event" ("SC Test Interface States")) -> ()
                                n1310 = Wait (ms)(milliseconds to wait=u32 1) -> ()  [unwired: 1 out]
                                }
                                frame True {
                                n1311 = flat-sequence {
                                tunnel: [w1131] -> w1129
                                tunnel: w1128 -> [w1131]
                                tunnel: [w1134] -> w1130
                                tunnel: w1129 -> [w1134]
                                tunnel: w1130 -> [w1135]
                                frame #0 {
                                n1312 = local read "Slow for  Diagnostics"() -> (w1132:bool)
                                n1313 = case shown="True" w1132 {
                                frame False {
                                }
                                frame True {
                                n1314 = local read "GPIB wait time (ms)"() -> (w1133:u32)
                                n1315 = Wait (ms)(milliseconds to wait=w1133) -> ()  [unwired: 1 out]
                                }
                                }
                                }
                                frame #1 {
                                }
                                frame #2 {
                                n1316 = Match Pattern(string=w1135, regular expression="?") -> (offset past match=w1138:i32)  [unwired: 1 in, 3 out]
                                n1317 = Greater Or Equal To 0?(x=w1138) -> (x >= 0?=w1136:bool)
                                n1318 = case shown="False" w1136 {
                                tunnel: w1135 -> [w1142 w1157]
                                frame False {
                                n1319 = Match Pattern(string=w1142, regular expression=":" ("true string")) -> (offset past match=w1139:i32)  [unwired: 1 in, 3 out]
                                n1320 = Greater Or Equal To 0?(x=w1139) -> (x >= 0?=w1140:bool)
                                n1321 = case shown="False" w1140 {
                                tunnel: w1142 -> [w1145 w1152]
                                frame False {
                                n1322 = call <vilib>:"Space Constant.vi"() -> ("String"=w1146:string)
                                n1323 = Match Pattern(string=w1145, regular expression=w1146) -> (offset past match=w1144:i32)  [unwired: 1 in, 3 out]
                                n1324 = Greater Or Equal To 0?(x=w1144) -> (x >= 0?=w1143:bool)
                                n1325 = case shown="False" w1143 {
                                tunnel: w1145 -> [w1147 w1149]
                                frame False {
                                n1326 = local write "GPIB parsed msg from tester hid"(w1147) -> ()
                                }
                                frame True {
                                n1327 = call <vilib>:"Space Constant.vi"() -> ("String"=w1150:string)
                                n1328 = Match Pattern(string=w1149, regular expression=w1150) -> (before substring=w1148:string)  [unwired: 1 in, 3 out]
                                n1329 = local write "GPIB parsed msg from tester hid"(w1148) -> ()
                                }
                                }
                                }
                                frame True {
                                n1330 = Match Pattern(string=w1152, regular expression=":") -> (before substring=w1151:string)  [unwired: 1 in, 3 out]
                                n1331 = local write "GPIB parsed msg from tester hid"(w1151) -> ()
                                }
                                }
                                }
                                frame True {
                                w1155 = "?" ("regular expression")
                                n1332 = Match Pattern(string=w1157, regular expression=w1155) -> (before substring=w1156:string)  [unwired: 1 in, 3 out]
                                n1333 = Concatenate Strings(w1156, w1155) -> (w1154:string)
                                n1334 = local write "GPIB parsed msg from tester hid"(w1154) -> ()
                                }
                                }
                                }
                                frame #3 {
                                n1335 = local read "GPIB parsed msg from tester hid"() -> (w1158:string)
                                n1336 = case shown="\"Fullsites?\"" w1158 {
                                frame "*IDN?" {
                                n1337 = local write "SC handler states hid"(SC_handler_states."responding to *IDN?" ("SC Test Interface States")) -> ()
                                }
                                frame "SITES?" {
                                n1338 = local read "Tester online"() -> (w1162:bool)
                                n1339 = local read "POWER"() -> (w1160:bool)
                                n1340 = Compound Arithmetic op=AND(w1162, w1160) -> (w1161:bool)
                                n1341 = case shown="True" w1161 {
                                frame False {
                                n1342 = local write "SC handler states hid"(SC_handler_states."closing bus" ("SC virtual handler states")) -> ()
                                }
                                frame True {
                                n1343 = flat-sequence {
                                frame #0 {
                                # "this could be a problem or uneccessary"
                                n1344 = while {
                                stop <- w1165 stop-if-true
                                n1345 = local read "H1 Waiting"() -> (w1167:bool)
                                n1346 = local read "H2 Waiting"() -> (w1166:bool)
                                n1347 = Or(x=w1167, y=w1166) -> (x .or. y?=w1165:bool)
                                n1348 = Wait (ms)(milliseconds to wait=u32 5) -> ()  [unwired: 1 out]
                                }
                                }
                                frame #1 {
                                n1349 = local write "SC handler states hid"(SC_handler_states."responding to SITES?" ("SC Test Interface States")) -> ()
                                }
                                }
                                }
                                }
                                }
                                frame "Fullsites?" {
                                n1350 = local write "SC handler states hid"(SC_handler_states."responding to Fullsites?" ("SC Test Interface States")) -> ()
                                }
                                frame "HIDN?" {
                                n1351 = local write "SC handler states hid"(SC_handler_states."responding to HIDN?" ("SC Test Interface States")) -> ()
                                }
                                frame "HAND?" {
                                n1352 = local write "SC handler states hid"(SC_handler_states."respond to HAND?" ("SC Test Interface States")) -> ()
                                }
                                frame "A BIN" {
                                n1353 = flat-sequence {
                                frame #0 {
                                n1354 = local read "Message from tester hid"() -> (w1172:string)
                                n1355 = local write "Binning string from tester hid"(w1172) -> ()
                                }
                                frame #1 {
                                n1356 = local write "SC handler states hid"(SC_handler_states."responding to A BIN" ("SC Test Interface States")) -> ()
                                }
                                }
                                }
                                frame "BINON" {
                                n1357 = flat-sequence {
                                frame #0 {
                                # "when this loop unlocks the handlers,\nthe handler interface loops are free to continue\nto send the binning information to their\nrespective handlers."
                                n1358 = local write "H1 Lock"(FALSE ("H1 Lock")) -> ()
                                n1359 = local write "H2 Lock"(FALSE ("H1 Lock")) -> ()
                                n1360 = local write "Binning string from tester hid"("") -> ()
                                n1361 = local read "Message from tester hid"() -> (w1178:string)
                                n1362 = local write "Echo state of tester hid"(Echo_tester_states."NO ECHO" ("Echo state of tester hid")) -> ()
                                n1363 = local write "Binning string from tester hid"(w1178) -> ()
                                }
                                frame #1 {
                                n1364 = local write "SC handler states hid"(SC_handler_states."responding to BINON" ("SC Test Interface States")) -> ()
                                }
                                }
                                }
                                frame "ECHOOK" {
                                # "5"
                                n1365 = local write "Echo state of tester hid"(Echo_tester_states."ECHOOK" ("Echo state of tester hid")) -> ()
                                n1366 = local write "SC handler states hid"(SC_handler_states."ECHOOK" ("SC Test Interface States")) -> ()
                                n1367 = local write "H1 Lock"(FALSE ("H1 Lock")) -> ()
                                n1368 = local write "H2 Lock"(FALSE ("H2 Lock")) -> ()
                                }
                                frame "ECHONG" {
                                n1369 = local write "Echo state of tester hid"(Echo_tester_states."ECHONG" ("Echo state of tester hid")) -> ()
                                n1370 = local write "SC handler states hid"(SC_handler_states."ECHONG" ("SC Test Interface States")) -> ()
                                }
                                frame Default {
                                n1371 = local write "SC handler states hid"(SC_handler_states."responding to unknown command" ("SC Test Interface States")) -> ()
                                }
                                }
                                }
                                }
                                }
                                }
                                }
                                }
                              }
                              frame "responding to *IDN?" {
                                n1372 = flat-sequence {
                                frame #0 {
                                n1373 = while {
                                stop <- w1192 stop-if-true
                                w1189 = "Sentinel Controller Handler Interface"
                                n1374 = local read "VISA bus 0 resource name out hid"() -> (w1201:refnum<visa-resource-name>)
                                n1375 = local read "VISA bus 0 error out hid"() -> (w1200:errorcluster)
                                n1376 = local read "GPIB Bus 0 traffic"() -> (w1197:string)
                                n1377 = VISA Write(VISA resource name=w1201, write buffer=w1189, error in (no error)=w1200) -> (VISA resource name out=w1199:refnum<visa-resource-name>, return count=w1193:u32, error out=w1198:errorcluster)
                                n1378 = call <vilib>:"Trim Whitespace.vi"("string"=w1189) -> ("trimmed string"=w1190:string)  [unwired: 1 in]
                                n1379 = local write "VISA bus 0 resource name out hid"(w1199) -> ()
                                n1380 = local write "VISA bus 0 error out hid"(w1198) -> ()
                                n1381 = Unbundle By Name(w1198) -> ("status"=w1191:bool)
                                n1382 = Concatenate Strings(w1197, "\r\n", "Bus 0 write: " ("string"), w1190) -> (w1195:string)
                                n1383 = Greater Than 0?(x=w1193) -> (x > 0?=w1192:bool)
                                n1384 = local write "GPIB bus 0 write error"(w1191) -> ()
                                n1385 = local write "GPIB Bus 0 traffic"(w1195) -> ()
                                }
                                }
                                frame #1 {
                                n1386 = local write "SC handler states hid"(SC_handler_states."waiting on event" ("SC Test Interface States")) -> ()
                                }
                                }
                              }
                              frame "respond to HAND?" {
                                n1387 = local read "H1 Lock"() -> (w1205:bool)
                                n1388 = case shown="True" w1205 {
                                frame False {
                                n1389 = local read "H2 Lock"() -> (w1206:bool)
                                n1390 = case shown="True" w1206 {
                                frame False {
                                n1391 = flat-sequence {
                                frame #0 {
                                n1392 = One Button Dialog(message="Fatal error 200:\nThe SC responded to a handler being ready with devices\nto test, but when the SC check for a lock when responding\nto *HAND?, no handler had a lock. \nPlease report this bug to Celerint at www.celerint.com  ") -> ()  [unwired: 1 in, 1 out]
                                }
                                frame #1 {
                                n1393 = local write "SC handler states hid"(SC_handler_states."closing bus" ("SC Test Interface States")) -> ()
                                }
                                }
                                }
                                frame True {
                                n1394 = flat-sequence {
                                frame #0 {
                                n1395 = while {
                                stop <- w1212 stop-if-true
                                w1210 = "H2" ("string")
                                n1396 = local read "VISA bus 0 resource name out hid"() -> (w1218:refnum<visa-resource-name>)
                                n1397 = local read "GPIB Bus 0 traffic"() -> (w1216:string)
                                n1398 = local read "VISA bus 0 error out hid"() -> (w1217:errorcluster)
                                n1399 = call <vilib>:"Trim Whitespace.vi"("string"=w1210) -> ("trimmed string"=w1209:string)  [unwired: 1 in]
                                n1400 = VISA Write(VISA resource name=w1218, write buffer=w1210, error in (no error)=w1217) -> (VISA resource name out=w1219:refnum<visa-resource-name>, return count=w1211:u32, error out=w1220:errorcluster)
                                n1401 = Concatenate Strings(w1216, "\r\n", "H2: Bus 0 write: " ("string"), w1209) -> (w1214:string)
                                n1402 = local write "VISA bus 0 error out hid"(w1220) -> ()
                                n1403 = Unbundle By Name(w1220) -> ("status"=w1221:bool)
                                n1404 = local write "GPIB Bus 0 traffic"(w1214) -> ()
                                n1405 = Greater Than 0?(x=w1211) -> (x > 0?=w1212:bool)
                                n1406 = local write "VISA bus 0 resource name out hid"(w1219) -> ()
                                n1407 = local write "GPIB bus 0 write error"(w1221) -> ()
                                }
                                }
                                frame #1 {
                                n1408 = local write "SC handler states hid"(SC_handler_states."waiting on event" ("SC Test Interface States")) -> ()
                                }
                                }
                                }
                                }
                                }
                                frame True {
                                n1409 = flat-sequence {
                                frame #0 {
                                n1410 = while {
                                stop <- w1226 stop-if-true
                                w1224 = "H1" ("string")
                                n1411 = local read "VISA bus 0 resource name out hid"() -> (w1232:refnum<visa-resource-name>)
                                n1412 = local read "GPIB Bus 0 traffic"() -> (w1230:string)
                                n1413 = local read "VISA bus 0 error out hid"() -> (w1231:errorcluster)
                                n1414 = call <vilib>:"Trim Whitespace.vi"("string"=w1224) -> ("trimmed string"=w1223:string)  [unwired: 1 in]
                                n1415 = Concatenate Strings(w1230, "\r\n", "H1: Bus 0 write: " ("string"), w1223) -> (w1228:string)
                                n1416 = VISA Write(VISA resource name=w1232, write buffer=w1224, error in (no error)=w1231) -> (VISA resource name out=w1233:refnum<visa-resource-name>, return count=w1225:u32, error out=w1234:errorcluster)
                                n1417 = local write "VISA bus 0 resource name out hid"(w1233) -> ()
                                n1418 = local write "VISA bus 0 error out hid"(w1234) -> ()
                                n1419 = Unbundle By Name(w1234) -> ("status"=w1235:bool)
                                n1420 = local write "GPIB Bus 0 traffic"(w1228) -> ()
                                n1421 = Greater Than 0?(x=w1225) -> (x > 0?=w1226:bool)
                                n1422 = local write "GPIB bus 0 write error"(w1235) -> ()
                                }
                                }
                                frame #1 {
                                n1423 = local write "SC handler states hid"(SC_handler_states."waiting on event" ("SC Test Interface States")) -> ()
                                }
                                }
                                }
                                }
                              }
                              frame "responding to HIDN?" {
                                n1424 = local read "H1 Lock"() -> (w1239:bool)
                                n1425 = case shown="True" w1239 {
                                frame False {
                                n1426 = local read "H2 Lock"() -> (w1240:bool)
                                n1427 = case shown="True" w1240 {
                                frame False {
                                n1428 = flat-sequence {
                                frame #0 {
                                n1429 = One Button Dialog(message="Fatal error 201:\nThe SC responded to a handler being ready with devices\nto test, but when the SC check for a lock when responding\nto *HIDN?, no handler had a lock. \nPlease report this bug to Celerint at www.celerint.com  ") -> ()  [unwired: 1 in, 1 out]
                                }
                                frame #1 {
                                n1430 = local write "SC handler states hid"(SC_handler_states."testing" ("SC Test Interface States")) -> ()
                                }
                                }
                                }
                                frame True {
                                n1431 = flat-sequence {
                                frame #0 {
                                n1432 = while {
                                stop <- w1246 stop-if-true
                                n1433 = local read "VISA bus 0 resource name out hid"() -> (w1252:refnum<visa-resource-name>)
                                n1434 = local read "H2 response to *HAND? hid"() -> (w1244:string)
                                n1435 = local read "VISA bus 0 error out hid"() -> (w1251:errorcluster)
                                n1436 = local read "GPIB Bus 0 traffic"() -> (w1250:string)
                                n1437 = VISA Write(VISA resource name=w1252, write buffer=w1244, error in (no error)=w1251) -> (VISA resource name out=w1253:refnum<visa-resource-name>, return count=w1245:u32, error out=w1254:errorcluster)
                                n1438 = call <vilib>:"Trim Whitespace.vi"("string"=w1244) -> ("trimmed string"=w1243:string)  [unwired: 1 in]
                                n1439 = local write "VISA bus 0 error out hid"(w1254) -> ()
                                n1440 = Unbundle By Name(w1254) -> ("status"=w1255:bool)
                                n1441 = Concatenate Strings(w1250, "\r\n", "H2: Bus 0 write: " ("string"), w1243) -> (w1248:string)
                                n1442 = Greater Than 0?(x=w1245) -> (x > 0?=w1246:bool)
                                n1443 = local write "VISA bus 0 resource name out hid"(w1253) -> ()
                                n1444 = local write "GPIB Bus 0 traffic"(w1248) -> ()
                                n1445 = local write "GPIB bus 0 write error"(w1255) -> ()
                                }
                                }
                                frame #1 {
                                n1446 = local write "SC handler states hid"(SC_handler_states."waiting on event" ("SC Test Interface States")) -> ()
                                }
                                }
                                }
                                }
                                }
                                frame True {
                                n1447 = flat-sequence {
                                frame #0 {
                                n1448 = while {
                                stop <- w1260 stop-if-true
                                n1449 = local read "VISA bus 0 resource name out hid"() -> (w1266:refnum<visa-resource-name>)
                                n1450 = local read "H1 response to *HAND? hid"() -> (w1258:string)
                                n1451 = local read "VISA bus 0 error out hid"() -> (w1265:errorcluster)
                                n1452 = local read "GPIB Bus 0 traffic"() -> (w1264:string)
                                n1453 = call <vilib>:"Trim Whitespace.vi"("string"=w1258) -> ("trimmed string"=w1257:string)  [unwired: 1 in]
                                n1454 = VISA Write(VISA resource name=w1266, write buffer=w1258, error in (no error)=w1265) -> (VISA resource name out=w1267:refnum<visa-resource-name>, return count=w1259:u32, error out=w1268:errorcluster)
                                n1455 = local write "VISA bus 0 resource name out hid"(w1267) -> ()
                                n1456 = local write "VISA bus 0 error out hid"(w1268) -> ()
                                n1457 = Unbundle By Name(w1268) -> ("status"=w1269:bool)
                                n1458 = Concatenate Strings(w1264, "\r\n", "H1: Bus 0 write: " ("string"), w1257) -> (w1262:string)
                                n1459 = Greater Than 0?(x=w1259) -> (x > 0?=w1260:bool)
                                n1460 = local write "GPIB Bus 0 traffic"(w1262) -> ()
                                n1461 = local write "GPIB bus 0 write error"(w1269) -> ()
                                }
                                }
                                frame #1 {
                                n1462 = local write "SC handler states hid"(SC_handler_states."waiting on event" ("SC Test Interface States")) -> ()
                                }
                                }
                                }
                                }
                              }
                              frame "responding to Fullsites?" {
                                n1463 = local read "Last locked handler hid"() -> (w1271:enum16{"H1", "H2"})
                                n1464 = case shown="\"H2\"" w1271 {
                                frame "H1", Default {
                                n1465 = flat-sequence {
                                frame #0 {
                                n1466 = while {
                                i -> [w1277]
                                stop <- w1279 stop-if-true
                                n1467 = local read "VISA bus 0 resource name out hid"() -> (w1276:refnum<visa-resource-name>)
                                n1468 = local read "VISA bus 0 error out hid"() -> (w1275:errorcluster)
                                n1469 = local read "H1 FULLSITES? response hid"() -> (w1280:string)
                                n1470 = local read "GPIB Bus 0 traffic"() -> (w1282:string)
                                n1471 = call <vilib>:"Trim Whitespace.vi"("string"=w1280) -> ("trimmed string"=w1281:string)  [unwired: 1 in]
                                n1472 = VISA Write(VISA resource name=w1276, write buffer=w1280, error in (no error)=w1275) -> (return count=w1278:u32, error out=w1286:errorcluster)  [unwired: 1 out]
                                n1473 = Unbundle By Name(w1286) -> ("status"=w1274:bool)
                                n1474 = local write "VISA bus 0 error out hid"(w1286) -> ()
                                n1475 = Concatenate Strings(w1282, "\r\n", "Bus 0 write: " ("string"), w1281) -> (w1284:string)
                                n1476 = local write "GPIB bus 0 write error"(w1274) -> ()
                                n1477 = local write "GPIB Bus 0 traffic"(w1284) -> ()
                                n1478 = Greater Than 0?(x=w1278) -> (x > 0?=w1279:bool)
                                "Numeric 3" <- w1277
                                }
                                }
                                frame #1 {
                                n1479 = local write "SC handler states hid"(SC_handler_states."testing" ("SC Test Interface States")) -> ()
                                }
                                }
                                }
                                frame "H2" {
                                n1480 = flat-sequence {
                                frame #0 {
                                n1481 = while {
                                stop <- w1291 stop-if-true
                                n1482 = local read "VISA bus 0 resource name out hid"() -> (w1288:refnum<visa-resource-name>)
                                n1483 = local read "H2 FULLSITES? response hid"() -> (w1292:string)
                                n1484 = local read "VISA bus 0 error out hid"() -> (w1289:errorcluster)
                                n1485 = local read "GPIB Bus 0 traffic"() -> (w1294:string)
                                n1486 = VISA Write(VISA resource name=w1288, write buffer=w1292, error in (no error)=w1289) -> (return count=w1290:u32, error out=w1298:errorcluster)  [unwired: 1 out]
                                n1487 = call <vilib>:"Trim Whitespace.vi"("string"=w1292) -> ("trimmed string"=w1293:string)  [unwired: 1 in]
                                n1488 = local write "VISA bus 0 error out hid"(w1298) -> ()
                                n1489 = Unbundle By Name(w1298) -> ("status"=w1299:bool)
                                n1490 = local write "GPIB bus 0 write error"(w1299) -> ()
                                n1491 = Concatenate Strings(w1294, "\r\n", "Bus 0 write: " ("string"), w1293) -> (w1296:string)
                                n1492 = local write "GPIB Bus 0 traffic"(w1296) -> ()
                                n1493 = Greater Than 0?(x=w1290) -> (x > 0?=w1291:bool)
                                }
                                }
                                frame #1 {
                                n1494 = local write "SC handler states hid"(SC_handler_states."testing" ("SC Test Interface States")) -> ()
                                }
                                }
                                }
                                }
                              }
                              frame "testing" {
                                n1495 = flat-sequence {
                                tunnel: w1311 -> [w1315]
                                tunnel: w1312 -> [w1316]
                                tunnel: [w1314] -> w1308
                                tunnel: [w1313] -> w1307
                                tunnel: w1308 -> [w1332]
                                tunnel: [w1332] -> w1306
                                tunnel: w1307 -> [w1331]
                                tunnel: [w1331] -> w1305
                                tunnel: w1306 -> [w1334]
                                tunnel: w1305 -> [w1333]
                                tunnel: [w1334] -> w1304
                                tunnel: [w1333] -> w1303
                                tunnel: w1304 -> [w1343]
                                tunnel: w1303 -> [w1342]
                                tunnel: [w1343] -> w1302
                                tunnel: [w1342] -> w1301
                                tunnel: [w1345] -> w1310
                                tunnel: [w1346] -> w1309
                                tunnel: w1302 -> [w1346]
                                tunnel: w1301 -> [w1345]
                                frame #0 {
                                n1496 = local read "SC measured test time hid"() -> (w1317:dbl)
                                n1497 = local read "SC measured wait time hid"() -> (w1318:dbl)
                                n1498 = local read "Tester loop counter hid"() -> (w1320:u32)
                                n1499 = Add(x=w1317, y=w1318) -> (x+y=w1324:dbl)
                                n1500 = local read "Utilization averaging"() -> (w1319:i32)
                                n1501 = Divide(x=w1317, y=w1324) -> (x/y=w1325:dbl)
                                n1502 = Multiply(x=100.0, y=w1325) -> (x*y=w1321:dbl)
                                n1503 = call "moving_avg_core.vi"("Array in"=w1315, "avg"=w1319, "accumulator in"=w1316, "i"=w1320, "data in"=w1321) -> ("Array out"=w1314:dbl[], "accumulator out"=w1313:dbl, "rolling avg out"=w1322:dbl)  [unwired: 4 in]
                                n1504 = Bundle(w1321, "rolling avg out"=w1322) -> (w1323:cluster{dbl, "rolling avg out":dbl})  [unwired: 1 in]
                                n1505 = local write "Sys utilization"(w1322) -> ()
                                n1506 = local write "SysUtilMon"(w1323) -> ()
                                }
                                frame #1 {
                                # "empty binning string wiill hold handlers at BINON until valid"
                                n1507 = local read "H1 loop counter hid"() -> (w1329:u32)
                                n1508 = Increment(x=w1329) -> (x+1=w1330:u32)
                                n1509 = property class="GPIB BoardInterface"(reference=refnum<visa-resource-name> "GPIB0::INTFC", "Device STB"=u8 0 ("Message Based Settings:Device Status Byte")) -> ()  [unwired: 1 in, 2 out]
                                n1510 = local write "H1 loop counter hid"(w1330) -> ()
                                }
                                frame #2 {
                                n1511 = Tick Count (ms)() -> (millisecond timer value=w1336:u32)
                                n1512 = Tick Count (ms)() -> (millisecond timer value=w1335:u32)
                                n1513 = local write "tester wt end hid"(w1336) -> ()
                                n1514 = local write "tester tt start hid"(w1335) -> ()
                                }
                                frame #3 {
                                n1515 = local read "tester wt start hid"() -> (w1340:u32)
                                n1516 = local read "tester wt end hid"() -> (w1341:u32)
                                n1517 = Subtract(x=w1341, y=w1340) -> (x-y=w1339:u32)
                                n1518 = Divide(x=w1339, y=u32 1000) -> (x/y=w1337:dbl)
                                n1519 = local write "SC measured wait time hid"(w1337) -> ()
                                }
                                frame #4 {
                                n1520 = local write "SC handler states hid"(SC_handler_states."waiting on event" ("SC Test Interface States")) -> ()
                                }
                                }
                              }
                              frame "responding to SITES?" {
                                n1521 = flat-sequence {
                                frame #0 {
                                # "This is the engine that decides if H1 is checked first or H2"
                                n1522 = local read "Last locked handler hid"() -> (w1349:enum16{"H1", "H2"})
                                n1523 = case shown="\"H2\"" w1349 {
                                frame "H1", Default {
                                n1524 = local read "H2 Waiting"() -> (w1350:bool)
                                n1525 = case shown="True" w1350 {
                                frame False {
                                n1526 = local read "H1 Waiting"() -> (w1351:bool)
                                n1527 = case shown="True" w1351 {
                                frame False {
                                # "end up here only if neither handler is waiting and ready"
                                }
                                frame True {
                                n1528 = flat-sequence {
                                frame #0 {
                                n1529 = local write "H2 Lock"(FALSE ("H1 Lock")) -> ()
                                n1530 = local write "H1 Lock"(TRUE ("H1 Lock")) -> ()
                                n1531 = local write "Last locked handler hid"(enum16{"H1", "H2"}."H1" ("Last locked handler")) -> ()
                                }
                                frame #1 {
                                n1532 = while {
                                stop <- w1357 stop-if-true
                                n1533 = local read "VISA bus 0 resource name out hid"() -> (w1365:refnum<visa-resource-name>)
                                n1534 = local read "VISA bus 0 error out hid"() -> (w1366:errorcluster)
                                n1535 = local read "H1 SITES? response hid"() -> (w1355:string)
                                n1536 = VISA Write(VISA resource name=w1365, write buffer=w1355, error in (no error)=w1366) -> (VISA resource name out=w1364:refnum<visa-resource-name>, return count=w1358:u32, error out=w1363:errorcluster)
                                n1537 = local write "VISA bus 0 resource name out hid"(w1364) -> ()
                                n1538 = Unbundle By Name(w1363) -> ("status"=w1367:bool)
                                n1539 = local write "VISA bus 0 error out hid"(w1363) -> ()
                                n1540 = call <vilib>:"Trim Whitespace.vi"("string"=w1355) -> ("trimmed string"=w1356:string)  [unwired: 1 in]
                                n1541 = Greater Than 0?(x=w1358) -> (x > 0?=w1357:bool)
                                n1542 = Concatenate Strings("H1: Tester test cycle start" ("string"), "\r\n", "Bus 0 write: " ("string"), w1356) -> (w1361:string)
                                n1543 = local write "GPIB bus 0 write error"(w1367) -> ()
                                n1544 = local write "GPIB Bus 0 traffic"(w1361) -> ()
                                }
                                }
                                }
                                }
                                }
                                }
                                frame True {
                                n1545 = flat-sequence {
                                frame #0 {
                                n1546 = local write "H1 Lock"(FALSE ("H1 Lock")) -> ()
                                n1547 = local write "H2 Lock"(TRUE ("H1 Lock")) -> ()
                                n1548 = local write "Last locked handler hid"(enum16{"H1", "H2"}."H2" ("Last locked handler")) -> ()
                                }
                                frame #1 {
                                n1549 = while {
                                stop <- w1374 stop-if-true
                                n1550 = local read "VISA bus 0 resource name out hid"() -> (w1381:refnum<visa-resource-name>)
                                n1551 = local read "VISA bus 0 error out hid"() -> (w1382:errorcluster)
                                n1552 = local read "H2 SITES? response hid"() -> (w1371:string)
                                n1553 = VISA Write(VISA resource name=w1381, write buffer=w1371, error in (no error)=w1382) -> (VISA resource name out=w1380:refnum<visa-resource-name>, return count=w1373:u32, error out=w1379:errorcluster)
                                n1554 = local write "VISA bus 0 resource name out hid"(w1380) -> ()
                                n1555 = Unbundle By Name(w1379) -> ("status"=w1383:bool)
                                n1556 = local write "VISA bus 0 error out hid"(w1379) -> ()
                                n1557 = Greater Than 0?(x=w1373) -> (x > 0?=w1374:bool)
                                n1558 = call <vilib>:"Trim Whitespace.vi"("string"=w1371) -> ("trimmed string"=w1372:string)  [unwired: 1 in]
                                n1559 = local write "GPIB bus 0 write error"(w1383) -> ()
                                n1560 = Concatenate Strings("H2: Tester test cycle start" ("string"), "\r\n", "Bus 0 write: " ("string"), w1372) -> (w1377:string)
                                n1561 = local write "GPIB Bus 0 traffic"(w1377) -> ()
                                }
                                }
                                frame #2 {
                                n1562 = local read "H2 loop counter hid"() -> (w1384:u32)
                                n1563 = Increment(x=w1384) -> (x+1=w1385:u32)
                                n1564 = local write "H2 loop counter hid"(w1385) -> ()
                                }
                                }
                                }
                                }
                                }
                                frame "H2" {
                                n1565 = local read "H1 Waiting"() -> (w1386:bool)
                                n1566 = case shown="True" w1386 {
                                frame False {
                                n1567 = local read "H2 Waiting"() -> (w1387:bool)
                                n1568 = case shown="True" w1387 {
                                frame False {
                                # "end up here only if neither handler is waiting and ready"
                                }
                                frame True {
                                n1569 = flat-sequence {
                                frame #0 {
                                n1570 = local write "H2 Lock"(TRUE ("H1 Lock")) -> ()
                                n1571 = local write "H1 Lock"(FALSE ("H1 Lock")) -> ()
                                n1572 = local write "Last locked handler hid"(enum16{"H1", "H2"}."H2" ("Last locked handler")) -> ()
                                }
                                frame #1 {
                                n1573 = while {
                                stop <- w1394 stop-if-true
                                n1574 = local read "VISA bus 0 resource name out hid"() -> (w1401:refnum<visa-resource-name>)
                                n1575 = local read "VISA bus 0 error out hid"() -> (w1402:errorcluster)
                                n1576 = local read "H2 SITES? response hid"() -> (w1391:string)
                                n1577 = VISA Write(VISA resource name=w1401, write buffer=w1391, error in (no error)=w1402) -> (VISA resource name out=w1400:refnum<visa-resource-name>, return count=w1393:u32, error out=w1399:errorcluster)
                                n1578 = local write "VISA bus 0 resource name out hid"(w1400) -> ()
                                n1579 = Unbundle By Name(w1399) -> ("status"=w1403:bool)
                                n1580 = local write "VISA bus 0 error out hid"(w1399) -> ()
                                n1581 = Greater Than 0?(x=w1393) -> (x > 0?=w1394:bool)
                                n1582 = call <vilib>:"Trim Whitespace.vi"("string"=w1391) -> ("trimmed string"=w1392:string)  [unwired: 1 in]
                                n1583 = Concatenate Strings("H2: Tester test cycle start" ("string"), "\r\n", "Bus 0 write: " ("string"), w1392) -> (w1397:string)
                                n1584 = local write "GPIB bus 0 write error"(w1403) -> ()
                                n1585 = local write "GPIB Bus 0 traffic"(w1397) -> ()
                                }
                                }
                                frame #2 {
                                n1586 = local read "H2 loop counter hid"() -> (w1404:u32)
                                n1587 = Increment(x=w1404) -> (x+1=w1405:u32)
                                n1588 = local write "H2 loop counter hid"(w1405) -> ()
                                }
                                }
                                }
                                }
                                }
                                frame True {
                                n1589 = flat-sequence {
                                frame #0 {
                                n1590 = local write "Last locked handler hid"(enum16{"H1", "H2"}."H1" ("Last locked handler")) -> ()
                                }
                                frame #1 {
                                n1591 = while {
                                stop <- w1409 stop-if-true
                                n1592 = local read "VISA bus 0 resource name out hid"() -> (w1417:refnum<visa-resource-name>)
                                n1593 = local read "VISA bus 0 error out hid"() -> (w1418:errorcluster)
                                n1594 = local read "H1 SITES? response hid"() -> (w1407:string)
                                n1595 = VISA Write(VISA resource name=w1417, write buffer=w1407, error in (no error)=w1418) -> (VISA resource name out=w1416:refnum<visa-resource-name>, return count=w1410:u32, error out=w1415:errorcluster)
                                n1596 = local write "VISA bus 0 resource name out hid"(w1416) -> ()
                                n1597 = Unbundle By Name(w1415) -> ("status"=w1419:bool)
                                n1598 = local write "VISA bus 0 error out hid"(w1415) -> ()
                                n1599 = Greater Than 0?(x=w1410) -> (x > 0?=w1409:bool)
                                n1600 = call <vilib>:"Trim Whitespace.vi"("string"=w1407) -> ("trimmed string"=w1408:string)  [unwired: 1 in]
                                n1601 = local write "GPIB bus 0 write error"(w1419) -> ()
                                n1602 = Concatenate Strings("H1: Tester test cycle start" ("string"), "\r\n", "Bus 0 write: " ("string"), w1408) -> (w1413:string)
                                n1603 = local write "GPIB Bus 0 traffic"(w1413) -> ()
                                }
                                }
                                frame #2 {
                                n1604 = local read "H1 loop counter hid"() -> (w1421:u32)
                                n1605 = Increment(x=w1421) -> (x+1=w1420:u32)
                                n1606 = local write "H1 loop counter hid"(w1420) -> ()
                                }
                                }
                                }
                                }
                                }
                                }
                                }
                                frame #1 {
                                n1607 = local write "SC handler states hid"(SC_handler_states."testing" ("SC Test Interface States")) -> ()
                                }
                                }
                              }
                              frame "responding to A BIN" {
                                n1608 = flat-sequence {
                                frame #0 {
                                n1609 = local read "H1 Lock"() -> (w1425:bool)
                                n1610 = case shown="True" w1425 {
                                frame False {
                                n1611 = local read "H2 Lock"() -> (w1426:bool)
                                n1612 = case shown="True" w1426 {
                                frame False {
                                }
                                frame True {
                                n1613 = local read "GPIB Bus 0 traffic"() -> (w1430:string)
                                n1614 = Concatenate Strings(w1430, "\r\n", "Bus 0: binning" ("string")) -> (w1428:string)
                                n1615 = local write "GPIB Bus 0 traffic"(w1428) -> ()
                                }
                                }
                                }
                                frame True {
                                n1616 = local read "GPIB Bus 0 traffic"() -> (w1434:string)
                                n1617 = Concatenate Strings(w1434, "\r\n", "Bus 0: binning" ("string")) -> (w1432:string)
                                n1618 = local write "GPIB Bus 0 traffic"(w1432) -> ()
                                }
                                }
                                }
                                frame #1 {
                                n1619 = Tick Count (ms)() -> (millisecond timer value=w1436:u32)
                                n1620 = Tick Count (ms)() -> (millisecond timer value=w1435:u32)
                                n1621 = local write "tester tt end hid"(w1436) -> ()
                                n1622 = local write "tester wt start hid"(w1435) -> ()
                                }
                                frame #2 {
                                n1623 = local read "tester tt start hid"() -> (w1440:u32)
                                n1624 = local read "tester tt end hid"() -> (w1441:u32)
                                n1625 = Subtract(x=w1441, y=w1440) -> (x-y=w1439:u32)
                                n1626 = Divide(x=w1439, y=u32 1000) -> (x/y=w1437:dbl)
                                n1627 = local write "SC measured test time hid"(w1437) -> ()
                                }
                                frame #3 {
                                n1628 = local read "H1 Lock"() -> (w1442:bool)
                                n1629 = case shown="False" w1442 {
                                frame False {
                                n1630 = local read "H2 Lock"() -> (w1443:bool)
                                n1631 = case shown="False" w1443 {
                                frame False {
                                n1632 = One Button Dialog(message="Fatal error 202:\nThe SC responded to a handler being ready with devices\nto test, but when the SC received binning data, no handler had a lock. \nPlease report this bug to Celerint at www.celerint.com  ") -> ()  [unwired: 1 in, 1 out]
                                }
                                frame True {
                                n1633 = local read "H2 online"() -> (w1464:bool)
                                n1634 = local read "Tandem\nfloorspace area"() -> (w1447:i32)
                                n1635 = local read "Std cell \nfloorspace area"() -> (w1475:i32)
                                n1636 = case shown="True" w1464 {
                                tunnel: [0 w1479] -> w1465
                                frame False {
                                }
                                frame True {
                                n1637 = local read "H2 UPH"() -> (w1480:cluster{u32, u32})
                                n1638 = Unbundle(w1480) -> (w1479:u32)  [unwired: 1 out]
                                }
                                }
                                n1639 = local read "System UPH"() -> (w1446:u32)
                                n1640 = local read "UPH"() -> (w1476:dbl)
                                n1641 = Divide(x=w1446, y=w1447) -> (x/y=w1445:dbl)
                                n1642 = local write "Tandem UPH\nper unit area"(w1445) -> ()
                                n1643 = Divide(x=w1476, y=w1475) -> (x/y=w1477:dbl)
                                n1644 = local read "Std hourly\ncost ($/hr)"() -> (w1472:dbl)
                                n1645 = local read "H1 UPH"() -> (w1474:cluster{u32, u32})
                                n1646 = local write "H1 UPH per unit area"(w1477) -> ()
                                n1647 = local read "Utilization (%)"() -> (w1457:u32)
                                n1648 = local read "Tandem hourly\ncost ($/hr)"() -> (w1473:dbl)
                                n1649 = local read "# of devices to test"() -> (w1463:u32)
                                n1650 = Unbundle(w1474) -> (w1466:u32)  [unwired: 1 out]
                                n1651 = local read "Hours per month"() -> (w1458:i32)
                                n1652 = local write "Calc H2 UPH"(w1465) -> ()
                                n1653 = local write "Calc H1 UPH"(w1466) -> ()
                                n1654 = local read "UPH"() -> (w1471:dbl)
                                n1655 = Add(x=w1466, y=w1465) -> (x+y=w1453:u32)
                                n1656 = Divide(x=w1457, y=u32 100) -> (x/y=w1456:dbl)
                                n1657 = Divide(x=w1463, y=w1453) -> (x/y=w1462:dbl)
                                n1658 = Multiply(x=w1458, y=w1456) -> (x*y=w1454:dbl)
                                n1659 = Divide(x=w1472, y=w1471) -> (x/y=w1470:dbl)
                                n1660 = Divide(x=w1473, y=w1453) -> (x/y=w1468:dbl)
                                n1661 = local write "System UPH"(w1453) -> ()
                                n1662 = local write "Calc\nsystem UPH"(w1453) -> ()
                                n1663 = local read "# of devices to test"() -> (w1451:u32)
                                n1664 = Divide(x=w1462, y=w1454) -> (x/y=w1461:dbl)
                                n1665 = Multiply(x=w1470, y=100.0) -> (x*y=w1449:dbl)
                                n1666 = Multiply(x=w1468, y=100.0) -> (x*y=w1448:dbl)
                                n1667 = local write "Std unit cost\n(cents/device)"(w1449) -> ()
                                n1668 = local write "Tandem unit cost\n(cents/device)"(w1448) -> ()
                                n1669 = Subtract(x=w1449, y=w1448) -> (x-y=w1452:dbl)
                                n1670 = Multiply(x=w1461, y=30) -> (x*y=w1459:dbl)
                                n1671 = Multiply(x=w1451, y=w1452) -> (x*y=w1450:dbl)
                                n1672 = local write "Calendar days required\nfor testing all units"(w1459) -> ()
                                n1673 = local write "$ saved"(w1450) -> ()
                                }
                                }
                                }
                                frame True {
                                n1674 = local read "H1 online"() -> (w1501:bool)
                                n1675 = local read "Tandem\nfloorspace area"() -> (w1513:i32)
                                n1676 = local read "Std cell \nfloorspace area"() -> (w1506:i32)
                                n1677 = case shown="True" w1501 {
                                tunnel: [0 w1515] -> w1481
                                frame False {
                                }
                                frame True {
                                n1678 = local read "H1 UPH"() -> (w1516:cluster{u32, u32})
                                n1679 = Unbundle(w1516) -> (w1515:u32)  [unwired: 1 out]
                                }
                                }
                                n1680 = local read "System UPH"() -> (w1512:u32)
                                n1681 = local read "H2 calc UPH"() -> (w1507:dbl)
                                n1682 = Divide(x=w1512, y=w1513) -> (x/y=w1484:dbl)
                                n1683 = Divide(x=w1507, y=w1506) -> (x/y=w1485:dbl)
                                n1684 = local write "Tandem UPH\nper unit area"(w1484) -> ()
                                n1685 = local write "H2 UPH per unit area"(w1485) -> ()
                                n1686 = local read "Std hourly\ncost ($/hr)"() -> (w1509:dbl)
                                n1687 = local read "H2 UPH"() -> (w1511:cluster{u32, u32})
                                n1688 = local read "Utilization (%)"() -> (w1491:u32)
                                n1689 = local read "Tandem hourly\ncost ($/hr)"() -> (w1510:dbl)
                                n1690 = local read "# of devices to test"() -> (w1497:u32)
                                n1691 = local read "Hours per month"() -> (w1492:i32)
                                n1692 = Unbundle(w1511) -> (w1487:u32)  [unwired: 1 out]
                                n1693 = local write "Calc H1 UPH"(w1481) -> ()
                                n1694 = local write "Calc H2 UPH"(w1487) -> ()
                                n1695 = local read "UPH"() -> (w1508:dbl)
                                n1696 = Add(x=w1481, y=w1487) -> (x+y=w1486:u32)
                                n1697 = Divide(x=w1491, y=u32 100) -> (x/y=w1490:dbl)
                                n1698 = local write "System UPH"(w1486) -> ()
                                n1699 = local write "Calc\nsystem UPH"(w1486) -> ()
                                n1700 = Divide(x=w1497, y=w1486) -> (x/y=w1496:dbl)
                                n1701 = Multiply(x=w1492, y=w1490) -> (x*y=w1488:dbl)
                                n1702 = Divide(x=w1509, y=w1508) -> (x/y=w1505:dbl)
                                n1703 = Divide(x=w1510, y=w1486) -> (x/y=w1503:dbl)
                                n1704 = local read "# of devices to test"() -> (w1499:u32)
                                n1705 = Divide(x=w1496, y=w1488) -> (x/y=w1495:dbl)
                                n1706 = Multiply(x=w1505, y=100.0) -> (x*y=w1483:dbl)
                                n1707 = Multiply(x=w1503, y=100.0) -> (x*y=w1482:dbl)
                                n1708 = local write "Std unit cost\n(cents/device)"(w1483) -> ()
                                n1709 = local write "Tandem unit cost\n(cents/device)"(w1482) -> ()
                                n1710 = Subtract(x=w1483, y=w1482) -> (x-y=w1500:dbl)
                                n1711 = Multiply(x=w1495, y=30) -> (x*y=w1493:dbl)
                                n1712 = Multiply(x=w1499, y=w1500) -> (x*y=w1498:dbl)
                                n1713 = local write "Calendar days required\nfor testing all units"(w1493) -> ()
                                n1714 = local write "$ saved"(w1498) -> ()
                                }
                                }
                                }
                                frame #4 {
                                # "when this loop unlocks the handlers,\nthe handler interface loops are free to continue\nto send the binning information to their\nrespective handlers.  Each handler interface \nloop using the \"binning string hidden\" to do\nthis.  That is why, here, there is no writing of\nthe binning informatrion to a handler.  \nThat is done in the handler interface loops."
                                n1715 = local write "H1 Lock"(FALSE ("H1 Lock")) -> ()
                                n1716 = local write "H2 Lock"(FALSE ("H1 Lock")) -> ()
                                }
                                frame #5 {
                                n1717 = local read "Tester online"() -> (w1519:bool)
                                n1718 = local read "POWER"() -> (w1521:bool)
                                n1719 = Compound Arithmetic op=AND(w1519, w1521) -> (w1520:bool)
                                n1720 = case shown="True" w1520 {
                                frame False {
                                n1721 = local write "SC handler states hid"(SC_handler_states."closing bus" ("SC virtual handler states")) -> ()
                                }
                                frame True {
                                n1722 = local write "SC handler states hid"(SC_handler_states."waiting on event" ("SC virtual handler states")) -> ()
                                }
                                }
                                }
                                }
                              }
                              frame "responding to BINON" {
                                n1723 = local read "Last locked handler hid"() -> (w1524:enum16{"H1", "H2"})
                                n1724 = case shown="\"H1\", Default" w1524 {
                                frame "H1", Default {
                                n1725 = flat-sequence {
                                tunnel: [w1538] -> w1529
                                tunnel: [w1537] -> w1528
                                tunnel: [w1546] -> w1527
                                tunnel: w1528 -> [w1547]
                                tunnel: w1529 -> [w1548]
                                tunnel: w1527 -> [w1566]
                                frame #0 {
                                n1726 = while {
                                i -> [w1530]
                                stop <- w1532 stop-if-true
                                n1727 = local read "NS6040 tester states H1 hid"() -> (w1534:T4)
                                n1728 = Wait (ms)(milliseconds to wait=u32 10) -> ()  [unwired: 1 out]
                                n1729 = Equal?(x=w1534, y=SC_NS6040_tester_states_v2."binning") -> (x = y?=w1532:bool)
                                "Numeric 4" <- w1530
                                }
                                }
                                frame #1 {
                                # "write binning to active handler"
                                n1730 = local read "VISA bus 1 resource name out hid"() -> (w1544:refnum<visa-resource-name>)
                                n1731 = local read "Binning string from tester hid"() -> (w1535:string)
                                n1732 = local read "VISA bus 1 error out hid"() -> (w1545:errorcluster)
                                n1733 = local read "GPIB bus 1 traffic"() -> (w1542:string)
                                n1734 = call <vilib>:"Trim Whitespace.vi"("string"=w1535) -> ("trimmed string"=w1536:string)  [unwired: 1 in]
                                n1735 = VISA Write(VISA resource name=w1544, write buffer=w1535, error in (no error)=w1545) -> (VISA resource name out=w1537:refnum<visa-resource-name>, error out=w1538:errorcluster)  [unwired: 1 out]
                                n1736 = local write "VISA bus 1 error out hid"(w1538) -> ()
                                n1737 = Unbundle By Name(w1538) -> ("status"=w1543:bool)
                                n1738 = Concatenate Strings(w1542, "\r\n", "Bus 1 write: " ("string"), w1536) -> (w1540:string)
                                n1739 = local write "GPIB bus 1 write error"(w1543) -> ()
                                n1740 = local write "GPIB bus 1 traffic"(w1540) -> ()
                                }
                                frame #2 {
                                # "read echo from active handler"
                                n1741 = while {
                                tunnel: w1548 -> [w1565]
                                tunnel: w1547 -> [w1564]
                                tunnel: [w1554] -> w1546
                                i -> [w1549]
                                stop <- w1551 stop-if-true
                                n1742 = local read "GPIB bus 1 traffic"() -> (w1557:string)
                                n1743 = VISA Read(VISA resource name=w1564, byte count=u32 128, error in (no error)=w1565) -> (VISA resource name out=w1562:refnum<visa-resource-name>, read buffer=w1554:string, error out=w1561:errorcluster)  [unwired: 1 out]
                                n1744 = local write "VISA bus 1 resource name out hid"(w1562) -> ()
                                n1745 = Unbundle By Name(w1561) -> ("status"=w1556:bool)
                                n1746 = call <vilib>:"Trim Whitespace.vi"("string"=w1554) -> ("trimmed string"=w1555:string)  [unwired: 1 in]
                                n1747 = local write "GPIB bus 1 read error"(w1556) -> ()
                                n1748 = Match True/False String(2:"X" ("false string"), 3:"ECHO" ("true string"), 4:w1554) -> (0:w1551:bool)  [unwired: 1 out]
                                n1749 = Concatenate Strings(w1557, "\r\n", "Bus 1 read: " ("string"), w1555) -> (w1559:string)
                                n1750 = local write "GPIB bus 1 traffic"(w1559) -> ()
                                n1751 = Wait (ms)(milliseconds to wait=u32 5) -> ()  [unwired: 1 out]
                                "Numeric 5" <- w1549
                                }
                                }
                                frame #3 {
                                # "write echo back to H1"
                                n1752 = call <vilib>:"Trim Whitespace.vi"("string"=w1566) -> ("trimmed string"=w1567:string)  [unwired: 1 in]
                                n1753 = local read "GPIB Bus 0 traffic"() -> (w1572:string)
                                n1754 = local read "VISA bus 0 resource name out hid"() -> (w1576:refnum<visa-resource-name>)
                                n1755 = local read "VISA bus 0 error out hid"() -> (w1575:errorcluster)
                                n1756 = Concatenate Strings(w1572, "\r\n", "Bus 0 write: " ("string"), w1567) -> (w1570:string)
                                n1757 = local write "GPIB Bus 0 traffic"(w1570) -> ()
                                n1758 = VISA Write(VISA resource name=w1576, write buffer=w1566, error in (no error)=w1575) -> (VISA resource name out=w1574:refnum<visa-resource-name>, error out=w1573:errorcluster)  [unwired: 1 out]
                                n1759 = local write "VISA bus 0 resource name out hid"(w1574) -> ()
                                n1760 = Unbundle By Name(w1573) -> ("status"=w1568:bool)
                                n1761 = local write "VISA bus 0 error out hid"(w1573) -> ()
                                n1762 = local write "GPIB bus 0 write error"(w1568) -> ()
                                }
                                frame #4 {
                                # "go wait for results from tester:\nECHONG\nECHOOK\nActive handler is waiting for\nEcho state of tester to become\nECHOOK"
                                n1763 = local write "SC handler states hid"(SC_handler_states."waiting on event" ("SC Test Interface States")) -> ()
                                }
                                }
                                }
                                frame "H2" {
                                n1764 = flat-sequence {
                                tunnel: [w1588] -> w1580
                                tunnel: [w1587] -> w1579
                                tunnel: [w1596] -> w1578
                                tunnel: w1579 -> [w1597]
                                tunnel: w1580 -> [w1598]
                                tunnel: w1578 -> [w1615]
                                frame #0 {
                                n1765 = while {
                                stop <- w1583 stop-if-true
                                n1766 = local read "NS6040 tester states H2 hid"() -> (w1581:T4)
                                n1767 = Wait (ms)(milliseconds to wait=u32 10) -> ()  [unwired: 1 out]
                                n1768 = Equal?(x=w1581, y=SC_NS6040_tester_states_v2."binning") -> (x = y?=w1583:bool)
                                }
                                }
                                frame #1 {
                                n1769 = local read "VISA bus 2 resource name out hid"() -> (w1594:refnum<visa-resource-name>)
                                n1770 = local read "Binning string from tester hid"() -> (w1585:string)
                                n1771 = local read "VISA bus 2 error out hid"() -> (w1595:errorcluster)
                                n1772 = local read "GPIB bus 2 traffic"() -> (w1592:string)
                                n1773 = call <vilib>:"Trim Whitespace.vi"("string"=w1585) -> ("trimmed string"=w1586:string)  [unwired: 1 in]
                                n1774 = VISA Write(VISA resource name=w1594, write buffer=w1585, error in (no error)=w1595) -> (VISA resource name out=w1588:refnum<visa-resource-name>, error out=w1587:errorcluster)  [unwired: 1 out]
                                n1775 = local write "VISA bus 2 error out hid"(w1587) -> ()
                                n1776 = Unbundle By Name(w1587) -> ("status"=w1593:bool)
                                n1777 = Concatenate Strings(w1592, "\r\n", "Bus 2 write: " ("string"), w1586) -> (w1590:string)
                                n1778 = local write "GPIB bus 2 write error"(w1593) -> ()
                                n1779 = local write "GPIB bus 2 traffic"(w1590) -> ()
                                }
                                frame #2 {
                                n1780 = while {
                                tunnel: w1598 -> [w1614]
                                tunnel: w1597 -> [w1613]
                                tunnel: [w1601] -> w1596
                                stop <- w1600 stop-if-true
                                n1781 = local read "GPIB bus 2 traffic"() -> (w1606:string)
                                n1782 = VISA Read(VISA resource name=w1614, byte count=u32 128, error in (no error)=w1613) -> (VISA resource name out=w1611:refnum<visa-resource-name>, read buffer=w1601:string, error out=w1610:errorcluster)  [unwired: 1 out]
                                n1783 = local write "VISA bus 2 resource name out hid"(w1611) -> ()
                                n1784 = Unbundle By Name(w1610) -> ("status"=w1605:bool)
                                n1785 = call <vilib>:"Trim Whitespace.vi"("string"=w1601) -> ("trimmed string"=w1604:string)  [unwired: 1 in]
                                n1786 = local write "GPIB bus 2 read error"(w1605) -> ()
                                n1787 = Match True/False String(2:"X" ("false string"), 3:"ECHO" ("true string"), 4:w1601) -> (0:w1600:bool)  [unwired: 1 out]
                                n1788 = Concatenate Strings(w1606, "\r\n", "Bus 2 read: " ("string"), w1604) -> (w1608:string)
                                n1789 = local write "GPIB bus 2 traffic"(w1608) -> ()
                                n1790 = Wait (ms)(milliseconds to wait=u32 5) -> ()  [unwired: 1 out]
                                }
                                }
                                frame #3 {
                                n1791 = call <vilib>:"Trim Whitespace.vi"("string"=w1615) -> ("trimmed string"=w1617:string)  [unwired: 1 in]
                                n1792 = local read "GPIB Bus 0 traffic"() -> (w1616:string)
                                n1793 = local read "VISA bus 0 resource name out hid"() -> (w1623:refnum<visa-resource-name>)
                                n1794 = local read "VISA bus 0 error out hid"() -> (w1624:errorcluster)
                                n1795 = Concatenate Strings(w1616, "\r\n", "Bus 0 write: " ("string"), w1617) -> (w1619:string)
                                n1796 = local write "GPIB Bus 0 traffic"(w1619) -> ()
                                n1797 = VISA Write(VISA resource name=w1623, write buffer=w1615, error in (no error)=w1624) -> (VISA resource name out=w1622:refnum<visa-resource-name>, error out=w1621:errorcluster)  [unwired: 1 out]
                                n1798 = local write "VISA bus 0 resource name out hid"(w1622) -> ()
                                n1799 = Unbundle By Name(w1621) -> ("status"=w1625:bool)
                                n1800 = local write "VISA bus 0 error out hid"(w1621) -> ()
                                n1801 = local write "GPIB bus 0 write error"(w1625) -> ()
                                }
                                frame #4 {
                                n1802 = local write "SC handler states hid"(SC_handler_states."waiting on event" ("SC Test Interface States")) -> ()
                                }
                                }
                                }
                                }
                              }
                              frame "ECHONG" {
                                n1803 = flat-sequence {
                                frame #0 {
                                n1804 = local read "GPIB Bus 0 traffic"() -> (w1629:string)
                                n1805 = Concatenate Strings(w1629, "\r\n", "Bus 0: ECHONG received from tester" ("string")) -> (w1631:string)
                                n1806 = local write "GPIB Bus 0 traffic"(w1631) -> ()
                                }
                                frame #1 {
                                n1807 = local read "Last locked handler hid"() -> (w1633:enum16{"H1", "H2"})
                                n1808 = case shown="\"H2\"" w1633 {
                                frame "H1", Default {
                                w1634 = "ECHONG\n"
                                n1809 = local read "VISA bus 1 resource name out hid"() -> (w1642:refnum<visa-resource-name>)
                                n1810 = local read "VISA bus 1 error out hid"() -> (w1643:errorcluster)
                                n1811 = local read "GPIB bus 1 traffic"() -> (w1640:string)
                                n1812 = call <vilib>:"Trim Whitespace.vi"("string"=w1634) -> ("trimmed string"=w1635:string)  [unwired: 1 in]
                                n1813 = VISA Write(VISA resource name=w1642, write buffer=w1634, error in (no error)=w1643) -> (error out=w1636:errorcluster)  [unwired: 2 out]
                                n1814 = local write "VISA bus 1 error out hid"(w1636) -> ()
                                n1815 = Unbundle By Name(w1636) -> ("status"=w1641:bool)
                                n1816 = Concatenate Strings(w1640, "\r\n", "Bus 1 write: " ("string"), w1635) -> (w1638:string)
                                n1817 = local write "GPIB bus 1 write error"(w1641) -> ()
                                n1818 = local write "GPIB bus 1 traffic"(w1638) -> ()
                                }
                                frame "H2" {
                                w1644 = "ECHONG\n"
                                n1819 = local read "VISA bus 2 resource name out hid"() -> (w1652:refnum<visa-resource-name>)
                                n1820 = local read "VISA bus 2 error out hid"() -> (w1653:errorcluster)
                                n1821 = local read "GPIB bus 2 traffic"() -> (w1650:string)
                                n1822 = call <vilib>:"Trim Whitespace.vi"("string"=w1644) -> ("trimmed string"=w1645:string)  [unwired: 1 in]
                                n1823 = VISA Write(VISA resource name=w1652, write buffer=w1644, error in (no error)=w1653) -> (error out=w1646:errorcluster)  [unwired: 2 out]
                                n1824 = local write "VISA bus 2 error out hid"(w1646) -> ()
                                n1825 = Unbundle By Name(w1646) -> ("status"=w1651:bool)
                                n1826 = Concatenate Strings(w1650, "\r\n", "Bus 2 write: " ("string"), w1645) -> (w1648:string)
                                n1827 = local write "GPIB bus 2 write error"(w1651) -> ()
                                n1828 = local write "GPIB bus 2 traffic"(w1648) -> ()
                                }
                                }
                                }
                                frame #2 {
                                n1829 = local write "SC handler states hid"(SC_handler_states."waiting on event" ("SC Test Interface States")) -> ()
                                }
                                }
                              }
                              frame "ECHOOK" {
                                n1830 = flat-sequence {
                                frame #0 {
                                n1831 = local read "GPIB Bus 0 traffic"() -> (w1657:string)
                                n1832 = Concatenate Strings(w1657, "\r\n", "Bus 0: ECHOOK received from tester." ("string")) -> (w1659:string)
                                n1833 = local write "GPIB Bus 0 traffic"(w1659) -> ()
                                }
                                frame #1 {
                                n1834 = local read "Last locked handler hid"() -> (w1661:enum16{"H1", "H2"})
                                n1835 = case shown="\"H1\", Default" w1661 {
                                frame "H1", Default {
                                w1662 = "ECHOOK\n"
                                n1836 = local read "VISA bus 1 resource name out hid"() -> (w1670:refnum<visa-resource-name>)
                                n1837 = local read "VISA bus 1 error out hid"() -> (w1671:errorcluster)
                                n1838 = local read "GPIB bus 1 traffic"() -> (w1668:string)
                                n1839 = call <vilib>:"Trim Whitespace.vi"("string"=w1662) -> ("trimmed string"=w1663:string)  [unwired: 1 in]
                                n1840 = VISA Write(VISA resource name=w1670, write buffer=w1662, error in (no error)=w1671) -> (error out=w1664:errorcluster)  [unwired: 2 out]
                                n1841 = local write "VISA bus 1 error out hid"(w1664) -> ()
                                n1842 = Unbundle By Name(w1664) -> ("status"=w1669:bool)
                                n1843 = Concatenate Strings(w1668, "\r\n", "Bus 1 write: " ("string"), w1663) -> (w1666:string)
                                n1844 = local write "GPIB bus 1 write error"(w1669) -> ()
                                n1845 = local write "GPIB bus 1 traffic"(w1666) -> ()
                                }
                                frame "H2" {
                                w1672 = "ECHOOK\n"
                                n1846 = local read "VISA bus 2 resource name out hid"() -> (w1680:refnum<visa-resource-name>)
                                n1847 = local read "VISA bus 2 error out hid"() -> (w1681:errorcluster)
                                n1848 = local read "GPIB bus 2 traffic"() -> (w1678:string)
                                n1849 = call <vilib>:"Trim Whitespace.vi"("string"=w1672) -> ("trimmed string"=w1673:string)  [unwired: 1 in]
                                n1850 = VISA Write(VISA resource name=w1680, write buffer=w1672, error in (no error)=w1681) -> (error out=w1674:errorcluster)  [unwired: 2 out]
                                n1851 = local write "VISA bus 2 error out hid"(w1674) -> ()
                                n1852 = Unbundle By Name(w1674) -> ("status"=w1679:bool)
                                n1853 = Concatenate Strings(w1678, "\r\n", "Bus 2 write: " ("string"), w1673) -> (w1676:string)
                                n1854 = local write "GPIB bus 2 write error"(w1679) -> ()
                                n1855 = local write "GPIB bus 2 traffic"(w1676) -> ()
                                }
                                }
                                }
                                frame #2 {
                                n1856 = Tick Count (ms)() -> (millisecond timer value=w1682:u32)
                                n1857 = Tick Count (ms)() -> (millisecond timer value=w1683:u32)
                                n1858 = local write "tester wt start hid"(w1682) -> ()
                                n1859 = local write "tester tt end hid"(w1683) -> ()
                                }
                                frame #3 {
                                n1860 = local read "tester tt start hid"() -> (w1687:u32)
                                n1861 = local read "tester tt end hid"() -> (w1688:u32)
                                n1862 = Subtract(x=w1688, y=w1687) -> (x-y=w1686:u32)
                                n1863 = Divide(x=w1686, y=u32 1000) -> (x/y=w1684:dbl)
                                n1864 = local write "SC measured test time hid"(w1684) -> ()
                                }
                                frame #4 {
                                n1865 = local read "Last locked handler hid"() -> (w1689:enum16{"H1", "H2"})
                                n1866 = case shown="\"H2\"" w1689 {
                                frame "H1", Default {
                                n1867 = local read "Tandem\nfloorspace area"() -> (w1722:i32)
                                n1868 = local read "Std cell \nfloorspace area"() -> (w1715:i32)
                                n1869 = local read "System UPH"() -> (w1721:u32)
                                n1870 = local read "H2 calc UPH"() -> (w1716:dbl)
                                n1871 = local read "H1 UPH"() -> (w1690:cluster{u32, u32})
                                n1872 = Divide(x=w1721, y=w1722) -> (x/y=w1694:dbl)
                                n1873 = Divide(x=w1716, y=w1715) -> (x/y=w1695:dbl)
                                n1874 = local read "Std hourly\ncost ($/hr)"() -> (w1718:dbl)
                                n1875 = Unbundle(w1690) -> (w1691:u32)  [unwired: 1 out]
                                n1876 = local write "Tandem UPH\nper unit area"(w1694) -> ()
                                n1877 = local write "H2 UPH per unit area"(w1695) -> ()
                                n1878 = local read "H2 UPH"() -> (w1720:cluster{u32, u32})
                                n1879 = local read "Tandem hourly\ncost ($/hr)"() -> (w1719:dbl)
                                n1880 = local read "Utilization (%)"() -> (w1701:u32)
                                n1881 = local read "# of devices to test"() -> (w1707:u32)
                                n1882 = local read "Hours per month"() -> (w1702:i32)
                                n1883 = Unbundle(w1720) -> (w1697:u32)  [unwired: 1 out]
                                n1884 = local write "Calc H1 UPH"(w1691) -> ()
                                n1885 = local write "Calc H2 UPH"(w1697) -> ()
                                n1886 = local read "UPH"() -> (w1717:dbl)
                                n1887 = Add(x=w1691, y=w1697) -> (x+y=w1696:u32)
                                n1888 = Divide(x=w1701, y=u32 100) -> (x/y=w1700:dbl)
                                n1889 = Divide(x=w1718, y=w1717) -> (x/y=w1714:dbl)
                                n1890 = Divide(x=w1719, y=w1696) -> (x/y=w1712:dbl)
                                n1891 = Divide(x=w1707, y=w1696) -> (x/y=w1706:dbl)
                                n1892 = Multiply(x=w1702, y=w1700) -> (x*y=w1698:dbl)
                                n1893 = local write "System UPH"(w1696) -> ()
                                n1894 = local write "Calc\nsystem UPH"(w1696) -> ()
                                n1895 = local read "# of devices to test"() -> (w1709:u32)
                                n1896 = Divide(x=w1706, y=w1698) -> (x/y=w1705:dbl)
                                n1897 = Multiply(x=w1714, y=100.0) -> (x*y=w1693:dbl)
                                n1898 = Multiply(x=w1712, y=100.0) -> (x*y=w1692:dbl)
                                n1899 = Subtract(x=w1693, y=w1692) -> (x-y=w1710:dbl)
                                n1900 = Multiply(x=w1705, y=30) -> (x*y=w1703:dbl)
                                n1901 = local write "Tandem unit cost\n(cents/device)"(w1692) -> ()
                                n1902 = local write "Std unit cost\n(cents/device)"(w1693) -> ()
                                n1903 = Multiply(x=w1709, y=w1710) -> (x*y=w1708:dbl)
                                n1904 = local write "Calendar days required\nfor testing all units"(w1703) -> ()
                                n1905 = local write "$ saved"(w1708) -> ()
                                }
                                frame "H2" {
                                n1906 = local read "Tandem\nfloorspace area"() -> (w1726:i32)
                                n1907 = local read "Std cell \nfloorspace area"() -> (w1753:i32)
                                n1908 = local read "System UPH"() -> (w1725:u32)
                                n1909 = local read "H2 UPH"() -> (w1723:cluster{u32, u32})
                                n1910 = local read "UPH"() -> (w1754:dbl)
                                n1911 = Divide(x=w1725, y=w1726) -> (x/y=w1724:dbl)
                                n1912 = local read "Std hourly\ncost ($/hr)"() -> (w1750:dbl)
                                n1913 = Divide(x=w1754, y=w1753) -> (x/y=w1755:dbl)
                                n1914 = Unbundle(w1723) -> (w1743:u32)  [unwired: 1 out]
                                n1915 = local write "Tandem UPH\nper unit area"(w1724) -> ()
                                n1916 = local read "H1 UPH"() -> (w1752:cluster{u32, u32})
                                n1917 = local read "Tandem hourly\ncost ($/hr)"() -> (w1751:dbl)
                                n1918 = local read "Utilization (%)"() -> (w1736:u32)
                                n1919 = local write "H1 UPH per unit area"(w1755) -> ()
                                n1920 = local read "# of devices to test"() -> (w1742:u32)
                                n1921 = local read "Hours per month"() -> (w1737:i32)
                                n1922 = Unbundle(w1752) -> (w1744:u32)  [unwired: 1 out]
                                n1923 = local write "Calc H1 UPH"(w1744) -> ()
                                n1924 = local write "Calc H2 UPH"(w1743) -> ()
                                n1925 = local read "UPH"() -> (w1749:dbl)
                                n1926 = Add(x=w1744, y=w1743) -> (x+y=w1732:u32)
                                n1927 = Divide(x=w1736, y=u32 100) -> (x/y=w1735:dbl)
                                n1928 = Divide(x=w1750, y=w1749) -> (x/y=w1748:dbl)
                                n1929 = Divide(x=w1751, y=w1732) -> (x/y=w1746:dbl)
                                n1930 = Divide(x=w1742, y=w1732) -> (x/y=w1741:dbl)
                                n1931 = Multiply(x=w1737, y=w1735) -> (x*y=w1733:dbl)
                                n1932 = local write "System UPH"(w1732) -> ()
                                n1933 = local write "Calc\nsystem UPH"(w1732) -> ()
                                n1934 = local read "# of devices to test"() -> (w1730:u32)
                                n1935 = Divide(x=w1741, y=w1733) -> (x/y=w1740:dbl)
                                n1936 = Multiply(x=w1748, y=100.0) -> (x*y=w1728:dbl)
                                n1937 = Multiply(x=w1746, y=100.0) -> (x*y=w1727:dbl)
                                n1938 = Subtract(x=w1728, y=w1727) -> (x-y=w1731:dbl)
                                n1939 = Multiply(x=w1740, y=30) -> (x*y=w1738:dbl)
                                n1940 = local write "Tandem unit cost\n(cents/device)"(w1727) -> ()
                                n1941 = local write "Std unit cost\n(cents/device)"(w1728) -> ()
                                n1942 = Multiply(x=w1730, y=w1731) -> (x*y=w1729:dbl)
                                n1943 = local write "Calendar days required\nfor testing all units"(w1738) -> ()
                                n1944 = local write "$ saved"(w1729) -> ()
                                }
                                }
                                }
                                frame #5 {
                                n1945 = local read "Tester online"() -> (w1756:bool)
                                n1946 = local read "POWER"() -> (w1758:bool)
                                n1947 = Compound Arithmetic op=AND(w1756, w1758) -> (w1757:bool)
                                n1948 = case shown="True" w1757 {
                                frame False {
                                n1949 = local write "SC handler states hid"(SC_handler_states."closing bus" ("SC virtual handler states")) -> ()
                                }
                                frame True {
                                n1950 = local write "SC handler states hid"(SC_handler_states."waiting on serial poll" ("SC Test Interface States")) -> ()
                                }
                                }
                                }
                                }
                              }
                              frame "closing bus" {
                                n1951 = flat-sequence {
                                frame #0 {
                                n1952 = local read "GPIB Bus 0 traffic"() -> (w1766:string)
                                n1953 = Concatenate Strings(w1766, "\r\n", "Bus 0 closing" ("string")) -> (w1764:string)
                                n1954 = local write "GPIB Bus 0 traffic"(w1764) -> ()
                                }
                                frame #1 {
                                n1955 = local read "VISA bus 0 resource name out hid"() -> (w1768:refnum<visa-resource-name>)
                                n1956 = local read "VISA bus 0 error out hid"() -> (w1769:errorcluster)
                                n1957 = VISA Close(VISA resource name=w1768, error in (no error)=w1769) -> (error out=w1767:errorcluster)
                                n1958 = Unbundle By Name(w1767) -> ("status"=w1770:bool)
                                n1959 = local write "VISA bus 0 close error"(w1770) -> ()
                                }
                                frame #2 {
                                n1960 = local write "Exit SC handler StMach hid"(TRUE ("Exit tester state machine hid")) -> ()
                                }
                                }
                              }
                              frame "responding to unknown command" {
                                n1961 = flat-sequence {
                                frame #0 {
                                n1962 = local read "GPIB Bus 0 traffic"() -> (w1778:string)
                                n1963 = Concatenate Strings(w1778, "\r\n", "Bus 0 write: " ("string"), "unrecognized string") -> (w1776:string)
                                n1964 = local write "GPIB Bus 0 traffic"(w1776) -> ()
                                }
                                frame #1 {
                                n1965 = local write "SC handler states hid"(SC_handler_states."waiting on event" ("SC Test Interface States")) -> ()
                                }
                                }
                              }
                            }
                          }
                          frame #1 {
                            n1966 = local read "Slow for  Diagnostics"() -> (w1780:bool)
                            n1967 = case shown="False" w1780 {
                              frame False {
                              }
                              frame True {
                                n1968 = local read "GPIB wait time (ms)"() -> (w1783:u32)
                                n1969 = Wait (ms)(milliseconds to wait=w1783) -> ()  [unwired: 1 out]
                              }
                            }
                          }
                        }
                        n1970 = Wait (ms)(milliseconds to wait=u32 5) -> ()  [unwired: 1 out]
                        n1971 = local read "Exit SC handler StMach hid"() -> (w993:bool)
                      }
                    }
                  }
                }
              }
              n1972 = Wait (ms)(milliseconds to wait=u32 5) -> ()  [unwired: 1 out]
              n1973 = local read "POWER"() -> (w980:bool)
            }
            n1974 = while {
              stop <- w360 continue-if-true
              n1975 = local read "H1 online"() -> (w361:bool)
              n1976 = case shown="True" w361 {
                frame False {
                }
                frame True {
                  n1977 = flat-sequence {
                    frame #0 {
                      n1978 = local write "Exit SC tester H1 StMach hid"(FALSE ("Exit H1 state machine hid")) -> ()
                    }
                    frame #1 {
                      n1979 = local read "H1 handler type"() -> (w363:T2)
                      n1980 = case shown="\"Seiko-Epson NS6040\"" w363 {
                        frame "Multitest", Default {
                          n1981 = local write "MT99XX tester states H1 hid"(SC_MT99XX_tester_states."initializing bus" ("SC virtual tester states")) -> ()
                          n1982 = flat-sequence {
                            frame #0 {
                              n1983 = local read "MT99XX tester states H1 hid"() -> (w365:T5)
                              n1984 = case shown="\"binning\"" w365 {
                                frame "initializing bus", Default {
                                n1985 = flat-sequence {
                                frame #0 {
                                # "bus 1"
                                n1986 = local read "GPIB wait timeout hid"() -> (w369:u32)
                                n1987 = local read "SentCtrl talks to handler 1 at"() -> (w370:refnum<visa-resource-name>)
                                n1988 = local read "GPIB wait timeout hid"() -> (w368:u32)
                                n1989 = VISA Open(timeout (0)=w369, VISA resource name=w370) -> (VISA resource name=w367:refnum<visa-resource-name>, error out=w372:errorcluster)  [unwired: 3 in]
                                n1990 = property class="GPIB Instr"(reference=w367, error in=w372, "Timeout"=w368) -> (error out=w366:errorcluster)  [unwired: 1 out]
                                n1991 = local write "VISA bus 1 resource name out hid"(w367) -> ()
                                n1992 = Unbundle By Name(w366) -> ("status"=w371:bool)
                                n1993 = local write "VISA bus 1 open error"(w371) -> ()
                                n1994 = local write "VISA bus 1 error out hid"(w366) -> ()
                                }
                                frame #1 {
                                n1995 = local write "Exit SC tester H1 StMach hid"(FALSE ("Exit H1 state machine hid")) -> ()
                                n1996 = Concatenate Strings("Bus 1 initializing" ("string"), "\r\n") -> (w375:string)
                                n1997 = local write "GPIB bus 1 traffic"(w375) -> ()
                                }
                                frame #2 {
                                n1998 = local write "MT99XX tester states H1 hid"(SC_MT99XX_tester_states."sending *IDN?" ("SC virtual tester states")) -> ()
                                }
                                }
                                }
                                frame "sending *IDN?" {
                                n1999 = flat-sequence {
                                tunnel: [w387] -> w380
                                tunnel: [w386] -> w379
                                tunnel: w380 -> [w401]
                                tunnel: w379 -> [w400]
                                tunnel: [w391] -> w378
                                tunnel: w378 -> [w402]
                                frame #0 {
                                w381 = "*IDN?"
                                n2000 = local read "VISA bus 1 resource name out hid"() -> (w390:refnum<visa-resource-name>)
                                n2001 = local read "GPIB bus 1 traffic"() -> (w385:string)
                                n2002 = local read "VISA bus 1 error out hid"() -> (w389:errorcluster)
                                n2003 = Concatenate Strings(w385, "\r\n", "Bus 1 write: " ("string"), w381) -> (w383:string)
                                n2004 = VISA Write(VISA resource name=w390, write buffer=w381, error in (no error)=w389) -> (VISA resource name out=w387:refnum<visa-resource-name>, error out=w386:errorcluster)  [unwired: 1 out]
                                n2005 = Unbundle By Name(w386) -> ("status"=w388:bool)
                                n2006 = local write "GPIB bus 1 traffic"(w383) -> ()
                                n2007 = local write "GPIB bus 1 write error"(w388) -> ()
                                }
                                frame #1 {
                                n2008 = local read "GPIB bus 1 traffic"() -> (w393:string)
                                n2009 = VISA Read(VISA resource name=w401, byte count=u32 256, error in (no error)=w400) -> (VISA resource name out=w398:refnum<visa-resource-name>, read buffer=w392:string, error out=w397:errorcluster)  [unwired: 1 out]
                                n2010 = local write "VISA bus 1 resource name out hid"(w398) -> ()
                                n2011 = Unbundle By Name(w397) -> ("status"=w391:bool)
                                n2012 = local write "H1 response to *IDN? hid"(w392) -> ()
                                n2013 = local write "GPIB bus 1 read error"(w391) -> ()
                                n2014 = Concatenate Strings(w393, "\r\n", "Bus 1 read: " ("string"), w392) -> (w395:string)
                                n2015 = local write "GPIB bus 1 traffic"(w395) -> ()
                                }
                                frame #2 {
                                n2016 = case shown="True" w402 {
                                frame False {
                                n2017 = local write "MT99XX tester states H1 hid"(SC_MT99XX_tester_states."polling *SITES?" ("SC virtual tester states")) -> ()
                                }
                                frame True {
                                n2018 = flat-sequence {
                                frame #0 {
                                n2019 = while {
                                stop <- w405 stop-if-true
                                n2020 = One Button Dialog(message="Warning:\nVirtual tester does not get a response\nto *IDN? from handler 1.\nCheck GPIB cable and that  handler 1 \nis running and ready to issue a start of test\nby responding with sites ready.", button name ("OK")="Dismiss and retry") -> (true=w405:bool)
                                n2021 = Wait (ms)(milliseconds to wait=u32 100) -> ()  [unwired: 1 out]
                                }
                                }
                                frame #1 {
                                n2022 = local write "H1 online"(FALSE ("H1 online")) -> ()
                                }
                                frame #2 {
                                n2023 = local write "MT99XX tester states H1 hid"(SC_MT99XX_tester_states."sending *IDN?" ("SC virtual tester states")) -> ()
                                }
                                }
                                }
                                }
                                }
                                }
                                }
                                frame "polling *SITES?" {
                                n2024 = flat-sequence {
                                tunnel: [w413] -> w411
                                tunnel: [w412] -> w410
                                tunnel: w411 -> [w449]
                                tunnel: w410 -> [w448]
                                frame #0 {
                                n2025 = while {
                                tunnel: [w417] -> w413
                                tunnel: [w415] -> w412
                                stop <- w414 stop-if-true
                                n2026 = stacked-sequence {
                                tunnel: [w429] -> w419
                                tunnel: [w428] -> w418
                                frame #0 {
                                w421 = "*SITES?"
                                n2027 = local read "VISA bus 1 resource name out hid"() -> (w427:refnum<visa-resource-name>)
                                n2028 = local read "VISA bus 1 error out hid"() -> (w426:errorcluster)
                                n2029 = Concatenate Strings("Handler 1 cycle start" ("string"), "\r\n", "Bus 1 write: " ("string"), w421) -> (w423:string)
                                n2030 = VISA Write(VISA resource name=w427, write buffer=w421, error in (no error)=w426) -> (VISA resource name out=w429:refnum<visa-resource-name>, error out=w428:errorcluster)  [unwired: 1 out]
                                n2031 = Unbundle By Name(w428) -> ("status"=w425:bool)
                                n2032 = local write "GPIB bus 1 traffic"(w423) -> ()
                                n2033 = local write "GPIB bus 1 write error"(w425) -> ()
                                }
                                }
                                n2034 = Wait (ms)(milliseconds to wait=u32 1) -> ()  [unwired: 1 out]
                                n2035 = flat-sequence {
                                tunnel: w419 -> [w447]
                                tunnel: w418 -> [w446]
                                tunnel: [w434] -> w417
                                tunnel: [w430] -> w415
                                tunnel: [w431] -> w414
                                frame #0 {
                                n2036 = local read "GPIB bus 1 traffic"() -> (w439:string)
                                n2037 = VISA Read(VISA resource name=w447, byte count=u32 128, error in (no error)=w446) -> (read buffer=w434:string, error out=w433:errorcluster)  [unwired: 2 out]
                                n2038 = Unbundle By Name(w433) -> ("status"=w430:bool)
                                n2039 = String Length(string=w434) -> (length=w436:i32)
                                n2040 = Scan Value(string=w434, format string="%b", default (0 dbl)=u8 0) -> (value=w438:u8)  [unwired: 1 out]
                                n2041 = Concatenate Strings(w439, "\r\n", "Bus 1 read: " ("string"), w434) -> (w441:string)
                                n2042 = local write "GPIB bus 1 read error"(w430) -> ()
                                n2043 = Greater Than 0?(x=w436) -> (x > 0?=w435:bool)
                                n2044 = Greater Than 0?(x=w438) -> (x > 0?=w437:bool)
                                n2045 = local write "GPIB bus 1 traffic"(w441) -> ()
                                n2046 = And(x=w435, y=w437) -> (x .and. y?=w432:bool)
                                n2047 = Or(x=w432, y=w430) -> (x .or. y?=w431:bool)
                                }
                                }
                                }
                                }
                                frame #1 {
                                n2048 = case shown="False" w448 {
                                tunnel: w449 -> [w450 _]
                                frame False {
                                n2049 = flat-sequence {
                                tunnel: w450 -> [w451]
                                frame #0 {
                                n2050 = String Length(string=w451) -> (length=w452:i32)
                                n2051 = local write "H1 SITES? response hid"(w451) -> ()
                                n2052 = local write "H1 parallelism"(w452) -> ()
                                }
                                frame #1 {
                                # "This block adds zeroes (sites not ready)\nto SITES READY from handlers when the\nhandler is running at a lower parallelism\nthan the test program, but has the same\npin mapping for the active sites in common."
                                n2053 = local read "Program Parallelism"() -> (w456:u32)
                                n2054 = local read "H1 allow lower parallelism"() -> (w455:bool)
                                n2055 = local read "H1 parallelism"() -> (w457:u32)
                                n2056 = Less?(x=w457, y=w456) -> (x < y?=w454:bool)
                                n2057 = And(x=w454, y=w455) -> (x .and. y?=w453:bool)
                                n2058 = case shown="True" w453 {
                                frame False {
                                n2059 = local read "Program Parallelism"() -> (w460:u32)
                                n2060 = local read "H1 parallelism"() -> (w458:u32)
                                n2061 = Greater?(x=w458, y=w460) -> (0:w459:bool)
                                n2062 = case shown="True" w459 {
                                frame False {
                                # "parallelisms must match if arriving here"
                                n2063 = local write "MT99XX tester states H1 hid"(SC_MT99XX_tester_states."testing" ("SC virtual tester states")) -> ()
                                }
                                frame True {
                                n2064 = local write "MT99XX tester states H1 hid"(SC_MT99XX_tester_states."closing bus" ("SC virtual tester states")) -> ()
                                n2065 = local write "POWER"(FALSE ("POWER")) -> ()
                                n2066 = One Button Dialog(message="Fatal error 300:\nTest program cannot support higher\nparallelism on handler 1.\nThe Sentinel Controller program is shutting down.\nPlease correct the mismatch and restart.") -> ()  [unwired: 1 in, 1 out]
                                }
                                }
                                }
                                frame True {
                                n2067 = local read "Program Parallelism"() -> (w470:u32)
                                n2068 = local read "H1 parallelism"() -> (w467:u32)
                                n2069 = local read "H1 SITES? response hid"() -> (w468:string)
                                n2070 = Subtract(x=w470, y=w467) -> (x-y=w469:u32)
                                n2071 = for {
                                N: w469 -> [_]
                                shift-right: [w471] -> w465
                                shift-left: w468 -> [w472]
                                n2072 = Concatenate Strings(w472, "0" ("string")) -> (w471:string)
                                }
                                n2073 = local write "H1 SITES? response hid"(w465) -> ()
                                n2074 = local write "MT99XX tester states H1 hid"(SC_MT99XX_tester_states."testing" ("SC virtual tester states")) -> ()
                                }
                                }
                                }
                                frame #2 {
                                n2075 = Tick Count (ms)() -> (millisecond timer value=w478:u32)
                                n2076 = Tick Count (ms)() -> (millisecond timer value=w477:u32)
                                n2077 = local write "H1 wt start hidden"(w478) -> ()
                                n2078 = local write "H1 it end hidden"(w477) -> ()
                                n2079 = local write "H1 Waiting"(TRUE ("H2 Waiting")) -> ()
                                n2080 = local write "H1 Indexing"(FALSE ("h1 indexing")) -> ()
                                n2081 = local write "H1 Testing"(FALSE ("h1 indexing")) -> ()
                                }
                                frame #3 {
                                n2082 = local read "H1 it start hidden"() -> (w482:u32)
                                n2083 = local read "H1 it end hidden"() -> (w483:u32)
                                n2084 = Subtract(x=w483, y=w482) -> (x-y=w479:u32)
                                n2085 = Divide(x=w479, y=u32 1000) -> (x/y=w481:dbl)
                                n2086 = local write "MT99XX tester states H1 hid"(SC_MT99XX_tester_states."testing" ("SC virtual tester states")) -> ()
                                n2087 = local write "H1 measured Index Time"(w481) -> ()
                                }
                                }
                                }
                                frame True {
                                n2088 = flat-sequence {
                                frame #0 {
                                n2089 = local read "VISA bus 1 resource name out hid"() -> (w487:refnum<visa-resource-name>)
                                n2090 = local read "VISA bus 1 error out hid"() -> (w488:errorcluster)
                                n2091 = VISA Close(VISA resource name=w487, error in (no error)=w488) -> (error out=w486:errorcluster)
                                n2092 = Unbundle By Name(w486) -> ("status"=w485:bool)
                                n2093 = local write "VISA bus 1 close error"(w485) -> ()
                                }
                                frame #1 {
                                n2094 = local write "VISA bus 1 close error"(FALSE ("VISA bus 1 close error")) -> ()
                                n2095 = Concatenate Strings("Bus 1 error  while reading,\nclosing Bus 1 and re-initializing" ("string"), "\r\n") -> (w491:string)
                                n2096 = local write "GPIB bus 1 traffic"(w491) -> ()
                                }
                                frame #2 {
                                n2097 = local write "MT99XX tester states H1 hid"(SC_MT99XX_tester_states."initializing bus" ("SC virtual tester states")) -> ()
                                }
                                }
                                }
                                }
                                }
                                }
                                }
                                frame "testing" {
                                n2098 = flat-sequence {
                                frame #0 {
                                n2099 = while {
                                stop <- w494 stop-if-true
                                n2100 = local read "H1 Lock"() -> (w494:bool)
                                n2101 = Wait (ms)(milliseconds to wait=u32 1) -> ()  [unwired: 1 out]
                                }
                                }
                                frame #1 {
                                n2102 = Tick Count (ms)() -> (millisecond timer value=w505:u32)
                                n2103 = Tick Count (ms)() -> (millisecond timer value=w504:u32)
                                n2104 = local write "H1 Testing"(TRUE ("testing")) -> ()
                                n2105 = local write "H1 Indexing"(FALSE ("waiting")) -> ()
                                n2106 = local write "H1 Waiting"(FALSE ("H1 Waiting")) -> ()
                                n2107 = local write "H1 wt end hidden"(w505) -> ()
                                n2108 = local write "H1 tt start hidden"(w504) -> ()
                                n2109 = local read "GPIB bus 1 traffic"() -> (w497:string)
                                n2110 = Concatenate Strings(w497, "\r\n", "Bus 1: " ("string"), "testing" ("string")) -> (w499:string)
                                n2111 = local write "GPIB bus 1 traffic"(w499) -> ()
                                }
                                frame #2 {
                                n2112 = local read "H1 wt start hidden"() -> (w509:u32)
                                n2113 = local read "H1 wt end hidden"() -> (w510:u32)
                                n2114 = Subtract(x=w510, y=w509) -> (x-y=w508:u32)
                                n2115 = Divide(x=w508, y=u32 1000) -> (x/y=w506:dbl)
                                n2116 = local write "H1 measured Wait Time"(w506) -> ()
                                }
                                frame #3 {
                                n2117 = local write "MT99XX tester states H1 hid"(SC_MT99XX_tester_states."binning" ("SC virtual tester states")) -> ()
                                }
                                }
                                }
                                frame "binning" {
                                n2118 = flat-sequence {
                                tunnel: [w523] -> w514
                                tunnel: [w550] -> w515
                                tunnel: w514 -> [w550]
                                tunnel: w515 -> [w557]
                                tunnel: [w556] -> w513
                                tunnel: [w555] -> w512
                                tunnel: w513 -> [w608]
                                tunnel: w512 -> [w607]
                                frame #0 {
                                n2119 = while {
                                stop <- w517 continue-if-true
                                n2120 = local read "H1 Lock"() -> (w517:bool)
                                n2121 = Wait (ms)(milliseconds to wait=u32 1) -> ()  [unwired: 1 out]
                                }
                                }
                                frame #1 {
                                n2122 = local read "Program Parallelism"() -> (w521:u32)
                                n2123 = local read "H1 parallelism"() -> (w522:u32)
                                n2124 = Less?(x=w522, y=w521) -> (x < y?=w519:bool)
                                n2125 = local read "H1 allow lower parallelism"() -> (w520:bool)
                                n2126 = And(x=w519, y=w520) -> (x .and. y?=w518:bool)
                                n2127 = case shown="False" w518 {
                                tunnel: [w524 w535] -> w523
                                frame False {
                                n2128 = local read "VISA bus 1 resource name out hid"() -> (w532:refnum<visa-resource-name>)
                                n2129 = local read "Binning string from tester hid"() -> (w524:string)
                                n2130 = local read "VISA bus 1 error out hid"() -> (w533:errorcluster)
                                n2131 = local read "GPIB bus 1 traffic"() -> (w528:string)
                                n2132 = VISA Write(VISA resource name=w532, write buffer=w524, error in (no error)=w533) -> (VISA resource name out=w530:refnum<visa-resource-name>, error out=w531:errorcluster)  [unwired: 1 out]
                                n2133 = local write "VISA bus 1 resource name out hid"(w530) -> ()
                                n2134 = local write "VISA bus 1 error out hid"(w531) -> ()
                                n2135 = Unbundle By Name(w531) -> ("status"=w529:bool)
                                n2136 = Concatenate Strings(w528, "\r\n", "Bus 1 write: " ("string"), w524) -> (w526:string)
                                n2137 = local write "GPIB bus 1 write error"(w529) -> ()
                                n2138 = local write "GPIB bus 1 traffic"(w526) -> ()
                                }
                                frame True {
                                n2139 = local read "H1 parallelism"() -> (w534:u32)
                                n2140 = local read "Binning string from tester hid"() -> (w536:string)
                                n2141 = local read "VISA bus 1 resource name out hid"() -> (w547:refnum<visa-resource-name>)
                                n2142 = local read "VISA bus 1 error out hid"() -> (w548:errorcluster)
                                n2143 = Multiply(x=w534, y=u32 8) -> (x*y=w538:u32)
                                n2144 = local read "GPIB bus 1 traffic"() -> (w543:string)
                                n2145 = Decrement(x=w538) -> (x-1=w539:u32)
                                n2146 = String Subset(string=w536, length (rest)=w539) -> (substring=w535:string)  [unwired: 1 in]
                                n2147 = VISA Write(VISA resource name=w547, write buffer=w535, error in (no error)=w548) -> (VISA resource name out=w545:refnum<visa-resource-name>, error out=w546:errorcluster)  [unwired: 1 out]
                                n2148 = local write "VISA bus 1 resource name out hid"(w545) -> ()
                                n2149 = local write "VISA bus 1 error out hid"(w546) -> ()
                                n2150 = Unbundle By Name(w546) -> ("status"=w544:bool)
                                n2151 = Concatenate Strings(w543, "\r\n", "Bus 1 write: " ("string"), w535) -> (w541:string)
                                n2152 = local write "GPIB bus 1 traffic"(w541) -> ()
                                n2153 = local write "GPIB bus 1 write error"(w544) -> ()
                                }
                                }
                                }
                                frame #2 {
                                n2154 = local write "H1 Waiting"(FALSE ("waiting")) -> ()
                                n2155 = Tick Count (ms)() -> (millisecond timer value=w551:u32)
                                n2156 = Tick Count (ms)() -> (millisecond timer value=w552:u32)
                                n2157 = local write "H1 tt end hidden"(w551) -> ()
                                n2158 = local write "H1 it start hidden"(w552) -> ()
                                n2159 = local write "H1 Indexing"(TRUE ("waiting")) -> ()
                                n2160 = local write "H1 Testing"(FALSE ("waiting")) -> ()
                                }
                                frame #3 {
                                n2161 = local read "H1 tt start hidden"() -> (w561:u32)
                                n2162 = local read "H1 tt end hidden"() -> (w562:u32)
                                n2163 = while {
                                tunnel: [w580] -> w576 mode=indexing
                                shift-right: [w581] -> _
                                shift-left: w557 -> [w583]
                                stop <- w578 stop-if-true
                                n2164 = Match Pattern(string=w583, regular expression=" ") -> (before substring=w580:string, after substring=w581:string, offset past match=w579:i32)  [unwired: 2 out]
                                n2165 = Less Than 0?(x=w579) -> (x < 0?=w578:bool)
                                }
                                n2166 = Subtract(x=w562, y=w561) -> (x-y=w560:u32)
                                n2167 = Divide(x=w560, y=u32 1000) -> (x/y=w558:dbl)
                                n2168 = local write "H1 measured Test Time"(w558) -> ()
                                n2169 = Array Size(array=w576) -> (size(s)=w573:i32)
                                n2170 = Divide(x=w573, y=3) -> (x/y=w575:dbl)
                                n2171 = To Unsigned Byte Integer(number=w575) -> (unsigned 8bit integer=w571:u8)
                                n2172 = local read "H1 SITES? response hid"() -> (w568:string)
                                n2173 = local read "H1 parallelism"() -> (w567:u32)
                                n2174 = Not Equal?(x=w567, y=w571) -> (x != y?=w572:bool)
                                n2175 = for {
                                N: w571 -> [_]
                                tunnel: w576 -> [w606]
                                tunnel: w568 -> [w597]
                                shift-right: [w590] -> w555
                                shift-left: 0 -> [w589]
                                shift-right: [w586] -> w556
                                shift-left: 0 -> [w584]
                                i -> [w587]
                                n2176 = Increment(x=w584) -> (x+1=w585:i32)
                                n2177 = Increment(x=w589) -> (x+1=w588:i32)
                                n2178 = Increment(x=w587) -> (x+1=w605:i32)
                                n2179 = String Subset(string=w597, offset (0)=w587, length (rest)=1 ("length (rest)")) -> (substring=w593:string)
                                n2180 = Multiply(x=3, y=w605) -> (x*y=w599:i32)
                                n2181 = Equal?(x=w593, y="1") -> (x = y?=w591:bool)
                                n2182 = Decrement(x=w599) -> (x-1=w598:i32)
                                n2183 = Select(t=w588, s=w591, f=w589) -> (s? t:f=w590:i32)
                                n2184 = Index Array(array=w606, index=w598) -> (element=w603:string)
                                n2185 = Decimal String To Number(string=w603, offset=0) -> (number=w601:i32)  [unwired: 1 in, 1 out]
                                n2186 = Equal?(x=w601, y=1) -> (x = y?=w594:bool)
                                n2187 = And(x=w594, y=w591) -> (x .and. y?=w595:bool)
                                n2188 = Select(t=w585, s=w595, f=w584) -> (s? t:f=w586:i32)
                                }
                                n2189 = case shown="True" w572 {
                                frame False {
                                }
                                frame True {
                                n2190 = One Button Dialog(message="Warning:\nH1 Parallelism Mismatch!\nEither allow this from the system configuration tab\nor change the parallelism on H2. This message will\ncontinue until the problem is corrected.") -> ()  [unwired: 1 in, 1 out]
                                }
                                }
                                n2191 = local read "H1 Device Count"() -> (w564:u32)
                                n2192 = local read "H1 Good Units"() -> (w565:u32)
                                n2193 = Add(x=w565, y=w556) -> (x+y=w566:u32)
                                n2194 = Add(x=w564, y=w555) -> (x+y=w563:u32)
                                n2195 = local write "H1 Good Units"(w566) -> ()
                                n2196 = local write "H1 Device Count"(w563) -> ()
                                }
                                frame #4 {
                                n2197 = local read "H1 Device Count"() -> (w612:u32)
                                n2198 = Divide(x=w608, y=w607) -> (x/y=w609:dbl)
                                n2199 = local read "H1 Good Units"() -> (w613:u32)
                                n2200 = Multiply(x=w609, y=100.0) -> (x*y=w611:dbl)
                                n2201 = Divide(x=w613, y=w612) -> (x/y=w616:dbl)
                                n2202 = local write "H1 cycle yield hid"(w611) -> ()
                                n2203 = Multiply(x=w616, y=100.0) -> (x*y=w614:dbl)
                                n2204 = local write "H1 lot yield mon"(w614) -> ()
                                }
                                frame #5 {
                                n2205 = local read "H1 online"() -> (w617:bool)
                                n2206 = local read "POWER"() -> (w618:bool)
                                n2207 = Compound Arithmetic op=AND(w617, w618) -> (w619:bool)
                                n2208 = case shown="True" w619 {
                                frame False {
                                n2209 = local write "MT99XX tester states H1 hid"(SC_MT99XX_tester_states."closing bus" ("SC virtual tester states")) -> ()
                                }
                                frame True {
                                n2210 = local write "MT99XX tester states H1 hid"(SC_MT99XX_tester_states."polling *SITES?" ("SC virtual tester states")) -> ()
                                }
                                }
                                }
                                }
                                }
                                frame "closing bus" {
                                n2211 = local read "GPIB bus 1 traffic"() -> (w626:string)
                                n2212 = local write "Exit SC tester H1 StMach hid"(TRUE ("Exit H1 state machine hid")) -> ()
                                n2213 = local read "VISA bus 1 resource name out hid"() -> (w630:refnum<visa-resource-name>)
                                n2214 = local read "VISA bus 1 error out hid"() -> (w629:errorcluster)
                                n2215 = Concatenate Strings(w626, "\r\n", "Bus 1: closing " ("string")) -> (w624:string)
                                n2216 = local write "GPIB bus 1 traffic"(w624) -> ()
                                n2217 = VISA Close(VISA resource name=w630, error in (no error)=w629) -> (error out=w628:errorcluster)
                                n2218 = Unbundle By Name(w628) -> ("status"=w627:bool)
                                n2219 = local write "VISA bus 1 close error"(w627) -> ()
                                }
                              }
                            }
                            frame #1 {
                              n2220 = local read "Slow for  Diagnostics"() -> (w631:bool)
                              n2221 = case shown="False" w631 {
                                frame False {
                                }
                                frame True {
                                n2222 = local read "GPIB wait time (ms)"() -> (w632:u32)
                                n2223 = Wait (ms)(milliseconds to wait=w632) -> ()  [unwired: 1 out]
                                }
                              }
                            }
                          }
                        }
                        frame "Seiko-Epson NS6040" {
                          n2224 = local write "NS6040 tester states H1 hid"(SC_NS6040_tester_states_v2."initializing bus" ("NS6040 tester states H1 hid")) -> ()
                          n2225 = while {
                            stop <- w635 stop-if-true
                            n2226 = Wait (ms)(milliseconds to wait=u32 5) -> ()  [unwired: 1 out]
                            n2227 = flat-sequence {
                              frame #0 {
                                n2228 = local read "NS6040 tester states H1 hid"() -> (w636:T4)
                                n2229 = case shown="\"sending Fullsites?\"" w636 {
                                frame "initializing bus", Default {
                                n2230 = flat-sequence {
                                frame #0 {
                                # "bus 1"
                                n2231 = local read "GPIB wait timeout hid"() -> (w640:u32)
                                n2232 = local read "SentCtrl talks to handler 1 at"() -> (w641:refnum<visa-resource-name>)
                                n2233 = local read "GPIB wait timeout hid"() -> (w639:u32)
                                n2234 = VISA Open(timeout (0)=w640, VISA resource name=w641) -> (VISA resource name=w638:refnum<visa-resource-name>, error out=w643:errorcluster)  [unwired: 3 in]
                                n2235 = property class="GPIB Instr"(reference=w638, error in=w643, "Timeout"=w639) -> (error out=w637:errorcluster)  [unwired: 1 out]
                                n2236 = local write "VISA bus 1 resource name out hid"(w638) -> ()
                                n2237 = Unbundle By Name(w637) -> ("status"=w642:bool)
                                n2238 = local write "VISA bus 1 open error"(w642) -> ()
                                n2239 = local write "VISA bus 1 error out hid"(w637) -> ()
                                }
                                frame #1 {
                                n2240 = local read "VISA bus 1 resource name out hid"() -> (w646:refnum<visa-resource-name>)
                                n2241 = local read "VISA bus 1 error out hid"() -> (w645:errorcluster)
                                n2242 = VISA Clear(VISA resource name=w646, error in (no error)=w645) -> (error out=w644:errorcluster)  [unwired: 1 out]
                                n2243 = local write "VISA bus 1 error out hid"(w644) -> ()
                                }
                                frame #2 {
                                n2244 = local write "Exit SC tester H1 StMach hid"(FALSE ("Exit H1 state machine hid")) -> ()
                                n2245 = Concatenate Strings("Bus 1 initializing" ("string"), "\r\n") -> (w649:string)
                                n2246 = local write "GPIB bus 1 traffic"(w649) -> ()
                                }
                                frame #3 {
                                n2247 = local write "NS6040 tester states H1 hid"(SC_NS6040_tester_states_v2."serial polling handler" ("NS6040 tester states H1 hid")) -> ()
                                }
                                }
                                }
                                frame "sending *IDN?" {
                                n2248 = flat-sequence {
                                tunnel: [w661] -> w654
                                tunnel: [w660] -> w653
                                tunnel: w654 -> [w675]
                                tunnel: w653 -> [w674]
                                tunnel: [w665] -> w652
                                tunnel: w652 -> [w676]
                                frame #0 {
                                w655 = "*IDN?\n"
                                # "It was discovered that his state is not initialized in application"
                                n2249 = local read "VISA bus 1 resource name out hid"() -> (w664:refnum<visa-resource-name>)
                                n2250 = local read "GPIB bus 1 traffic"() -> (w659:string)
                                n2251 = local read "VISA bus 1 error out hid"() -> (w663:errorcluster)
                                n2252 = Concatenate Strings(w659, "\r\n", "Bus 1 write: " ("string"), w655) -> (w657:string)
                                n2253 = VISA Write(VISA resource name=w664, write buffer=w655, error in (no error)=w663) -> (VISA resource name out=w661:refnum<visa-resource-name>, error out=w660:errorcluster)  [unwired: 1 out]
                                n2254 = Unbundle By Name(w660) -> ("status"=w662:bool)
                                n2255 = local write "GPIB bus 1 traffic"(w657) -> ()
                                n2256 = local write "GPIB bus 1 write error"(w662) -> ()
                                }
                                frame #1 {
                                n2257 = local read "GPIB bus 1 traffic"() -> (w667:string)
                                n2258 = VISA Read(VISA resource name=w675, byte count=u32 128, error in (no error)=w674) -> (VISA resource name out=w672:refnum<visa-resource-name>, read buffer=w666:string, error out=w671:errorcluster)  [unwired: 1 out]
                                n2259 = local write "VISA bus 1 resource name out hid"(w672) -> ()
                                n2260 = Unbundle By Name(w671) -> ("status"=w665:bool)
                                n2261 = local write "H1 response to *IDN? hid"(w666) -> ()
                                n2262 = local write "GPIB bus 1 read error"(w665) -> ()
                                n2263 = Concatenate Strings(w667, "\r\n", "Bus 1 read: " ("string"), w666) -> (w669:string)
                                n2264 = local write "GPIB bus 1 traffic"(w669) -> ()
                                }
                                frame #2 {
                                n2265 = case shown="True" w676 {
                                frame False {
                                n2266 = local write "NS6040 tester states H1 hid"(SC_NS6040_tester_states_v2."serial polling handler" ("NS6040 tester states H1 hid")) -> ()
                                }
                                frame True {
                                n2267 = flat-sequence {
                                frame #0 {
                                n2268 = while {
                                stop <- w679 stop-if-true
                                n2269 = One Button Dialog(message="Warning:\nVirtual tester does not get a response\nto *IDN? from handler 1.\nCheck GPIB cable and that  handler 1 \nis running and ready to issue a start of test\nby responding with sites ready.", button name ("OK")="Dismiss and retry") -> (true=w679:bool)
                                n2270 = Wait (ms)(milliseconds to wait=u32 100) -> ()  [unwired: 1 out]
                                }
                                }
                                frame #1 {
                                n2271 = local write "H1 online"(FALSE ("H1 online")) -> ()
                                }
                                frame #2 {
                                n2272 = local write "NS6040 tester states H1 hid"(SC_NS6040_tester_states_v2."sending *IDN?" ("NS6040 tester states H1 hid")) -> ()
                                }
                                }
                                }
                                }
                                }
                                }
                                }
                                frame "serial polling handler" {
                                n2273 = flat-sequence {
                                frame #0 {
                                n2274 = Concatenate Strings("Bus 1 read: " ("string"), "Serial polling handler 1") -> (w685:string)
                                n2275 = local write "GPIB bus 1 traffic"(w685) -> ()
                                }
                                frame #1 {
                                n2276 = local read "VISA bus 1 resource name out hid"() -> (w692:refnum<visa-resource-name>)
                                n2277 = local read "VISA bus 1 error out hid"() -> (w691:errorcluster)
                                n2278 = VISA Read STB(8:w691, 11:w692) -> (0:w693:errorcluster, 2:w689:u16)  [unwired: 1 out]
                                n2279 = Unbundle By Name(w693) -> ("status"=w690:bool)
                                n2280 = Equal?(x=w689, y=u16 65) -> (x = y?=w687:bool)
                                n2281 = case shown="True" w687 {
                                frame False {
                                n2282 = flat-sequence {
                                frame #0 {
                                n2283 = Wait (ms)(milliseconds to wait=u32 5) -> ()  [unwired: 1 out]
                                }
                                frame #1 {
                                n2284 = local write "NS6040 tester states H1 hid"(SC_NS6040_tester_states_v2."serial polling handler" ("NS6040 tester states H1 hid")) -> ()
                                }
                                }
                                }
                                frame True {
                                n2285 = flat-sequence {
                                frame #0 {
                                n2286 = local write "H1 Waiting"(TRUE ("H1 Ready with sites")) -> ()
                                n2287 = local write "H1 Indexing"(FALSE ("h1 indexing")) -> ()
                                n2288 = local write "H1 Testing"(FALSE ("h1 indexing")) -> ()
                                n2289 = local write "H1 Ready with sites hid"(TRUE ("H1 Ready with sites hid")) -> ()
                                }
                                frame #1 {
                                n2290 = Tick Count (ms)() -> (millisecond timer value=w700:u32)
                                n2291 = Tick Count (ms)() -> (millisecond timer value=w701:u32)
                                n2292 = local write "H1 wt start hidden"(w700) -> ()
                                n2293 = local write "H1 it end hidden"(w701) -> ()
                                }
                                frame #2 {
                                n2294 = local read "H1 it start hidden"() -> (w705:u32)
                                n2295 = local read "H1 it end hidden"() -> (w706:u32)
                                n2296 = Subtract(x=w706, y=w705) -> (x-y=w702:u32)
                                n2297 = Divide(x=w702, y=u32 1000) -> (x/y=w704:dbl)
                                n2298 = local write "H1 measured Index Time"(w704) -> ()
                                }
                                frame #3 {
                                n2299 = local write "NS6040 tester states H1 hid"(SC_NS6040_tester_states_v2."sending Fullsites?" ("NS6040 tester states H1 hid")) -> ()
                                }
                                }
                                }
                                }
                                n2300 = local write "GPIB bus 1 write error"(w690) -> ()
                                }
                                }
                                }
                                frame "sending Fullsites?" {
                                n2301 = flat-sequence {
                                tunnel: [w719] -> w711
                                tunnel: [w718] -> w710
                                tunnel: [w723] -> w709
                                tunnel: w710 -> [w724]
                                tunnel: w711 -> [w725]
                                tunnel: w709 -> [w741]
                                tunnel: [w741] -> w708
                                tunnel: w708 -> [w742]
                                frame #0 {
                                w717 = "Fullsites?\n"
                                n2302 = local read "VISA bus 1 resource name out hid"() -> (w721:refnum<visa-resource-name>)
                                n2303 = local read "VISA bus 1 error out hid"() -> (w720:errorcluster)
                                n2304 = local read "GPIB bus 1 traffic"() -> (w713:string)
                                n2305 = call <vilib>:"Trim Whitespace.vi"("string"=w717) -> ("trimmed string"=w712:string)  [unwired: 1 in]
                                n2306 = VISA Write(VISA resource name=w721, write buffer=w717, error in (no error)=w720) -> (VISA resource name out=w718:refnum<visa-resource-name>, error out=w719:errorcluster)  [unwired: 1 out]
                                n2307 = Unbundle By Name(w719) -> ("status"=w722:bool)
                                n2308 = Concatenate Strings(w713, "\r\n", "Bus 1 write: " ("string"), w712) -> (w716:string)
                                n2309 = local write "GPIB bus 1 write error"(w722) -> ()
                                n2310 = local write "GPIB bus 1 traffic"(w716) -> ()
                                }
                                frame #1 {
                                n2311 = while {
                                tunnel: w725 -> [w734]
                                tunnel: w724 -> [w733]
                                tunnel: [w728] -> w723
                                stop <- w727 stop-if-true
                                n2312 = local read "GPIB bus 1 traffic"() -> (w739:string)
                                n2313 = VISA Read(VISA resource name=w733, byte count=u32 128, error in (no error)=w734) -> (read buffer=w728:string, error out=w731:errorcluster)  [unwired: 2 out]
                                n2314 = Unbundle By Name(w731) -> ("status"=w740:bool)
                                n2315 = call <vilib>:"Trim Whitespace.vi"("string"=w728) -> ("trimmed string"=w732:string)  [unwired: 1 in]
                                n2316 = Match True/False String(2:"X" ("false string"), 3:"Fullsites" ("true string"), 4:w728) -> (0:w727:bool)  [unwired: 1 out]
                                n2317 = local write "GPIB bus 1 read error"(w740) -> ()
                                n2318 = Concatenate Strings(w739, "\r\n", "Bus 1 read: " ("string"), w732) -> (w737:string)
                                n2319 = local write "GPIB bus 1 traffic"(w737) -> ()
                                n2320 = Wait (ms)(milliseconds to wait=u32 5) -> ()  [unwired: 1 out]
                                }
                                }
                                frame #2 {
                                n2321 = local write "H1 FULLSITES? response hid"(w741) -> ()
                                }
                                frame #3 {
                                w744 = "%032b"  # format string
                                n2322 = call <vilib>:"Space Constant.vi"() -> ("String"=w749:string)
                                n2323 = Concatenate Strings("Fullsites" ("regular expression"), w749) -> (w750:string)
                                n2324 = Match Pattern(string=w742, regular expression=w750) -> (after substring=w746:string)  [unwired: 1 in, 3 out]
                                n2325 = Hexadecimal String To Number(string=w746, default (0uL)=u64 0 ("default (0 U32)")) -> (number=w743:u64)  [unwired: 1 in, 1 out]
                                n2326 = Format Into String "Format Into String"(format string=w744, w743) -> (resulting string=w747:string)  [unwired: 2 in, 1 out]
                                n2327 = local write "H1 FULLSITES? binary hid"(w747) -> ()
                                }
                                frame #4 {
                                n2328 = while {
                                i -> [w751]
                                stop <- w752 stop-if-true
                                n2329 = Wait (ms)(milliseconds to wait=u32 1) -> ()  [unwired: 1 out]
                                n2330 = local read "H1 Lock"() -> (w752:bool)
                                "Numeric 2" <- w751
                                }
                                }
                                frame #5 {
                                n2331 = local write "NS6040 tester states H1 hid"(SC_NS6040_tester_states_v2."testing" ("NS6040 tester states H1 hid")) -> ()
                                n2332 = local write "SC handler states hid"(SC_handler_states."testing" ("SC Test Interface States")) -> ()
                                }
                                }
                                }
                                frame "testing" {
                                n2333 = flat-sequence {
                                frame #0 {
                                n2334 = local read "GPIB bus 1 traffic"() -> (w759:string)
                                n2335 = Concatenate Strings(w759, "\r\n", "Bus 1: " ("string"), "testing" ("string")) -> (w757:string)
                                n2336 = local write "GPIB bus 1 traffic"(w757) -> ()
                                }
                                frame #1 {
                                n2337 = Tick Count (ms)() -> (millisecond timer value=w764:u32)
                                n2338 = Tick Count (ms)() -> (millisecond timer value=w765:u32)
                                n2339 = local write "H1 Indexing"(FALSE ("waiting")) -> ()
                                n2340 = local write "H1 Testing"(TRUE ("testing")) -> ()
                                n2341 = local write "H1 tt start hidden"(w764) -> ()
                                n2342 = local write "H1 wt end hidden"(w765) -> ()
                                n2343 = local write "H1 Waiting"(TRUE ("H1 Ready with sites")) -> ()
                                }
                                frame #2 {
                                n2344 = local read "H1 wt start hidden"() -> (w769:u32)
                                n2345 = local read "H1 wt end hidden"() -> (w770:u32)
                                n2346 = Subtract(x=w770, y=w769) -> (x-y=w768:u32)
                                n2347 = Divide(x=w768, y=u32 1000) -> (x/y=w766:dbl)
                                n2348 = local write "H1 measured Wait Time"(w766) -> ()
                                }
                                frame #3 {
                                n2349 = while {
                                stop <- w772 continue-if-true
                                n2350 = local read "H1 Lock"() -> (w772:bool)
                                n2351 = Wait (ms)(milliseconds to wait=u32 1) -> ()  [unwired: 1 out]
                                }
                                }
                                frame #4 {
                                n2352 = local write "H1 Ready with sites hid"(FALSE ("H1 Ready with siutes hid")) -> ()
                                n2353 = local write "NS6040 tester states H1 hid"(SC_NS6040_tester_states_v2."binning" ("NS6040 tester states H1 hid")) -> ()
                                }
                                }
                                }
                                frame "binning" {
                                n2354 = flat-sequence {
                                frame #0 {
                                n2355 = Tick Count (ms)() -> (millisecond timer value=w776:u32)
                                n2356 = Tick Count (ms)() -> (millisecond timer value=w775:u32)
                                n2357 = local write "H1 it start hidden"(w776) -> ()
                                n2358 = local write "H1 tt end hidden"(w775) -> ()
                                }
                                frame #1 {
                                n2359 = local read "GPIB bus 1 traffic"() -> (w780:string)
                                n2360 = Concatenate Strings(w780, "\r\n", "Bus 1: " ("string"), "binning" ("string")) -> (w778:string)
                                n2361 = local write "GPIB bus 1 traffic"(w778) -> ()
                                }
                                frame #2 {
                                n2362 = local write "H1 Waiting"(FALSE ("H1 Ready with sites")) -> ()
                                n2363 = local write "H1 Indexing"(TRUE ("waiting")) -> ()
                                n2364 = local write "H1 Testing"(FALSE ("testing")) -> ()
                                }
                                frame #3 {
                                n2365 = local read "H1 tt start hidden"() -> (w786:u32)
                                n2366 = local read "H1 tt end hidden"() -> (w787:u32)
                                n2367 = Subtract(x=w787, y=w786) -> (x-y=w788:u32)
                                n2368 = Divide(x=w788, y=u32 1000) -> (x/y=w785:dbl)
                                n2369 = local write "H1 measured Test Time"(w785) -> ()
                                }
                                frame #4 {
                                n2370 = local read "H1 binning string hid"() -> (w796:string)
                                n2371 = local read "H1 FULLSITES? binary hid"() -> (w795:string)
                                n2372 = String Subset(string=w796, offset (0)=6, length (rest)=35 ("length (rest)")) -> (substring=w802:string)
                                n2373 = local read "H1 Device Count"() -> (w793:u32)
                                n2374 = local read "H1 Good Units"() -> (w794:u32)
                                n2375 = Search and Replace String(replace all?=TRUE ("replace all? (F)"), input string=w802, search string=",") -> (result string=w808:string)  [unwired: 5 in, 3 out]
                                n2376 = Search and Replace String(replace all?=TRUE ("replace all? (F)"), input string=w795, search string="1") -> (number of replacements=w799:i32)  [unwired: 5 in, 3 out]
                                n2377 = Add(x=w799, y=w793) -> (x+y=w791:u32)
                                n2378 = Divide(x=w794, y=w793) -> (x/y=w809:dbl)
                                n2379 = Search and Replace String(replace all?=TRUE ("replace all? (F)"), input string=w808, search string="1") -> (number of replacements=w807:i32)  [unwired: 5 in, 3 out]
                                n2380 = local write "H1 Device Count"(w791) -> ()
                                n2381 = Add(x=w807, y=w794) -> (x+y=w792:u32)
                                n2382 = Multiply(x=w809, y=100.0) -> (x*y=w790:dbl)
                                n2383 = local write "H1 Good Units"(w792) -> ()
                                n2384 = local write "H1 cycle yield hid"(w790) -> ()
                                }
                                frame #5 {
                                n2385 = local read "H1 Device Count"() -> (w812:u32)
                                n2386 = local read "H1 Good Units"() -> (w813:u32)
                                n2387 = Divide(x=w813, y=w812) -> (x/y=w814:dbl)
                                n2388 = Multiply(x=w814, y=100.0) -> (x*y=w811:dbl)
                                n2389 = local write "H1 lot yield mon"(w811) -> ()
                                }
                                frame #6 {
                                n2390 = local read "H1 online"() -> (w816:bool)
                                n2391 = local read "POWER"() -> (w817:bool)
                                n2392 = Compound Arithmetic op=AND(w816, w817) -> (w818:bool)
                                n2393 = case shown="False" w818 {
                                frame False {
                                n2394 = local write "NS6040 tester states H1 hid"(SC_NS6040_tester_states_v2."closing bus" ("NS6040 tester states H1 hid")) -> ()
                                }
                                frame True {
                                n2395 = local write "NS6040 tester states H1 hid"(SC_NS6040_tester_states_v2."serial polling handler" ("NS6040 tester states H1 hid")) -> ()
                                }
                                }
                                }
                                }
                                }
                                frame "closing bus" {
                                n2396 = local read "GPIB bus 1 traffic"() -> (w825:string)
                                n2397 = local write "Exit SC tester H1 StMach hid"(TRUE ("Exit H1 state machine hid")) -> ()
                                n2398 = local read "VISA bus 1 resource name out hid"() -> (w829:refnum<visa-resource-name>)
                                n2399 = local read "VISA bus 1 error out hid"() -> (w828:errorcluster)
                                n2400 = Concatenate Strings(w825, "\r\n", "Bus 1: closing " ("string")) -> (w823:string)
                                n2401 = local write "GPIB bus 1 traffic"(w823) -> ()
                                n2402 = VISA Close(VISA resource name=w829, error in (no error)=w828) -> (error out=w827:errorcluster)
                                n2403 = Unbundle By Name(w827) -> ("status"=w826:bool)
                                n2404 = local write "VISA bus 1 close error"(w826) -> ()
                                }
                                }
                              }
                              frame #1 {
                                n2405 = local read "Slow for  Diagnostics"() -> (w830:bool)
                                n2406 = case shown="False" w830 {
                                frame False {
                                }
                                frame True {
                                n2407 = local read "GPIB wait time (ms)"() -> (w831:u32)
                                n2408 = Wait (ms)(milliseconds to wait=w831) -> ()  [unwired: 1 out]
                                }
                                }
                              }
                            }
                            n2409 = local read "Exit SC tester H1 StMach hid"() -> (w635:bool)
                          }
                        }
                      }
                    }
                  }
                }
              }
              n2410 = local read "POWER"() -> (w360:bool)
            }
            n2411 = while {
              stop <- w1784 continue-if-true
              n2412 = local read "H2 online"() -> (w1785:bool)
              n2413 = case shown="True" w1785 {
                frame False {
                }
                frame True {
                  n2414 = flat-sequence {
                    frame #0 {
                      n2415 = local write "Exit SC tester H2 StMach hid"(FALSE ("Exit H2 state machine hid")) -> ()
                    }
                    frame #1 {
                      n2416 = local read "H2 handler type"() -> (w1787:T2)
                      n2417 = case shown="\"Seiko-Epson NS6040\"" w1787 {
                        frame "Multitest" {
                          n2418 = local write "MT99XX tester states H2 hid"(SC_MT99XX_tester_states."initializing bus" ("MT99XX tester states H2 hid")) -> ()
                          n2419 = flat-sequence {
                            frame #0 {
                              n2420 = local read "MT99XX tester states H2 hid"() -> (w1789:T5)
                              n2421 = case shown="\"binning\"" w1789 {
                                frame "initializing bus", Default {
                                n2422 = flat-sequence {
                                frame #0 {
                                # "bus 2"
                                n2423 = local read "GPIB wait timeout hid"() -> (w1792:u32)
                                n2424 = local read "SentCtrl talks to handler 2 at"() -> (w1794:refnum<visa-resource-name>)
                                n2425 = local read "GPIB wait timeout hid"() -> (w1793:u32)
                                n2426 = VISA Open(timeout (0)=w1792, VISA resource name=w1794) -> (VISA resource name=w1791:refnum<visa-resource-name>, error out=w1796:errorcluster)  [unwired: 3 in]
                                n2427 = property class="GPIB Instr"(reference=w1791, error in=w1796, "Timeout"=w1793) -> (error out=w1790:errorcluster)  [unwired: 1 out]
                                n2428 = local write "VISA bus 2 resource name out hid"(w1791) -> ()
                                n2429 = Unbundle By Name(w1790) -> ("status"=w1795:bool)
                                n2430 = local write "VISA bus 2 error out hid"(w1790) -> ()
                                n2431 = local write "VISA bus 2 open error"(w1795) -> ()
                                }
                                frame #1 {
                                n2432 = local write "Exit SC tester H2 StMach hid"(FALSE ("Exit H2 state machine hid")) -> ()
                                n2433 = Concatenate Strings("Bus 2 initializing" ("string"), "\r\n") -> (w1799:string)
                                n2434 = local write "GPIB bus 2 traffic"(w1799) -> ()
                                }
                                frame #2 {
                                n2435 = local write "MT99XX tester states H2 hid"(SC_MT99XX_tester_states."sending *IDN?" ("SC virtual tester states")) -> ()
                                }
                                }
                                }
                                frame "sending *IDN?" {
                                n2436 = flat-sequence {
                                tunnel: [w1811] -> w1804
                                tunnel: [w1810] -> w1803
                                tunnel: w1804 -> [w1825]
                                tunnel: w1803 -> [w1824]
                                tunnel: [w1815] -> w1802
                                tunnel: w1802 -> [w1826]
                                frame #0 {
                                w1805 = "*IDN?"
                                n2437 = local read "VISA bus 2 resource name out hid"() -> (w1814:refnum<visa-resource-name>)
                                n2438 = local read "GPIB bus 2 traffic"() -> (w1809:string)
                                n2439 = local read "VISA bus 2 error out hid"() -> (w1813:errorcluster)
                                n2440 = Concatenate Strings(w1809, "\r\n", "Bus 2 write: " ("string"), w1805) -> (w1807:string)
                                n2441 = VISA Write(VISA resource name=w1814, write buffer=w1805, error in (no error)=w1813) -> (VISA resource name out=w1811:refnum<visa-resource-name>, error out=w1810:errorcluster)  [unwired: 1 out]
                                n2442 = local write "GPIB bus 2 traffic"(w1807) -> ()
                                n2443 = Unbundle By Name(w1810) -> ("status"=w1812:bool)
                                n2444 = local write "GPIB bus 2 write error"(w1812) -> ()
                                }
                                frame #1 {
                                n2445 = local read "GPIB bus 2 traffic"() -> (w1817:string)
                                n2446 = VISA Read(VISA resource name=w1825, byte count=u32 128, error in (no error)=w1824) -> (VISA resource name out=w1822:refnum<visa-resource-name>, read buffer=w1816:string, error out=w1821:errorcluster)  [unwired: 1 out]
                                n2447 = local write "VISA bus 2 resource name out hid"(w1822) -> ()
                                n2448 = Unbundle By Name(w1821) -> ("status"=w1815:bool)
                                n2449 = local write "H2 response to *IDN? hid"(w1816) -> ()
                                n2450 = local write "GPIB bus 2 read error"(w1815) -> ()
                                n2451 = Concatenate Strings(w1817, "\r\n", "Bus 2 read: " ("string"), w1816) -> (w1819:string)
                                n2452 = local write "GPIB bus 2 traffic"(w1819) -> ()
                                }
                                frame #2 {
                                n2453 = case shown="False" w1826 {
                                frame False {
                                n2454 = local write "MT99XX tester states H2 hid"(SC_MT99XX_tester_states."polling *SITES?" ("SC virtual tester states")) -> ()
                                }
                                frame True {
                                n2455 = flat-sequence {
                                frame #0 {
                                n2456 = while {
                                stop <- w1829 stop-if-true
                                n2457 = One Button Dialog(message="Warning:\nVirtual tester does not get a response\nto *IDN? from handler 2.\nCheck GPIB cable and that  handler 2 \nis running and ready to issue a start of test\nby responding with sites ready.", button name ("OK")="Dismiss and retry") -> (true=w1829:bool)
                                n2458 = Wait (ms)(milliseconds to wait=u32 100) -> ()  [unwired: 1 out]
                                }
                                }
                                frame #1 {
                                n2459 = local write "H2 online"(FALSE ("H2 online")) -> ()
                                }
                                frame #2 {
                                n2460 = local write "MT99XX tester states H2 hid"(SC_MT99XX_tester_states."sending *IDN?" ("SC virtual tester states")) -> ()
                                }
                                }
                                }
                                }
                                }
                                }
                                }
                                frame "polling *SITES?" {
                                n2461 = flat-sequence {
                                tunnel: [w1837] -> w1835
                                tunnel: [w1836] -> w1834
                                tunnel: w1835 -> [w1873]
                                tunnel: w1834 -> [w1872]
                                frame #0 {
                                n2462 = while {
                                tunnel: [w1841] -> w1837
                                tunnel: [w1838] -> w1836
                                stop <- w1840 stop-if-true
                                n2463 = stacked-sequence {
                                tunnel: [w1853] -> w1843
                                tunnel: [w1852] -> w1842
                                frame #0 {
                                w1848 = "*SITES?"
                                n2464 = local read "VISA bus 2 resource name out hid"() -> (w1845:refnum<visa-resource-name>)
                                n2465 = local read "VISA bus 2 error out hid"() -> (w1844:errorcluster)
                                n2466 = Concatenate Strings("Handler 2 cycle start" ("string"), "\r\n", "Bus 2 write: " ("string"), w1848) -> (w1850:string)
                                n2467 = VISA Write(VISA resource name=w1845, write buffer=w1848, error in (no error)=w1844) -> (VISA resource name out=w1853:refnum<visa-resource-name>, error out=w1852:errorcluster)  [unwired: 1 out]
                                n2468 = Unbundle By Name(w1852) -> ("status"=w1846:bool)
                                n2469 = local write "GPIB bus 2 traffic"(w1850) -> ()
                                n2470 = local write "GPIB bus 2 write error"(w1846) -> ()
                                }
                                }
                                n2471 = Wait (ms)(milliseconds to wait=u32 1) -> ()  [unwired: 1 out]
                                n2472 = flat-sequence {
                                tunnel: w1843 -> [w1871]
                                tunnel: w1842 -> [w1870]
                                tunnel: [w1857] -> w1841
                                tunnel: [w1855] -> w1840
                                tunnel: [w1854] -> w1838
                                frame #0 {
                                n2473 = local read "GPIB bus 2 traffic"() -> (w1862:string)
                                n2474 = VISA Read(VISA resource name=w1871, byte count=u32 128, error in (no error)=w1870) -> (read buffer=w1857:string, error out=w1868:errorcluster)  [unwired: 2 out]
                                n2475 = Unbundle By Name(w1868) -> ("status"=w1854:bool)
                                n2476 = String Length(string=w1857) -> (length=w1859:i32)
                                n2477 = Scan Value(string=w1857, format string="%b", default (0 dbl)=u8 0) -> (value=w1861:u8)  [unwired: 1 out]
                                n2478 = Concatenate Strings(w1862, "\r\n", "Bus 2 read: " ("string"), w1857) -> (w1864:string)
                                n2479 = local write "GPIB bus 2 read error"(w1854) -> ()
                                n2480 = Greater Than 0?(x=w1859) -> (x > 0?=w1858:bool)
                                n2481 = Greater Than 0?(x=w1861) -> (x > 0?=w1860:bool)
                                n2482 = local write "GPIB bus 2 traffic"(w1864) -> ()
                                n2483 = And(x=w1858, y=w1860) -> (x .and. y?=w1856:bool)
                                n2484 = Or(x=w1856, y=w1854) -> (x .or. y?=w1855:bool)
                                }
                                }
                                }
                                }
                                frame #1 {
                                n2485 = case shown="False" w1872 {
                                tunnel: w1873 -> [w1874 _]
                                frame False {
                                n2486 = flat-sequence {
                                tunnel: w1874 -> [w1875]
                                frame #0 {
                                n2487 = local write "H2 SITES? response hid"(w1875) -> ()
                                n2488 = String Length(string=w1875) -> (length=w1876:i32)
                                n2489 = local write "H2 parallelism"(w1876) -> ()
                                }
                                frame #1 {
                                # "This block adds zeroes (sites not ready)\nto SITES READY from handlers when the\nhandler is running at a lower parallelism\nthan the test program, but has the same\npin mapping for the active sites in common."
                                n2490 = local read "Program Parallelism"() -> (w1878:u32)
                                n2491 = local read "H2 allow lower parallelism"() -> (w1879:bool)
                                n2492 = local read "H2 parallelism"() -> (w1877:u32)
                                n2493 = Less?(x=w1877, y=w1878) -> (x < y?=w1880:bool)
                                n2494 = And(x=w1880, y=w1879) -> (x .and. y?=w1881:bool)
                                n2495 = case shown="False" w1881 {
                                frame False {
                                n2496 = local read "Program Parallelism"() -> (w1884:u32)
                                n2497 = local read "H2 parallelism"() -> (w1882:u32)
                                n2498 = Greater?(x=w1882, y=w1884) -> (0:w1883:bool)
                                n2499 = case shown="True" w1883 {
                                frame False {
                                # "parallelisms must match if arriving here"
                                n2500 = local write "MT99XX tester states H2 hid"(SC_MT99XX_tester_states."testing" ("SC virtual tester states")) -> ()
                                }
                                frame True {
                                n2501 = local write "POWER"(FALSE ("POWER")) -> ()
                                n2502 = local write "MT99XX tester states H2 hid"(SC_MT99XX_tester_states."closing bus" ("SC virtual tester states")) -> ()
                                n2503 = One Button Dialog(message="Fatal error 301:\nTest program cannot support higher\nparallelism on handler 2.\nThe Sentinel Controller program is shutting down.\nPlease correct the mismatch and restart.") -> ()  [unwired: 1 in, 1 out]
                                }
                                }
                                }
                                frame True {
                                n2504 = local read "Program Parallelism"() -> (w1894:u32)
                                n2505 = local read "H2 parallelism"() -> (w1892:u32)
                                n2506 = local read "H2 SITES? response hid"() -> (w1890:string)
                                n2507 = local write "MT99XX tester states H2 hid"(SC_MT99XX_tester_states."testing" ("SC virtual tester states")) -> ()
                                n2508 = Subtract(x=w1894, y=w1892) -> (x-y=w1893:u32)
                                n2509 = for {
                                N: w1893 -> [_]
                                shift-right: [w1895] -> w1889
                                shift-left: w1890 -> [w1896]
                                n2510 = Concatenate Strings(w1896, "0" ("string")) -> (w1895:string)
                                }
                                n2511 = local write "H2 SITES? response hid"(w1889) -> ()
                                }
                                }
                                }
                                frame #2 {
                                n2512 = Tick Count (ms)() -> (millisecond timer value=w1902:u32)
                                n2513 = Tick Count (ms)() -> (millisecond timer value=w1901:u32)
                                n2514 = local write "H2 Indexing"(FALSE ("h1 indexing")) -> ()
                                n2515 = local write "H2 Testing"(FALSE ("h1 indexing")) -> ()
                                n2516 = local write "H2 wt start hidden"(w1902) -> ()
                                n2517 = local write "H2 it end hidden"(w1901) -> ()
                                n2518 = local write "H2 Waiting"(TRUE ("H2 Waiting")) -> ()
                                }
                                frame #3 {
                                n2519 = local read "H2 it start hidden"() -> (w1906:u32)
                                n2520 = local read "H2 it end hidden"() -> (w1907:u32)
                                n2521 = Subtract(x=w1907, y=w1906) -> (x-y=w1903:u32)
                                n2522 = local write "MT99XX tester states H2 hid"(SC_MT99XX_tester_states."testing" ("SC virtual tester states")) -> ()
                                n2523 = Divide(x=w1903, y=u32 1000) -> (x/y=w1905:dbl)
                                n2524 = local write "H2 measured  Index Time"(w1905) -> ()
                                }
                                }
                                }
                                frame True {
                                n2525 = flat-sequence {
                                frame #0 {
                                n2526 = local read "VISA bus 2 resource name out hid"() -> (w1912:refnum<visa-resource-name>)
                                n2527 = local read "VISA bus 2 error out hid"() -> (w1911:errorcluster)
                                n2528 = VISA Close(VISA resource name=w1912, error in (no error)=w1911) -> (error out=w1910:errorcluster)
                                n2529 = Unbundle By Name(w1910) -> ("status"=w1909:bool)
                                n2530 = local write "VISA bus 2 close error"(w1909) -> ()
                                }
                                frame #1 {
                                n2531 = local write "VISA bus 2 close error"(FALSE ("VISA bus 1 close error")) -> ()
                                n2532 = Concatenate Strings("Bus 2 error  while reading,\nclosing Bus 2 and re-initializing" ("string"), "\r\n") -> (w1914:string)
                                n2533 = local write "GPIB bus 2 traffic"(w1914) -> ()
                                }
                                frame #2 {
                                n2534 = local write "MT99XX tester states H2 hid"(SC_MT99XX_tester_states."initializing bus" ("SC virtual tester states")) -> ()
                                }
                                }
                                }
                                }
                                }
                                }
                                }
                                frame "testing" {
                                n2535 = flat-sequence {
                                frame #0 {
                                n2536 = while {
                                stop <- w1918 stop-if-true
                                n2537 = local read "H2 Lock"() -> (w1918:bool)
                                n2538 = Wait (ms)(milliseconds to wait=u32 1) -> ()  [unwired: 1 out]
                                }
                                }
                                frame #1 {
                                n2539 = Tick Count (ms)() -> (millisecond timer value=w1930:u32)
                                n2540 = Tick Count (ms)() -> (millisecond timer value=w1929:u32)
                                n2541 = local write "H2 Indexing"(FALSE ("waiting")) -> ()
                                n2542 = local write "H2 Testing"(TRUE ("testing")) -> ()
                                n2543 = local write "H2 Waiting"(FALSE ("waiting")) -> ()
                                n2544 = local write "H2 wt end hidden"(w1930) -> ()
                                n2545 = local write "H2 tt start hidden"(w1929) -> ()
                                n2546 = local read "GPIB bus 2 traffic"() -> (w1921:string)
                                n2547 = local write "MT99XX tester states H2 hid"(SC_MT99XX_tester_states."binning" ("SC virtual tester states")) -> ()
                                n2548 = Concatenate Strings(w1921, "\r\n", "Bus 2: " ("string"), "testing" ("string")) -> (w1923:string)
                                n2549 = local write "GPIB bus 2 traffic"(w1923) -> ()
                                }
                                frame #2 {
                                n2550 = local read "H2 wt start hidden"() -> (w1932:u32)
                                n2551 = local read "H2 wt end hidden"() -> (w1931:u32)
                                n2552 = Subtract(x=w1931, y=w1932) -> (x-y=w1935:u32)
                                n2553 = Divide(x=w1935, y=u32 1000) -> (x/y=w1933:dbl)
                                n2554 = local write "H2 measured Wait Time"(w1933) -> ()
                                }
                                frame #3 {
                                n2555 = local write "MT99XX tester states H2 hid"(SC_MT99XX_tester_states."binning" ("MT99XX tester states H2 hid")) -> ()
                                }
                                }
                                }
                                frame "binning" {
                                n2556 = flat-sequence {
                                tunnel: [w1948] -> w1939
                                tunnel: [w1975] -> w1940
                                tunnel: w1939 -> [w1975]
                                tunnel: w1940 -> [w1982]
                                tunnel: [w1981] -> w1938
                                tunnel: [w1980] -> w1937
                                tunnel: w1938 -> [w2033]
                                tunnel: w1937 -> [w2032]
                                frame #0 {
                                n2557 = while {
                                stop <- w1942 continue-if-true
                                n2558 = local read "H2 Lock"() -> (w1942:bool)
                                n2559 = Wait (ms)(milliseconds to wait=u32 1) -> ()  [unwired: 1 out]
                                }
                                }
                                frame #1 {
                                n2560 = local read "Program Parallelism"() -> (w1945:u32)
                                n2561 = local read "H2 parallelism"() -> (w1944:u32)
                                n2562 = local read "H2 allow lower parallelism"() -> (w1946:bool)
                                n2563 = Less?(x=w1944, y=w1945) -> (x < y?=w1947:bool)
                                n2564 = And(x=w1947, y=w1946) -> (x .and. y?=w1943:bool)
                                n2565 = case shown="True" w1943 {
                                tunnel: [w1949 w1960] -> w1948
                                frame False {
                                n2566 = local read "VISA bus 2 resource name out hid"() -> (w1957:refnum<visa-resource-name>)
                                n2567 = local read "Binning string from tester hid"() -> (w1949:string)
                                n2568 = local read "VISA bus 2 error out hid"() -> (w1958:errorcluster)
                                n2569 = local read "GPIB bus 2 traffic"() -> (w1953:string)
                                n2570 = VISA Write(VISA resource name=w1957, write buffer=w1949, error in (no error)=w1958) -> (VISA resource name out=w1955:refnum<visa-resource-name>, error out=w1956:errorcluster)  [unwired: 1 out]
                                n2571 = local write "VISA bus 2 resource name out hid"(w1955) -> ()
                                n2572 = local write "VISA bus 2 error out hid"(w1956) -> ()
                                n2573 = Unbundle By Name(w1956) -> ("status"=w1954:bool)
                                n2574 = Concatenate Strings(w1953, "\r\n", "Bus 2 write: " ("string"), w1949) -> (w1951:string)
                                n2575 = local write "GPIB bus 2 write error"(w1954) -> ()
                                n2576 = local write "GPIB bus 2 traffic"(w1951) -> ()
                                }
                                frame True {
                                n2577 = local read "H2 parallelism"() -> (w1959:u32)
                                n2578 = local read "Binning string from tester hid"() -> (w1961:string)
                                n2579 = local read "VISA bus 2 resource name out hid"() -> (w1972:refnum<visa-resource-name>)
                                n2580 = Multiply(x=w1959, y=u32 8) -> (x*y=w1963:u32)
                                n2581 = local read "VISA bus 2 error out hid"() -> (w1973:errorcluster)
                                n2582 = local read "GPIB bus 2 traffic"() -> (w1968:string)
                                n2583 = Decrement(x=w1963) -> (x-1=w1964:u32)
                                n2584 = String Subset(string=w1961, length (rest)=w1964) -> (substring=w1960:string)  [unwired: 1 in]
                                n2585 = VISA Write(VISA resource name=w1972, write buffer=w1960, error in (no error)=w1973) -> (VISA resource name out=w1970:refnum<visa-resource-name>, error out=w1971:errorcluster)  [unwired: 1 out]
                                n2586 = local write "VISA bus 2 resource name out hid"(w1970) -> ()
                                n2587 = local write "VISA bus 2 error out hid"(w1971) -> ()
                                n2588 = Unbundle By Name(w1971) -> ("status"=w1969:bool)
                                n2589 = Concatenate Strings(w1968, "\r\n", "Bus 2 write: " ("string"), w1960) -> (w1966:string)
                                n2590 = local write "GPIB bus 2 traffic"(w1966) -> ()
                                n2591 = local write "GPIB bus 2 write error"(w1969) -> ()
                                }
                                }
                                }
                                frame #2 {
                                n2592 = Tick Count (ms)() -> (millisecond timer value=w1977:u32)
                                n2593 = Tick Count (ms)() -> (millisecond timer value=w1976:u32)
                                n2594 = local write "H2 Testing"(FALSE ("waiting")) -> ()
                                n2595 = local write "H2 Indexing"(TRUE ("waiting")) -> ()
                                n2596 = local write "H2 it start hidden"(w1977) -> ()
                                n2597 = local write "H2 tt end hidden"(w1976) -> ()
                                n2598 = local write "H2 Waiting"(FALSE ("waiting")) -> ()
                                }
                                frame #3 {
                                n2599 = while {
                                tunnel: [w2005] -> w2001 mode=indexing
                                shift-right: [w2006] -> _
                                shift-left: w1982 -> [w2008]
                                stop <- w2003 stop-if-true
                                n2600 = Match Pattern(string=w2008, regular expression=" ") -> (before substring=w2005:string, after substring=w2006:string, offset past match=w2004:i32)  [unwired: 2 out]
                                n2601 = Less Than 0?(x=w2004) -> (x < 0?=w2003:bool)
                                }
                                n2602 = local read "H2 tt start hidden"() -> (w1986:u32)
                                n2603 = local read "H2 tt end hidden"() -> (w1987:u32)
                                n2604 = Subtract(x=w1987, y=w1986) -> (x-y=w1985:u32)
                                n2605 = Divide(x=w1985, y=u32 1000) -> (x/y=w1983:dbl)
                                n2606 = Array Size(array=w2001) -> (size(s)=w1998:i32)
                                n2607 = local read "H2 SITES? response hid"() -> (w1993:string)
                                n2608 = local read "H2 parallelism"() -> (w1992:u32)
                                n2609 = local write "H2 measured Test Time"(w1983) -> ()
                                n2610 = Divide(x=w1998, y=3) -> (x/y=w2000:dbl)
                                n2611 = To Unsigned Byte Integer(number=w2000) -> (unsigned 8bit integer=w1996:u8)
                                n2612 = Not Equal?(x=w1992, y=w1996) -> (x != y?=w1997:bool)
                                n2613 = case shown="True" w1997 {
                                frame False {
                                }
                                frame True {
                                n2614 = One Button Dialog(message="Warning:\nH2 Parallelism Mismatch!\nEither allow this from the system configuration tab\nor change the parallelism on H2. This message will\ncontinue until the problem is corrected.") -> ()  [unwired: 1 in, 1 out]
                                }
                                }
                                n2615 = for {
                                N: w1996 -> [_]
                                tunnel: w2001 -> [w2031]
                                tunnel: w1993 -> [w2022]
                                shift-right: [w2015] -> w1980
                                shift-left: 0 -> [w2014]
                                shift-right: [w2011] -> w1981
                                shift-left: 0 -> [w2009]
                                i -> [w2012]
                                n2616 = Increment(x=w2009) -> (x+1=w2010:i32)
                                n2617 = Increment(x=w2014) -> (x+1=w2013:i32)
                                n2618 = Increment(x=w2012) -> (x+1=w2030:i32)
                                n2619 = String Subset(string=w2022, offset (0)=w2012, length (rest)=1 ("length (rest)")) -> (substring=w2018:string)
                                n2620 = Multiply(x=3, y=w2030) -> (x*y=w2024:i32)
                                n2621 = Equal?(x=w2018, y="1") -> (x = y?=w2016:bool)
                                n2622 = Select(t=w2013, s=w2016, f=w2014) -> (s? t:f=w2015:i32)
                                n2623 = Decrement(x=w2024) -> (x-1=w2023:i32)
                                n2624 = Index Array(array=w2031, index=w2023) -> (element=w2028:string)
                                n2625 = Decimal String To Number(string=w2028, offset=0) -> (number=w2026:i32)  [unwired: 1 in, 1 out]
                                n2626 = Equal?(x=w2026, y=1) -> (x = y?=w2019:bool)
                                n2627 = And(x=w2019, y=w2016) -> (x .and. y?=w2020:bool)
                                n2628 = Select(t=w2010, s=w2020, f=w2009) -> (s? t:f=w2011:i32)
                                }
                                n2629 = local read "H2 Device Count"() -> (w1989:u32)
                                n2630 = local read "H2 Good Units"() -> (w1990:u32)
                                n2631 = Add(x=w1990, y=w1981) -> (x+y=w1991:u32)
                                n2632 = Add(x=w1989, y=w1980) -> (x+y=w1988:u32)
                                n2633 = local write "H2 Good Units"(w1991) -> ()
                                n2634 = local write "H2 Device Count"(w1988) -> ()
                                }
                                frame #4 {
                                n2635 = Divide(x=w2033, y=w2032) -> (x/y=w2034:dbl)
                                n2636 = local read "H2 Device Count"() -> (w2037:u32)
                                n2637 = local read "H2 Good Units"() -> (w2038:u32)
                                n2638 = Multiply(x=w2034, y=100.0) -> (x*y=w2036:dbl)
                                n2639 = local write "H2 cycle yield hid"(w2036) -> ()
                                n2640 = Divide(x=w2038, y=w2037) -> (x/y=w2041:dbl)
                                n2641 = Multiply(x=w2041, y=100.0) -> (x*y=w2039:dbl)
                                n2642 = local write "H2 lot yield mon"(w2039) -> ()
                                }
                                frame #5 {
                                n2643 = local read "H2 online"() -> (w2042:bool)
                                n2644 = local read "POWER"() -> (w2044:bool)
                                n2645 = Compound Arithmetic op=AND(w2042, w2044) -> (w2043:bool)
                                n2646 = case shown="False" w2043 {
                                frame False {
                                n2647 = local write "MT99XX tester states H2 hid"(SC_MT99XX_tester_states."closing bus" ("SC virtual tester states")) -> ()
                                }
                                frame True {
                                n2648 = local write "MT99XX tester states H2 hid"(SC_MT99XX_tester_states."polling *SITES?" ("SC virtual tester states")) -> ()
                                }
                                }
                                }
                                }
                                }
                                frame "closing bus" {
                                n2649 = local read "GPIB bus 2 traffic"() -> (w2051:string)
                                n2650 = local write "Exit SC tester H2 StMach hid"(TRUE ("Exit H2 state machine hid")) -> ()
                                n2651 = local read "VISA bus 2 resource name out hid"() -> (w2055:refnum<visa-resource-name>)
                                n2652 = local read "VISA bus 2 error out hid"() -> (w2054:errorcluster)
                                n2653 = Concatenate Strings(w2051, "\r\n", "Bus 2: closing " ("string")) -> (w2049:string)
                                n2654 = local write "GPIB bus 2 traffic"(w2049) -> ()
                                n2655 = VISA Close(VISA resource name=w2055, error in (no error)=w2054) -> (error out=w2053:errorcluster)
                                n2656 = Unbundle By Name(w2053) -> ("status"=w2052:bool)
                                n2657 = local write "VISA bus 2 close error"(w2052) -> ()
                                }
                              }
                            }
                            frame #1 {
                              n2658 = local read "Slow for  Diagnostics"() -> (w2056:bool)
                              n2659 = case shown="True" w2056 {
                                frame False {
                                }
                                frame True {
                                n2660 = local read "GPIB wait time (ms)"() -> (w2057:u32)
                                n2661 = Wait (ms)(milliseconds to wait=w2057) -> ()  [unwired: 1 out]
                                }
                              }
                            }
                          }
                        }
                        frame "Seiko-Epson NS6040" {
                          n2662 = local write "NS6040 tester states H2 hid"(SC_NS6040_tester_states_v2."initializing bus" ("NS6040 tester states H1 hid")) -> ()
                          n2663 = while {
                            stop <- w2060 stop-if-true
                            n2664 = Wait (ms)(milliseconds to wait=u32 5) -> ()  [unwired: 1 out]
                            n2665 = flat-sequence {
                              frame #0 {
                                n2666 = local read "NS6040 tester states H2 hid"() -> (w2061:T4)
                                n2667 = case shown="\"sending Fullsites?\"" w2061 {
                                frame "initializing bus", Default {
                                n2668 = flat-sequence {
                                frame #0 {
                                # "bus 2"
                                n2669 = local read "GPIB wait timeout hid"() -> (w2064:u32)
                                n2670 = local read "SentCtrl talks to handler 2 at"() -> (w2066:refnum<visa-resource-name>)
                                n2671 = local read "GPIB wait timeout hid"() -> (w2065:u32)
                                n2672 = VISA Open(timeout (0)=w2064, VISA resource name=w2066) -> (VISA resource name=w2063:refnum<visa-resource-name>, error out=w2068:errorcluster)  [unwired: 3 in]
                                n2673 = property class="GPIB Instr"(reference=w2063, error in=w2068, "Timeout"=w2065) -> (error out=w2062:errorcluster)  [unwired: 1 out]
                                n2674 = local write "VISA bus 2 resource name out hid"(w2063) -> ()
                                n2675 = Unbundle By Name(w2062) -> ("status"=w2067:bool)
                                n2676 = local write "VISA bus 2 error out hid"(w2062) -> ()
                                n2677 = local write "VISA bus 2 open error"(w2067) -> ()
                                }
                                frame #1 {
                                n2678 = local read "VISA bus 2 resource name out hid"() -> (w2071:refnum<visa-resource-name>)
                                n2679 = local read "VISA bus 2 error out hid"() -> (w2070:errorcluster)
                                n2680 = VISA Clear(VISA resource name=w2071, error in (no error)=w2070) -> (error out=w2069:errorcluster)  [unwired: 1 out]
                                n2681 = local write "VISA bus 2 error out hid"(w2069) -> ()
                                }
                                frame #2 {
                                n2682 = local write "Exit SC tester H2 StMach hid"(FALSE ("Exit H2 state machine hid")) -> ()
                                n2683 = Concatenate Strings("Bus 2 initializing" ("string"), "\r\n") -> (w2074:string)
                                n2684 = local write "GPIB bus 2 traffic"(w2074) -> ()
                                }
                                frame #3 {
                                n2685 = local write "NS6040 tester states H2 hid"(SC_NS6040_tester_states_v2."serial polling handler" ("NS6040 tester states H2 hid")) -> ()
                                }
                                }
                                }
                                frame "sending *IDN?" {
                                n2686 = flat-sequence {
                                tunnel: [w2086] -> w2079
                                tunnel: [w2085] -> w2078
                                tunnel: w2079 -> [w2100]
                                tunnel: w2078 -> [w2099]
                                tunnel: [w2090] -> w2077
                                tunnel: w2077 -> [w2101]
                                frame #0 {
                                w2080 = "*IDN?"
                                # "It was discovered that his state is not initialized in application"
                                n2687 = local read "VISA bus 2 resource name out hid"() -> (w2089:refnum<visa-resource-name>)
                                n2688 = local read "GPIB bus 2 traffic"() -> (w2084:string)
                                n2689 = local read "VISA bus 2 error out hid"() -> (w2088:errorcluster)
                                n2690 = Concatenate Strings(w2084, "\r\n", "Bus 2 write: " ("string"), w2080) -> (w2082:string)
                                n2691 = VISA Write(VISA resource name=w2089, write buffer=w2080, error in (no error)=w2088) -> (VISA resource name out=w2086:refnum<visa-resource-name>, error out=w2085:errorcluster)  [unwired: 1 out]
                                n2692 = local write "GPIB bus 2 traffic"(w2082) -> ()
                                n2693 = Unbundle By Name(w2085) -> ("status"=w2087:bool)
                                n2694 = local write "GPIB bus 2 write error"(w2087) -> ()
                                }
                                frame #1 {
                                n2695 = VISA Read(VISA resource name=w2100, byte count=u32 128, error in (no error)=w2099) -> (VISA resource name out=w2097:refnum<visa-resource-name>, read buffer=w2091:string, error out=w2096:errorcluster)  [unwired: 1 out]
                                n2696 = local read "GPIB bus 2 traffic"() -> (w2092:string)
                                n2697 = local write "VISA bus 2 resource name out hid"(w2097) -> ()
                                n2698 = Unbundle By Name(w2096) -> ("status"=w2090:bool)
                                n2699 = local write "H2 response to *IDN? hid"(w2091) -> ()
                                n2700 = local write "GPIB bus 2 read error"(w2090) -> ()
                                n2701 = Concatenate Strings(w2092, "\r\n", "Bus 2 read: " ("string"), w2091) -> (w2094:string)
                                n2702 = local write "GPIB bus 2 traffic"(w2094) -> ()
                                }
                                frame #2 {
                                n2703 = case shown="True" w2101 {
                                frame False {
                                n2704 = local write "NS6040 tester states H2 hid"(SC_NS6040_tester_states_v2."testing" ("NS6040 tester states H2 hid")) -> ()
                                }
                                frame True {
                                n2705 = flat-sequence {
                                frame #0 {
                                n2706 = while {
                                stop <- w2104 stop-if-true
                                n2707 = One Button Dialog(message="Warning:\nVirtual tester does not get a response\nto *IDN? from handler 2.\nCheck GPIB cable and that  handler 2 \nis running and ready to issue a start of test\nby responding with sites ready.", button name ("OK")="Dismiss and retry") -> (true=w2104:bool)
                                n2708 = Wait (ms)(milliseconds to wait=u32 100) -> ()  [unwired: 1 out]
                                }
                                }
                                frame #1 {
                                n2709 = local write "H2 online"(FALSE ("H2 online")) -> ()
                                }
                                frame #2 {
                                n2710 = local write "NS6040 tester states H2 hid"(SC_NS6040_tester_states_v2."serial polling handler" ("NS6040 tester states H2 hid")) -> ()
                                }
                                }
                                }
                                }
                                }
                                }
                                }
                                frame "serial polling handler" {
                                n2711 = flat-sequence {
                                frame #0 {
                                n2712 = Concatenate Strings("Bus 2 write: " ("string"), "Serial polling handler 2") -> (w2110:string)
                                n2713 = local write "GPIB bus 2 traffic"(w2110) -> ()
                                }
                                frame #1 {
                                n2714 = local read "VISA bus 2 resource name out hid"() -> (w2116:refnum<visa-resource-name>)
                                n2715 = local read "VISA bus 2 error out hid"() -> (w2117:errorcluster)
                                n2716 = VISA Read STB(8:w2117, 11:w2116) -> (0:w2118:errorcluster, 2:w2114:u16)  [unwired: 1 out]
                                n2717 = Unbundle By Name(w2118) -> ("status"=w2115:bool)
                                n2718 = Equal?(x=u16 65, y=w2114) -> (x = y?=w2112:bool)
                                n2719 = case shown="True" w2112 {
                                frame False {
                                n2720 = flat-sequence {
                                frame #0 {
                                n2721 = Wait (ms)(milliseconds to wait=u32 5) -> ()  [unwired: 1 out]
                                }
                                frame #1 {
                                n2722 = local write "NS6040 tester states H2 hid"(SC_NS6040_tester_states_v2."serial polling handler" ("NS6040 tester states H1 hid")) -> ()
                                }
                                }
                                }
                                frame True {
                                n2723 = flat-sequence {
                                frame #0 {
                                n2724 = local write "H2 Waiting"(TRUE ("H2 Waiting")) -> ()
                                n2725 = local write "H2 Indexing"(FALSE ("h1 indexing")) -> ()
                                n2726 = local write "H2 Ready with sites hid"(TRUE ("H2 Waiting")) -> ()
                                n2727 = local write "H2 Testing"(FALSE ("h1 indexing")) -> ()
                                }
                                frame #1 {
                                n2728 = Tick Count (ms)() -> (millisecond timer value=w2125:u32)
                                n2729 = Tick Count (ms)() -> (millisecond timer value=w2126:u32)
                                n2730 = local write "H2 it end hidden"(w2125) -> ()
                                n2731 = local write "H2 wt start hidden"(w2126) -> ()
                                }
                                frame #2 {
                                n2732 = local read "H2 it start hidden"() -> (w2130:u32)
                                n2733 = local read "H2 it end hidden"() -> (w2131:u32)
                                n2734 = Subtract(x=w2131, y=w2130) -> (x-y=w2127:u32)
                                n2735 = Divide(x=w2127, y=u32 1000) -> (x/y=w2129:dbl)
                                n2736 = local write "H2 measured  Index Time"(w2129) -> ()
                                }
                                frame #3 {
                                n2737 = local write "NS6040 tester states H1 hid"(SC_NS6040_tester_states_v2."sending Fullsites?" ("NS6040 tester states H1 hid")) -> ()
                                }
                                }
                                }
                                }
                                n2738 = local write "GPIB bus 2 write error"(w2115) -> ()
                                }
                                }
                                }
                                frame "sending Fullsites?" {
                                n2739 = flat-sequence {
                                tunnel: [w2144] -> w2136
                                tunnel: [w2143] -> w2135
                                tunnel: [w2148] -> w2134
                                tunnel: w2135 -> [w2149]
                                tunnel: w2136 -> [w2150]
                                tunnel: w2134 -> [w2166]
                                tunnel: [w2166] -> w2133
                                tunnel: w2133 -> [w2167]
                                frame #0 {
                                w2142 = "Fulllsites?\n"
                                n2740 = local read "VISA bus 2 resource name out hid"() -> (w2145:refnum<visa-resource-name>)
                                n2741 = local read "VISA bus 2 error out hid"() -> (w2146:errorcluster)
                                n2742 = local read "GPIB bus 2 traffic"() -> (w2141:string)
                                n2743 = call <vilib>:"Trim Whitespace.vi"("string"=w2142) -> ("trimmed string"=w2137:string)  [unwired: 1 in]
                                n2744 = VISA Write(VISA resource name=w2145, write buffer=w2142, error in (no error)=w2146) -> (VISA resource name out=w2144:refnum<visa-resource-name>, error out=w2143:errorcluster)  [unwired: 1 out]
                                n2745 = local write "GPIB bus 2 traffic"(w2137) -> ()
                                n2746 = Unbundle By Name(w2143) -> ("status"=w2147:bool)
                                n2747 = Concatenate Strings(w2141, "\r\n", "Bus 2 write: " ("string"), w2137) -> (w2138:string)
                                n2748 = local write "GPIB bus 2 write error"(w2147) -> ()
                                n2749 = local write "GPIB bus 2 traffic"(w2138) -> ()
                                }
                                frame #1 {
                                n2750 = while {
                                tunnel: w2150 -> [w2159]
                                tunnel: w2149 -> [w2158]
                                tunnel: [w2154] -> w2148
                                stop <- w2151 stop-if-true
                                n2751 = local read "GPIB bus 2 traffic"() -> (w2164:string)
                                n2752 = VISA Read(VISA resource name=w2159, byte count=u32 128, error in (no error)=w2158) -> (read buffer=w2154:string, error out=w2156:errorcluster)  [unwired: 2 out]
                                n2753 = Unbundle By Name(w2156) -> ("status"=w2165:bool)
                                n2754 = call <vilib>:"Trim Whitespace.vi"("string"=w2154) -> ("trimmed string"=w2157:string)  [unwired: 1 in]
                                n2755 = Match True/False String(2:"X" ("false string"), 3:"Fullsites" ("true string"), 4:w2154) -> (0:w2151:bool)  [unwired: 1 out]
                                n2756 = local write "GPIB bus 2 read error"(w2165) -> ()
                                n2757 = Concatenate Strings(w2164, "\r\n", "Bus 2 read: " ("string"), w2157) -> (w2163:string)
                                n2758 = local write "GPIB bus 2 traffic"(w2163) -> ()
                                n2759 = Wait (ms)(milliseconds to wait=u32 5) -> ()  [unwired: 1 out]
                                }
                                }
                                frame #2 {
                                n2760 = local write "H2 FULLSITES? response hid"(w2166) -> ()
                                }
                                frame #3 {
                                w2169 = "%032b"  # format string
                                n2761 = call <vilib>:"Space Constant.vi"() -> ("String"=w2174:string)
                                n2762 = Concatenate Strings("Fullsites" ("regular expression"), w2174) -> (w2175:string)
                                n2763 = Match Pattern(string=w2167, regular expression=w2175) -> (after substring=w2171:string)  [unwired: 1 in, 3 out]
                                n2764 = Hexadecimal String To Number(string=w2171, default (0uL)=u64 0 ("default (0 U32)")) -> (number=w2168:u64)  [unwired: 1 in, 1 out]
                                n2765 = Format Into String "Format Into String"(format string=w2169, w2168) -> (resulting string=w2172:string)  [unwired: 2 in, 1 out]
                                n2766 = local write "H2 FULLSITES? binary hid"(w2172) -> ()
                                }
                                frame #4 {
                                n2767 = while {
                                stop <- w2176 stop-if-true
                                n2768 = local read "H2 Lock"() -> (w2176:bool)
                                n2769 = Wait (ms)(milliseconds to wait=u32 5) -> ()  [unwired: 1 out]
                                }
                                }
                                frame #5 {
                                n2770 = local write "NS6040 tester states H2 hid"(SC_NS6040_tester_states_v2."testing" ("NS6040 tester states H1 hid")) -> ()
                                }
                                }
                                }
                                frame "testing" {
                                n2771 = flat-sequence {
                                frame #0 {
                                n2772 = local read "GPIB bus 2 traffic"() -> (w2182:string)
                                n2773 = Concatenate Strings(w2182, "\r\n", "Bus 2: " ("string"), "testing" ("string")) -> (w2180:string)
                                n2774 = local write "GPIB bus 2 traffic"(w2180) -> ()
                                }
                                frame #1 {
                                n2775 = Tick Count (ms)() -> (millisecond timer value=w2187:u32)
                                n2776 = Tick Count (ms)() -> (millisecond timer value=w2188:u32)
                                n2777 = local write "H2 tt start hidden"(w2187) -> ()
                                n2778 = local write "H2 wt end hidden"(w2188) -> ()
                                n2779 = local write "H2 Indexing"(FALSE ("waiting")) -> ()
                                n2780 = local write "H2 Testing"(TRUE ("testing")) -> ()
                                n2781 = local write "H2 Waiting"(FALSE ("waiting")) -> ()
                                }
                                frame #2 {
                                n2782 = local read "H2 wt start hidden"() -> (w2190:u32)
                                n2783 = local read "H2 wt end hidden"() -> (w2189:u32)
                                n2784 = Subtract(x=w2189, y=w2190) -> (x-y=w2193:u32)
                                n2785 = Divide(x=w2193, y=u32 1000) -> (x/y=w2191:dbl)
                                n2786 = local write "H2 measured Wait Time"(w2191) -> ()
                                }
                                frame #3 {
                                n2787 = while {
                                stop <- w2195 continue-if-true
                                n2788 = local read "H2 Lock"() -> (w2195:bool)
                                n2789 = Wait (ms)(milliseconds to wait=u32 1) -> ()  [unwired: 1 out]
                                }
                                }
                                frame #4 {
                                n2790 = local write "H2 Ready with sites hid"(FALSE ("H2 Waiting")) -> ()
                                n2791 = local write "NS6040 tester states H2 hid"(SC_NS6040_tester_states_v2."binning" ("NS6040 tester states H1 hid")) -> ()
                                }
                                }
                                }
                                frame "binning" {
                                n2792 = flat-sequence {
                                frame #0 {
                                n2793 = Tick Count (ms)() -> (millisecond timer value=w2199:u32)
                                n2794 = Tick Count (ms)() -> (millisecond timer value=w2198:u32)
                                n2795 = local write "H2 it start hidden"(w2199) -> ()
                                n2796 = local write "H2 tt end hidden"(w2198) -> ()
                                }
                                frame #1 {
                                n2797 = local read "GPIB bus 2 traffic"() -> (w2201:string)
                                n2798 = Concatenate Strings(w2201, "\r\n", "Bus2: " ("string"), "binning" ("string")) -> (w2203:string)
                                n2799 = local write "GPIB bus 2 traffic"(w2203) -> ()
                                }
                                frame #2 {
                                n2800 = local write "H2 Waiting"(FALSE ("waiting")) -> ()
                                n2801 = local write "H2 Indexing"(TRUE ("waiting")) -> ()
                                n2802 = local write "H2 Testing"(FALSE ("testing")) -> ()
                                }
                                frame #3 {
                                n2803 = local read "H2 tt start hidden"() -> (w2208:u32)
                                n2804 = local read "H2 tt end hidden"() -> (w2209:u32)
                                n2805 = Subtract(x=w2209, y=w2208) -> (x-y=w2211:u32)
                                n2806 = Divide(x=w2211, y=u32 1000) -> (x/y=w2210:dbl)
                                n2807 = local write "H2 measured Test Time"(w2210) -> ()
                                }
                                frame #4 {
                                n2808 = local read "H2 binning string hid"() -> (w2219:string)
                                n2809 = local read "H2 FULLSITES? binary hid"() -> (w2218:string)
                                n2810 = String Subset(string=w2219, offset (0)=6, length (rest)=35 ("length (rest)")) -> (substring=w2225:string)
                                n2811 = local read "H2 Device Count"() -> (w2216:u32)
                                n2812 = local read "H2 Good Units"() -> (w2217:u32)
                                n2813 = Search and Replace String(replace all?=TRUE ("replace all? (F)"), input string=w2225, search string=",") -> (result string=w2231:string)  [unwired: 5 in, 3 out]
                                n2814 = Search and Replace String(replace all?=TRUE ("replace all? (F)"), input string=w2218, search string="1") -> (number of replacements=w2222:i32)  [unwired: 5 in, 3 out]
                                n2815 = Add(x=w2222, y=w2216) -> (x+y=w2214:u32)
                                n2816 = Divide(x=w2217, y=w2216) -> (x/y=w2232:dbl)
                                n2817 = Search and Replace String(replace all?=TRUE ("replace all? (F)"), input string=w2231, search string="1") -> (number of replacements=w2230:i32)  [unwired: 5 in, 3 out]
                                n2818 = local write "H2 Device Count"(w2214) -> ()
                                n2819 = Add(x=w2230, y=w2217) -> (x+y=w2215:u32)
                                n2820 = Multiply(x=w2232, y=100.0) -> (x*y=w2213:dbl)
                                n2821 = local write "H2 Good Units"(w2215) -> ()
                                n2822 = local write "H2 cycle yield hid"(w2213) -> ()
                                }
                                frame #5 {
                                n2823 = local read "H2 Device Count"() -> (w2234:u32)
                                n2824 = local read "H2 Good Units"() -> (w2235:u32)
                                n2825 = Divide(x=w2235, y=w2234) -> (x/y=w2237:dbl)
                                n2826 = Multiply(x=w2237, y=100.0) -> (x*y=w2236:dbl)
                                n2827 = local write "H2 lot yield mon"(w2236) -> ()
                                }
                                frame #6 {
                                n2828 = local read "H2 online"() -> (w2239:bool)
                                n2829 = local read "POWER"() -> (w2240:bool)
                                n2830 = Compound Arithmetic op=AND(w2239, w2240) -> (w2241:bool)
                                n2831 = case shown="True" w2241 {
                                frame False {
                                n2832 = local write "NS6040 tester states H2 hid"(SC_NS6040_tester_states_v2."closing bus" ("NS6040 tester states H1 hid")) -> ()
                                }
                                frame True {
                                n2833 = local write "NS6040 tester states H2 hid"(SC_NS6040_tester_states_v2."serial polling handler" ("NS6040 tester states H1 hid")) -> ()
                                }
                                }
                                }
                                }
                                }
                                frame "closing bus" {
                                n2834 = local read "GPIB bus 2 traffic"() -> (w2248:string)
                                n2835 = local write "Exit SC tester H2 StMach hid"(TRUE ("Exit H2 state machine hid")) -> ()
                                n2836 = local read "VISA bus 2 resource name out hid"() -> (w2252:refnum<visa-resource-name>)
                                n2837 = local read "VISA bus 2 error out hid"() -> (w2251:errorcluster)
                                n2838 = Concatenate Strings(w2248, "\r\n", "Bus 2: closing " ("string")) -> (w2246:string)
                                n2839 = local write "GPIB bus 2 traffic"(w2246) -> ()
                                n2840 = VISA Close(VISA resource name=w2252, error in (no error)=w2251) -> (error out=w2250:errorcluster)
                                n2841 = Unbundle By Name(w2250) -> ("status"=w2249:bool)
                                n2842 = local write "VISA bus 2 close error"(w2249) -> ()
                                }
                                }
                              }
                              frame #1 {
                                n2843 = local read "Slow for  Diagnostics"() -> (w2253:bool)
                                n2844 = case shown="True" w2253 {
                                frame False {
                                }
                                frame True {
                                n2845 = local read "GPIB wait time (ms)"() -> (w2254:u32)
                                n2846 = Wait (ms)(milliseconds to wait=w2254) -> ()  [unwired: 1 out]
                                }
                                }
                              }
                            }
                            n2847 = local read "Exit SC tester H2 StMach hid"() -> (w2060:bool)
                          }
                        }
                      }
                    }
                  }
                }
              }
              n2848 = local read "POWER"() -> (w1784:bool)
            }
          }
        }
      }
    }
  }
